vi "WVDIAL+HSRL_v1.0.vi"() -> ()   [LabVIEW 2012]
uses:
  C:/Users/H2ODial/Desktop/Shared Telescope WV DIAL Code/Libraries and VIs/PowerMeterCommands.dll
  Shared Telescope WV DIAL Code/Libraries and VIs/PowerMeterCommands.dll
  <vilib>/DAQmx/write.llb/DAQmx Write (Digital 1D Bool NChan 1Samp 1Line).vi
  <vilib>/DAQmx/miscellaneous.llb/DAQmx Fill In Error Info.vi
  <vilib>/Analysis/baseanly.llb/Mean (DBL).vi
  NCAR_DIAL_Labview/AMCS_Data.vi
  Libraries and VIs/Scalar_Data.vi
  <vilib>/Analysis/NI_AALBase.lvlib
  Libraries and VIs/Scalar_Data_2.vi
  Libraries and VIs/Scalar_Data_4.vi
  Libraries and VIs/Scalar_Data_3.vi
  Shared Telescope WV DIAL Code/bristol/CLDevIFace.dll
panel:
  out "FileHour":i32=21
  out "L_Count":i32=110
  out "background start":u32=534
  in  "Tab Control 2":enum32{"WV ND narrow", "WV ND wide"}(tab)=enum."WV ND wide"
  out "CH3 RingBuffer long":dbl[][](array[numeric])
  out "CH3 RingBuffer short":dbl[][](array[numeric])
  in  "?":T1(tab)
  out "NRB":dbl[][](graph) caption="Water Vapor Number Density"
  out "NRB 2":dbl[][](graph)=[[8.546195403591417e-05, 0.0002786584247195617, 0.0006090829121441516, 0.0011319761034550358, 0.001851230597986242, 0.002728257694582937, 0.003911345660657617, 0.005256523923123139, 0.006755425044654347, 0.008624773239187781, 0.010431137424772089, 0.012810234215426972, 0.015461219125224046, 0.018378218122423143, 0.02262031451514306, 0.02605089820013463, 0.03081964356661128, 0.03682776902972898, 0.04268026676965369, 0.050602630116497696, 0.058176055267544644, 0.06723475921094646, 0.07730364345829362, 0.08808311325248737, 0.10065736026541186, 0.1121183154362115, 0.12544132700380667, 0.1403937882704388, 0.15598356743521824, 0.17162511577051548, 0.18383704451264493, 0.19631841080771978, 0.21306952212863126, 0.22940462971855646, 0.24989138834202432, 0.26774391709096734, 0.28205876831659166, 0.3007676629703441, 0.31385204205047934, 0.33124784798609325, 0.3460233664658083, 0.35742760425188724, 0.3712840242876745, 0.3862720129999002, 0.39660375582269164, 0.40886228048361584, 0.4259284482749054, 0.440391338547647, 0.4566153688007287, 0.4717635460870204, 0.48207676553872175, 0.493753539302993, 0.5090591895240185, 0.5215880181755391, 0.533671261112484, 0.5420256236923419, 0.5530630628816117, 0.5689384508857108, 0.5752889942963373, 0.5875716528420664, 0.592552348222891, 0.5957528280323126, 0.60606140770504, 0.6165439786595378, 0.6287172140895222, 0.6342325225753401, 0.6490804275957623, 0.6524026888098357, 0.6569828232279292, 0.6692196293009464, 0.6831169256783645, 0.7013566860408543, 0.7100145647111005, 0.7160208275552816, 0.7118346778912209, 0.7144317674140145, 0.715945061880639, 0.7306883196013171, 0.7500440003241868, 0.7573606050746181, 0.7745392036058618, 0.7785022273472191, 0.7909248267167492, 0.8033782612939826, 0.8064196853129901, 0.8271538851971981, 0.8351575399099239, 0.8402193884447339, 0.8597133023547572, 0.8561064982936589, 0.8578435604795103, 0.8623534075092139, 0.8686671889614341, 0.8749972245828621, 0.8830530111544569, 0.909164243794476, 0.929038588425524, 0.9449513234760007, 0.957156632076746, 0.9643101360557969, 0.9596692122255749, 0.9545213343837654, 0.9805428317543672, 0.995047829667933, 1.029690672956509, 1.0674733507983893, 1.0955154176258788, 1.0951317989017593, 1.0974263194164438, 1.098780680310163, 1.0906771548016176, 1.1034601833969768, 1.1178136858913106, 1.1556491108545341, 1.170838831362434, 1.1937229570289496, 1.2185107373476831, 1.2369111498271113, 1.230561676484705, 1.2587157129408204, 1.258349691897498, 1.2643569689138991, 1.2850901805745287, 1.2890984172153068, 1.3232287209486395, 1.3179922411597433, 1.346817704187534, 1.3538431767650367, 1.3490196035262791, 1.3643175109856942, 1.357084592559015, 1.3735525179493822, 1.3720954670881582, 1.4069720445340057, 1.4377096932385625, 1.4667379965087042, 1.5062619180212748, 1.5283644930102516, 1.5354177107131104, 1.5563292232593602, 1.5684496791162663, 1.5568576568475363, 1.57314160663676, 1.5610280458417751, 1.581140399533629, 1.6296912525594276, 1.6562224982957428, 1.6957700702505019, 1.7149440773996392, 1.703831851733697, 1.7255160535134793, 1.7022433497624612, 1.7088135505273854, 1.7516190350709335, 1.798567492230373, 1.851955758886426, 1.8787729240747968, 1.9302841558592982, 1.9621318228338211, 1.9389378628727318, 1.9419926711108755, 1.9071918724993167, 1.8776863760152394, 1.8809405195258893, 1.9470314446188945, 1.9808515850130741, 2.0199051462386906, 2.111296178876415, 2.1153168527738186, 2.0968436639575736, 2.1412443186872054, 2.0756544478907495, 2.112753082434424, 2.1604416956610515, 2.1560867559085426, 2.239772997249097, 2.228779150280646, 2.263170685701022, 2.2168189161218668, 2.2129567210141583, 2.3490351617776835, 2.3904843802922366, 2.5153269519645782, 2.5634805908928726, 2.458644596909608, 2.4076529388828254, 2.431060203259, 2.487089848092278, 2.5385626161957418, 2.6534834782958736, 2.67324914118592, 2.6381061484328536, 2.659899097123786, 2.5932644861877714, 2.6291824330994853, 2.6989899250386693, 2.7424429265496375, 2.8488106986291943, 2.742279667999013, 2.725931661741348, 2.7773277260306966, 2.7669742901423433, 2.92714329948808, 2.9221494539127484, 2.950868194941447, 2.9730195868417186, 2.925221244719501, 3.0283229684289505, 3.045295843575443, 3.048386749915065, 2.9940537506089977, 2.999786519907248, 3.086225175965684, 3.0832975730831595, 3.1989694437550082, 3.243221406629081, 3.2005292303817927, 3.2510606719442636, 3.3383517491714887, 3.353440000926484, 3.3095989472229785, 3.410836647766328, 3.426518483197781, 3.5544093485967143, 3.796590326585979, 3.9752510583934777, 4.034684936991259, 3.941500910307474, 3.814794509432233, 3.614324384587308, 3.6283979364642334, 3.652682507305726, 3.6082445051935146, 3.757776325324033, 3.76070782445612, 3.8753962858175615, 3.832016308719547, 3.8070673373511394, 3.7482590130421487, 3.7356792789637026, 3.901429537689568, 3.9238044137388224, 3.981219962542532, 3.9581165639389835, 4.0440009093367, 3.9872219706905603, 4.074375676028611, 4.163939562811207, 4.109183162644875, 4.232130532448989, 4.32470565779948, 4.392875665538858, 4.419025834001803, 4.546703907908768, 4.6913520732902265, 5.095435948024424, 5.85033668191871, 6.948416991714669, 8.252360397367092, 9.704975333999297, 11.520408914991561, 13.322242925070737, 15.430932827011324, 17.759334108200914, 20.255853327839965, 23.129199142995606, 26.49310623037815, 30.317223286412915, 34.42247995845735, 38.843862293548, 42.96907001161705, 46.5351507877964, 49.700108765272844, 52.30595052176305, 54.66151784066439, 57.27473702687503, 59.76656578242474, 62.06676901244773, 64.07942162504204, 64.90714855474691, 64.57456805484065, 62.808310955515694, 59.961565043940276, 56.4288091190475, 52.44829418294068, 48.29155132434781, 44.122518735143416, 39.90135070569276, 35.95413315064079, 32.311788313192835, 28.664145828333695, 25.56822655944791, 22.593381127055597, 20.147311147330587, 18.37643667972368, 16.804539565374697, 15.544135239321264, 14.57019798472182, 13.511371779657093, 11.951556131001917, 10.556796376131562, 9.105859206777339, 7.636153114912772, 6.742182672366893, 5.884575550909214, 4.9120517923298905, 4.0816387293604155, 3.4251989306529906, 3.0755115887399, 2.992330865928349, 3.0592839009704034, 3.215509932991261, 3.164313441912157, 3.292078243733256, 3.3277022651481674, 3.4104950488283525, 3.6591380424661044, 3.6585893771087408, 3.645111765748741, 3.6040841077506585, 3.3942281204233713, 3.2723340521646254, 3.3042653495262546, 3.212298565962416, 3.2588896657794293, 3.412172206342532, 3.5365748913881014, 3.666044719857089, 3.6099922967500166, 3.5742002916165814, 3.3243040247393, 3.4802692620899798, 3.6002648864623774, 3.4946730738462572, 3.682551697278211, 3.534498028233769, 3.651838970885956, 3.6592843766152097, 3.5769786317282497, 3.831175889669123, 3.9537359381192307, 4.198205817594047, 4.292762449077934, 4.027917543935257, 3.86627577906732, 3.7390920401381775, 3.908518496471237, 3.9575314327457787, 4.045767179550537, 4.182182167113987, 4.319323821591138, 4.213359494616898, 3.9828552276172653, 3.9029181891931564, 3.8813083181843817, 4.124660793610378, 4.458753325246155, 4.484656167121237, 4.21569603752043, 4.398738645215913, 4.38977125517771, 4.486826719323201, 4.636388575777474, 4.721927541304717, 4.755068674711436, 4.678037042645568, 4.472456631914351, 4.437464950237424, 4.471292420670343, 4.635589244752503, 4.9756894692650535, 5.101888232883755, 5.196663320629597, 5.167081503628507, 4.932632838482907, 4.833721902386821, 4.920578756221176, 4.801799860414645, 4.982886632319263, 4.94287218541304, 4.7477113492626035, 5.053228596215403, 5.178145722278693, 5.251496618227864, 5.308182173096638, 5.126027314472312, 5.13158884387731, 5.245580767640445, 5.466282560232339, 5.520268417359091, 5.484994199187797, 5.440350102291734, 3.941060894744326, 2.540276340539141, 1.0752741992785009, -0.21371654449453512, -0.2535263616787527, -0.0215251722412666, 0.0736960393954925, -0.16074128741361193, -0.22026055992248075, -0.504917541914029, -0.5307574380992427, -0.5418672161900913, -0.5865574400501288, -0.47736616519198566, -0.17759619290122416, 0.025489947610103775, 0.12404732338561399, 0.5072486683987952, 0.1854880266358113, 0.26600693173218026, 0.37269308072518276, -0.06214751635724484, 0.16109730035647882, 0.19961295131033274, 0.16054713331939102, 0.3723968795809794, 0.13049120350027968, -0.17385934990265337, -0.21640202606490286, -0.48491744291793354, -0.3516048206810621, -0.5452074651121137, -0.6640463986814213, -0.5148790831917176, -0.5996424436961612, -0.3675738486958148, -0.24413197824721797, -0.31118451234206884, -0.451177199999366, -0.5872883257360875, -0.35674585539839615, -0.19314012538700928, 0.0021220489657220276, 0.21466183565900696, 0.09269836459999599, 0.17646046148922798, 0.056526565682545306, 0.24408390632204388, 0.07252540455404405, -0.02181420421509619, 0.10205416135256055, -0.09331498102145104, -0.07214578665686074, 0.1846866976108202, 0.5635053691699698, 0.5309428402635872, 0.5350604832036495, 0.5511159858985675, 0.39021559281953083, 0.5019216998108322, 0.8010907973716676, 0.1820967880098238, 0.2516937332550209, 0.13548174860232123, 0.003426436422801223, 0.5498271763579102, 0.3017178427483544, 0.30779490101395435, 0.3194336031664126, 0.14682798732272256, 0.35782941193936996, 0.21703523756214044, 0.1580964681743854, 0.26852071324119886, 0.06585437268575421, 0.25225607116669657, -0.0987900349022226, -0.2865272113485497, -0.23476975121469307, -0.3714731517059426, -0.2623208170135795, -0.9814932822860765, -1.0578589256565503, -0.6479324108525774, -0.5427806071790823, 0.20541712714675675, 0.19515889423177873, -0.29526119720445787, -0.472252091600822, -0.6651737975799542, -0.6186882389312311, -0.369116926064781, -0.3690155725472422, -0.38647936731578586, -0.0950262543059411, -0.03854286960600729, 0.30726911813041896, 0.4651921643385956, 0.6978446374004414, 1.0103301505079703, 1.1579083835337383, 1.3873538039368287, 0.4157864001006136, 0.6469789390673985, 0.5046572410534047, 0.26932256080595396, 0.5819929290496607, -0.026184210530850176, -0.5210278980359441, -0.5218016986678393, -0.09830787683363085, 0.10527780250099723, 0.4203966150447178, 0.43890253055010187, 0.14924195872471907, 0.49017086714906183, 0.7979315186565493, 0.9509911782214592, 1.060490580096141, 0.7547309430188422, 0.5481496744565173, 0.6572918231669737, 0.7080537983862634, 0.32232225319211155, 0.16999017226614138, -0.2027014179632393, -0.6150725603001224, -0.6127660288641613, -0.5963368434638746, -0.6377635713973827, -0.3022504867219528, 0.020185972398814287, 0.1271130821329239, 0.4991850715558948, 0.6693287614761402, 0.32397832728321585, 0.31794176368996296, 0.10669714138882108, -0.03197152766302852, 0.4185465993184435, 0.5081345035389131, 0.11472933106232114, -0.335101659818229, -0.7236369378617327, -1.0696346854599716, -0.7595991284525778, -0.4130296018032728, -0.4655290854617895, -0.1709578789784718, 0.35155527912355344, 0.49114775107992503, 0.670181627376166, 0.7230296930330916, 0.5770818030588206, 0.281430213436321, -0.15202417316952307, -0.5672339141806462, -0.784440563139071, -0.42794760098036877, 0.31191170275899854, 0.8830921349838413, 0.7115149103111856, 0.3440988921429906, 0.0, 0.0, 0.0, 0.0, 0.0]] caption="Water Vapor Number Density"
  out "CH 1 (WV off) counts display":dbl[][](graph) caption="Water Vapor Number Density"
  out "CH 3 (HSRL comb) counts display":dbl[][](graph)=[[105.35999999999967, 41.35999999999967, -21.640000000000327, 29.359999999999673, 89.35999999999967, -127.64000000000033, -119.64000000000033, 47.35999999999967, 53.35999999999967, -15.640000000000327, 82.35999999999967, 114.35999999999967, 141.35999999999967, -22.640000000000327, 130.35999999999967, 185.35999999999967, 154.35999999999967, 75.35999999999967, -42.64000000000033, 5.359999999999673, 129.35999999999967, 243.35999999999967, 192.35999999999967, 97.35999999999967, 206.35999999999967, 154.35999999999967, 301.3599999999997, 341.3599999999997, 187.35999999999967, 197.35999999999967, 384.3599999999997, 184.35999999999967, 331.3599999999997, 200.35999999999967, 183.35999999999967, 294.3599999999997, 307.3599999999997, 439.3599999999997, 415.3599999999997, 322.3599999999997, 367.3599999999997, 213.35999999999967, 366.3599999999997, 322.3599999999997, 197.35999999999967, 229.35999999999967, 264.3599999999997, 295.3599999999997, 196.35999999999967, 156.35999999999967, 205.35999999999967, 277.3599999999997, 294.3599999999997, 374.3599999999997, 277.3599999999997, 287.3599999999997, 132.35999999999967, 356.3599999999997, 275.3599999999997, 290.3599999999997, 272.3599999999997, 144.35999999999967, 185.35999999999967, 197.35999999999967, 246.35999999999967, 226.35999999999967, 185.35999999999967, 297.3599999999997, 214.35999999999967, 153.35999999999967, 159.35999999999967, 218.35999999999967, 42.35999999999967, 137.35999999999967, 88.35999999999967, 100.35999999999967, 96.35999999999967, 161.35999999999967, 102.35999999999967, 162.35999999999967, 23.359999999999673, 151.35999999999967, 171.35999999999967, 188.35999999999967, -84.64000000000033, 31.359999999999673, -26.640000000000327, 74.35999999999967, 93.35999999999967, 41.35999999999967, 17.359999999999673, -6.640000000000327, 148.35999999999967, 159.35999999999967, 33.35999999999967, 75.35999999999967, 50.35999999999967, 132.35999999999967, 43.35999999999967, 32.35999999999967, 52.35999999999967, 100.35999999999967, 1.3599999999996726, -25.640000000000327, -48.64000000000033, 80.35999999999967, -81.64000000000033, -28.640000000000327, -92.64000000000033, 70.35999999999967, 117.35999999999967, -4.640000000000327, 15.359999999999673, 36.35999999999967, 30.359999999999673, 136.35999999999967, 79.35999999999967, 103.35999999999967, 27.359999999999673, -65.64000000000033, 156.35999999999967, -72.64000000000033, 26.359999999999673, 9.359999999999673, -6.640000000000327, -48.64000000000033, 46.35999999999967, 103.35999999999967, 19.359999999999673, 80.35999999999967, -169.64000000000033, 94.35999999999967, 41.35999999999967, -86.64000000000033, -10.640000000000327, -41.64000000000033, 66.35999999999967, 74.35999999999967, 87.35999999999967, -17.640000000000327, -3.6400000000003274, -58.64000000000033, 46.35999999999967, 21.359999999999673, -12.640000000000327, -50.64000000000033, 45.35999999999967, 83.35999999999967, 152.35999999999967, -69.64000000000033, 4.359999999999673, 62.35999999999967, -40.64000000000033, -53.64000000000033, -50.64000000000033, -33.64000000000033, 38.35999999999967, -10.640000000000327, -1.6400000000003274, -7.640000000000327, -4.640000000000327, -59.64000000000033, -49.64000000000033, 60.35999999999967, 34.35999999999967, -143.64000000000033, -104.64000000000033, -59.64000000000033, 2.3599999999996726, -100.64000000000033, -3.6400000000003274, -54.64000000000033, 42.35999999999967, 135.35999999999967, -10.640000000000327, 3.3599999999996726, -6.640000000000327, -79.64000000000033, -117.64000000000033, 42.35999999999967, 90.35999999999967, -73.64000000000033, 161.35999999999967, 79.35999999999967, 41.35999999999967, -52.64000000000033, 61.35999999999967, 9.359999999999673, -10.640000000000327, -164.64000000000033, 103.35999999999967, -89.64000000000033, -32.64000000000033, 31.359999999999673, 41.35999999999967, 42.35999999999967, -68.64000000000033, 58.35999999999967, 8.359999999999673, 28.359999999999673, 37.35999999999967, -19.640000000000327, 39.35999999999967, 49.35999999999967, 9.359999999999673, 73.35999999999967, -105.64000000000033, -9.640000000000327, -171.64000000000033, -56.64000000000033, -17.640000000000327, 64.35999999999967, -50.64000000000033, -115.64000000000033, -48.64000000000033, 110.35999999999967, 79.35999999999967, -127.64000000000033, -117.64000000000033, -70.64000000000033, 46.35999999999967, -88.64000000000033, 65.35999999999967, -31.640000000000327, -32.64000000000033, -81.64000000000033, -12.640000000000327, -6.640000000000327, -25.640000000000327, -163.64000000000033, -7.640000000000327, 1.3599999999996726, -48.64000000000033, 67.35999999999967, -11.640000000000327, -14.640000000000327, 110.35999999999967, -35.64000000000033, 40.35999999999967, -34.64000000000033, -28.640000000000327, 25.359999999999673, -24.640000000000327, 32.35999999999967, 21.359999999999673, 32.35999999999967, -47.64000000000033, -158.64000000000033, -48.64000000000033, -19.640000000000327, 28.359999999999673, -32.64000000000033, 100.35999999999967, 0.3599999999996726, -58.64000000000033, 126.35999999999967, 39.35999999999967, -102.64000000000033, 45.35999999999967, 269.3599999999997, 248.35999999999967, 370.3599999999997, 551.3599999999997, 698.3599999999997, 743.3599999999997, 888.3599999999997, 1103.3599999999997, 1108.3599999999997, 1096.3599999999997, 1212.3599999999997, 1501.3599999999997, 1609.3599999999997, 1851.3599999999997, 1948.3599999999997, 1879.3599999999997, 1926.3599999999997, 1860.3599999999997, 2027.3599999999997, 1776.3599999999997, 1865.3599999999997, 1711.3599999999997, 1508.3599999999997, 1453.3599999999997, 1241.3599999999997, 1175.3599999999997, 1037.3599999999997, 924.3599999999997, 842.3599999999997, 875.3599999999997, 788.3599999999997, 727.3599999999997, 587.3599999999997, 441.3599999999997, 474.3599999999997, 404.3599999999997, 352.3599999999997, 329.3599999999997, 267.3599999999997, 205.35999999999967, 308.3599999999997, 160.35999999999967, 187.35999999999967, 146.35999999999967, 142.35999999999967, 175.35999999999967, 88.35999999999967, -74.64000000000033, 80.35999999999967, 42.35999999999967, -150.64000000000033, 30.359999999999673, -1.6400000000003274, -68.64000000000033, -65.64000000000033, 23.359999999999673, -22.640000000000327, -42.64000000000033, -84.64000000000033, -35.64000000000033, 64.35999999999967, -91.64000000000033, -36.64000000000033, -47.64000000000033, -135.64000000000033, -22.640000000000327, -123.64000000000033, 65.35999999999967, 50.35999999999967, -64.64000000000033, 13.359999999999673, 80.35999999999967, -85.64000000000033, -167.64000000000033, 13.359999999999673, 13.359999999999673, 82.35999999999967, 5.359999999999673, -0.6400000000003274, 96.35999999999967, -23.640000000000327, 49.35999999999967, -19.640000000000327, 36.35999999999967, 20.359999999999673, -70.64000000000033, -45.64000000000033, -40.64000000000033, -15.640000000000327, 7.359999999999673, -54.64000000000033, 56.35999999999967, 132.35999999999967, -0.6400000000003274, 106.35999999999967, -140.64000000000033, 54.35999999999967, -45.64000000000033, -20.640000000000327, -17.640000000000327, -74.64000000000033, 34.35999999999967, 19.359999999999673, 63.35999999999967, 43.35999999999967, 39.35999999999967, 17.359999999999673, -64.64000000000033, -58.64000000000033, 92.35999999999967, -40.64000000000033, 2.3599999999996726, 67.35999999999967, -34.64000000000033, 78.35999999999967, -14.640000000000327, -74.64000000000033, -30.640000000000327, 115.35999999999967, -34.64000000000033, -0.6400000000003274, -98.64000000000033, -52.64000000000033, -39.64000000000033, 42.35999999999967, 71.35999999999967, -8.640000000000327, 63.35999999999967, 61.35999999999967, -25.640000000000327, -98.64000000000033, -25.640000000000327, 4.359999999999673, 47.35999999999967, 155.35999999999967, 39.35999999999967, 70.35999999999967, -117.64000000000033, -26.640000000000327, -37.64000000000033, 0.3599999999996726, 2.3599999999996726, 109.35999999999967, -105.64000000000033, 88.35999999999967, -19.640000000000327, 51.35999999999967, -24.640000000000327, -84.64000000000033, 16.359999999999673, -44.64000000000033, 65.35999999999967, -39.64000000000033, 82.35999999999967, -63.64000000000033, 30.359999999999673, 36.35999999999967, 53.35999999999967, -33.64000000000033, 87.35999999999967, 131.35999999999967, 18.359999999999673, -67.64000000000033, 13.359999999999673, 67.35999999999967, -17.640000000000327, -1.6400000000003274, -44.64000000000033, 17.359999999999673, -34.64000000000033, -16.640000000000327, 49.35999999999967, 22.359999999999673, 69.35999999999967, -77.64000000000033, -6.640000000000327, 44.35999999999967, -24.640000000000327, 33.35999999999967, 33.35999999999967, -65.64000000000033, 96.35999999999967, -102.64000000000033, 57.35999999999967, 94.35999999999967, -95.64000000000033, -29.640000000000327, -88.64000000000033, -49.64000000000033, 168.35999999999967, -35.64000000000033, 10.359999999999673, -73.64000000000033, -84.64000000000033, -99.64000000000033, -39.64000000000033, -109.64000000000033, -51.64000000000033, 10.359999999999673, 52.35999999999967, -49.64000000000033, 10.359999999999673, -51.64000000000033, -6.640000000000327, 45.35999999999967, 60.35999999999967, -24.640000000000327, 29.359999999999673, 78.35999999999967, 4.359999999999673, 132.35999999999967, 13.359999999999673, -92.64000000000033, -52.64000000000033, 58.35999999999967, 30.359999999999673, -60.64000000000033, -135.64000000000033, 63.35999999999967, 8.359999999999673, 56.35999999999967, -60.64000000000033, 10.359999999999673, 30.359999999999673, -73.64000000000033, -37.64000000000033, 53.35999999999967, -18.640000000000327, -28.640000000000327, 52.35999999999967, 137.35999999999967, 53.35999999999967, 44.35999999999967, 96.35999999999967, 65.35999999999967, -82.64000000000033, -126.64000000000033, 10.359999999999673, -11.640000000000327, 21.359999999999673, 22.359999999999673, 51.35999999999967, -16.640000000000327, 51.35999999999967, 11.359999999999673, -53.64000000000033, 107.35999999999967, 109.35999999999967, -7.640000000000327, -50.64000000000033, -91.64000000000033, 40.35999999999967, 11.359999999999673, -44.64000000000033, 25.359999999999673, 80.35999999999967, 52.35999999999967, 88.35999999999967, 36.35999999999967, 89.35999999999967, 37.35999999999967, -136.64000000000033, 29.359999999999673, 57.35999999999967, 111.35999999999967, -102.64000000000033, 60.35999999999967, -92.64000000000033, 12.359999999999673, -63.64000000000033, 34.35999999999967, -151.64000000000033, -0.6400000000003274, 40.35999999999967, 142.35999999999967, 72.35999999999967, 40.35999999999967, 65.35999999999967, 29.359999999999673, -178.64000000000033, -44.64000000000033, -2.6400000000003274, 36.35999999999967, 20.359999999999673, -24.640000000000327, 34.35999999999967, -46.64000000000033, 0.3599999999996726, -38.64000000000033, -34.64000000000033, 10.359999999999673, 105.35999999999967, -24.640000000000327, 46.35999999999967, 59.35999999999967, -81.64000000000033, 51.35999999999967, -115.64000000000033, 16.359999999999673, 4.359999999999673, 0.0]] caption="Water Vapor Number Density"
  out "CH3 (HSRL combined) smooth S":dbl[](array[numeric])=[205.29783333333336, 167.4186666666667, 162.64783333333338, 170.01866666666672, 177.9353333333334, 182.0978333333334, 191.7811666666667, 197.3186666666667, 200.35616666666672, 207.1811666666667, 207.08533333333338, 213.6811666666667, 219.73533333333336, 225.1978333333334, 241.41033333333337, 244.34783333333334, 256.03533333333337, 272.84783333333337, 283.7645, 303.5686666666667, 316.51033333333334, 333.2353333333333, 350.4811666666666, 366.7019999999999, 386.11449999999996, 397.58116666666666, 412.4186666666667, 429.1186666666667, 444.3811666666667, 456.827, 458.2644999999999, 459.26449999999994, 468.65199999999993, 475.3019999999999, 488.5144999999999, 494.7061666666666, 493.37283333333323, 498.74366666666657, 494.11866666666657, 495.7478333333333, 492.92283333333324, 485.2519999999999, 480.9144999999999, 477.86033333333324, 469.12283333333323, 462.85616666666664, 461.88116666666656, 457.8936666666666, 455.5936666666666, 452.08533333333327, 444.0686666666667, 437.53116666666665, 434.24783333333335, 428.6353333333334, 422.7895000000001, 414.24783333333335, 408.0103333333334, 405.3853333333334, 396.17283333333336, 391.27699999999993, 381.802, 371.62283333333335, 366.16866666666664, 360.97283333333337, 356.87699999999995, 349.2103333333333, 346.8061666666666, 338.4353333333333, 331.03116666666665, 327.6436666666666, 325.102, 324.577, 319.6603333333333, 313.73116666666664, 303.6686666666667, 296.83116666666666, 289.8061666666666, 288.2436666666667, 288.43533333333335, 284.02700000000004, 283.34366666666665, 277.90616666666665, 275.5853333333334, 273.3061666666667, 267.9395, 268.47283333333337, 264.88533333333334, 260.4811666666667, 260.56866666666673, 253.76033333333336, 248.7311666666667, 244.64366666666672, 241.17283333333336, 237.7978333333334, 234.9686666666667, 236.89783333333338, 237.1103333333334, 236.27700000000004, 234.52283333333338, 231.58116666666672, 225.93950000000004, 220.35616666666672, 221.9853333333334, 220.96033333333338, 224.31033333333338, 228.16450000000003, 229.79783333333336, 225.4936666666667, 221.84783333333337, 218.11033333333336, 212.6311666666667, 211.30200000000005, 210.2811666666667, 213.5936666666667, 212.65616666666673, 213.08950000000004, 213.81033333333338, 213.37700000000007, 208.73950000000002, 209.9686666666667, 206.46033333333338, 204.06450000000004, 204.05200000000005, 201.4061666666667, 203.43950000000007, 199.43950000000004, 200.60200000000003, 198.51450000000003, 194.7603333333334, 193.95200000000003, 189.99783333333335, 189.40200000000004, 186.3728333333334, 188.26450000000006, 189.53533333333337, 190.52700000000004, 192.8103333333334, 192.81450000000007, 190.9311666666667, 190.77700000000004, 189.5478333333334, 185.51450000000006, 184.8436666666667, 180.88950000000006, 180.70200000000003, 183.70200000000006, 184.16033333333337, 186.01450000000006, 185.60200000000003, 181.95616666666672, 181.83950000000004, 177.0436666666667, 175.41450000000006, 177.47700000000006, 179.8853333333334, 182.85200000000006, 183.1436666666667, 185.78533333333337, 186.4811666666667, 181.98950000000005, 180.02283333333335, 174.6311666666667, 169.83533333333338, 168.06450000000004, 171.8603333333334, 172.7436666666667, 174.04366666666672, 179.74783333333338, 177.9686666666667, 174.35200000000003, 175.96450000000004, 168.61033333333336, 169.64366666666672, 171.4811666666667, 169.18950000000004, 173.7561666666667, 170.96033333333338, 171.65200000000004, 166.27283333333338, 164.14783333333338, 172.3061666666667, 173.4228333333334, 180.47700000000006, 181.9353333333334, 172.63116666666673, 167.24783333333338, 167.0728333333334, 169.10616666666672, 170.7811666666667, 176.62700000000004, 176.08533333333338, 171.97283333333337, 171.60200000000003, 165.5936666666667, 166.16866666666672, 168.83950000000004, 169.8186666666667, 174.6186666666667, 166.4186666666667, 163.7811666666667, 165.21033333333338, 162.97283333333337, 170.6978333333334, 168.7436666666667, 168.74366666666674, 168.36450000000005, 164.0686666666667, 168.21450000000004, 167.5436666666667, 166.12283333333338, 161.62700000000004, 160.41450000000003, 163.4853333333334, 161.81033333333335, 166.31450000000004, 167.0561666666667, 163.34783333333337, 164.4061666666667, 167.27700000000004, 166.5103333333334, 162.85616666666672, 166.32283333333336, 165.5936666666667, 170.23533333333336, 180.20200000000006, 187.00200000000004, 188.12700000000004, 182.18533333333338, 174.80616666666668, 164.20200000000006, 163.41866666666672, 163.09783333333337, 159.73950000000005, 164.9311666666667, 163.66033333333337, 167.2186666666667, 163.96033333333338, 161.5311666666667, 157.71450000000004, 155.88116666666673, 161.43950000000004, 161.02700000000004, 162.03950000000006, 159.78533333333337, 161.9186666666667, 158.35616666666672, 160.50616666666673, 162.71033333333338, 159.28950000000003, 162.73950000000005, 164.97283333333337, 166.2436666666667, 165.91450000000006, 169.3603333333334, 173.37283333333338, 186.81033333333338, 212.7603333333334, 250.63533333333336, 295.2311666666667, 344.34783333333337, 405.3645, 464.8895, 533.9811666666666, 609.4019999999999, 689.2269999999999, 780.3061666666665, 886.0769999999999, 1005.1020000000001, 1131.156166666667, 1265.131166666667, 1387.2978333333338, 1489.7103333333337, 1577.847833333334, 1647.206166666667, 1707.7395000000006, 1775.106166666667, 1837.7020000000005, 1893.543666666667, 1939.9520000000005, 1950.7645000000002, 1927.4811666666671, 1862.8311666666668, 1767.7270000000008, 1653.9770000000003, 1528.6645000000005, 1399.6895000000004, 1271.7603333333336, 1143.7395000000004, 1024.8228333333336, 915.7645, 807.7728333333333, 716.3228333333333, 629.2686666666666, 557.7686666666666, 505.58949999999993, 459.4561666666666, 422.3103333333333, 393.3228333333333, 362.427, 318.6061666666667, 279.677, 239.74783333333335, 199.81450000000007, 175.3103333333334, 152.0478333333334, 126.12700000000005, 104.1478333333334, 86.8478333333334, 77.48533333333339, 74.90616666666673, 76.08950000000007, 79.4603333333334, 77.69783333333339, 80.31866666666673, 80.6728333333334, 82.15616666666673, 87.5853333333334, 87.02283333333341, 86.1603333333334, 84.6603333333334, 79.23950000000006, 75.92283333333339, 76.18950000000005, 73.61450000000006, 74.22283333333338, 77.23533333333339, 79.56033333333339, 81.96866666666673, 80.22700000000006, 78.95200000000006, 72.99366666666671, 75.95616666666672, 78.10200000000006, 75.3603333333334, 78.93533333333339, 75.31450000000007, 77.35200000000006, 77.05200000000006, 74.87700000000005, 79.7228333333334, 81.78950000000006, 86.33533333333338, 87.76450000000006, 81.87700000000005, 78.13950000000006, 75.13533333333339, 78.08533333333338, 78.61033333333339, 79.90200000000006, 82.1228333333334, 84.33116666666672, 81.79783333333339, 76.88950000000006, 74.92283333333339, 74.08950000000006, 78.28950000000006, 84.15200000000006, 84.16866666666674, 78.6853333333334, 81.64366666666672, 81.02700000000006, 82.36033333333339, 84.63533333333339, 85.7228333333334, 85.85200000000006, 84.00200000000007, 79.87700000000007, 78.82283333333339, 78.99366666666671, 81.45200000000006, 86.95200000000006, 88.67700000000006, 89.83950000000006, 88.85200000000006, 84.3728333333334, 82.24366666666673, 83.27700000000006, 80.83950000000006, 83.44366666666673, 82.33950000000006, 78.67700000000006, 83.29783333333339, 84.9103333333334, 85.66450000000006, 86.13950000000006, 82.75616666666673, 82.41866666666674, 83.81450000000007, 86.88950000000007, 87.2978333333334, 86.2978333333334, 85.1603333333334, 61.39366666666673, 39.381166666666736, 16.589500000000058, -3.281333333333275, -3.8729999999999416, -0.32716666666660776, 1.1145000000000589, -2.4188333333332745, -3.2979999999999414, -7.522999999999941, -7.868833333333274, -7.993833333333274, -8.610499999999941, -6.97299999999994, -2.5813333333332737, 0.36866666666672543, 1.785333333333392, 7.264500000000059, 2.6436666666667255, 3.7728333333333923, 5.260333333333392, -0.872999999999941, 2.2520000000000593, 2.7770000000000588, 2.222833333333392, 5.131166666666726, 1.7895000000000585, -2.3729999999999416, -2.939666666666608, -6.556333333333274, -4.731333333333275, -7.302166666666608, -8.852166666666607, -6.831333333333275, -7.918833333333274, -4.831333333333275, -3.1938333333332745, -4.052166666666608, -5.847999999999941, -7.577166666666608, -4.581333333333275, -2.4688333333332744, 0.02700000000005842, 2.718666666666725, 1.1686666666667254, 2.2145000000000588, 0.7061666666667255, 3.035333333333392, 0.8978333333333921, -0.26883333333327464, 1.2520000000000588, -1.1396666666666078, -0.8771666666666079, 2.2353333333333922, 6.789500000000059, 6.3686666666667255, 6.3895000000000595, 6.552000000000059, 4.6186666666667255, 5.914500000000059, 9.397833333333391, 2.127000000000059, 2.927000000000059, 1.5686666666667257, 0.03950000000005893, 6.310333333333393, 3.447833333333392, 3.502000000000059, 3.6186666666667255, 1.6561666666667256, 4.018666666666726, 2.4270000000000587, 1.7603333333333924, 2.977000000000059, 0.7270000000000585, 2.7728333333333923, -1.0813333333332746, -3.122999999999941, -2.5479999999999414, -4.014666666666608, -2.8229999999999413, -10.518833333333275, -11.289666666666609, -6.885499999999942, -5.743833333333274, 2.164500000000059, 2.0478333333333922, -3.085499999999941, -4.914666666666608, -6.893833333333275, -6.385499999999942, -3.793833333333274, -3.7771666666666075, -3.9396666666666076, -0.964666666666607, -0.389666666666608, 3.0936666666667256, 4.664500000000059, 6.968666666666726, 10.047833333333394, 11.468666666666726, 13.685333333333391, 4.085333333333393, 6.331166666666727, 4.918666666666726, 2.6145000000000596, 5.627000000000059, -0.2521666666666079, -4.997999999999942, -4.985499999999941, -0.9354999999999412, 0.9978333333333924, 3.968666666666725, 4.127000000000059, 1.397833333333392, 4.572833333333392, 7.414500000000059, 8.802000000000058, 9.777000000000058, 6.9311666666667255, 5.014500000000059, 5.989500000000058, 6.427000000000059, 2.914500000000059, 1.5311666666667252, -1.8188333333332745, -5.497999999999941, -5.456333333333274, -5.289666666666609, -5.635499999999942, -2.6604999999999412, 0.17700000000005867, 1.110333333333392, 4.343666666666726, 5.802000000000058, 2.797833333333392, 2.7353333333333922, 0.9145000000000589, -0.2729999999999413, 3.560333333333392, 4.3061666666667255, 0.9686666666667256, -2.8188333333332745, -6.064666666666607, -8.931333333333274, -6.318833333333275, -3.4229999999999414, -3.843833333333275, -1.4063333333332746, 2.8811666666667257, 4.010333333333392, 5.452000000000059, 5.860333333333393, 4.6603333333333925, 2.2645000000000586, -1.2188333333332744, -4.531333333333275, -6.243833333333274, -3.393833333333275, 2.4645000000000583, 6.952000000000059, 5.581166666666725, 2.689500000000059]
  out "CH3 (HSRL combined) smooth L":dbl[](array[numeric])=[66.7708561643836, 29.338493150684968, 27.07393835616442, 32.525993150684975, 36.934383561643884, 40.63815068493156, 46.37873287671238, 48.601335616438405, 53.01743150684937, 59.80595890410964, 64.68438356164387, 71.85047945205483, 77.13900684931511, 82.96606164383564, 90.89414383561648, 98.40869863013702, 107.58078767123291, 118.46948630136993, 127.8898630136987, 139.92496575342471, 150.56965753424666, 164.39328767123294, 178.45150684931514, 191.23318493150688, 206.85390410958908, 219.08250000000004, 230.7408904109589, 241.09020547945207, 249.3325, 255.5533904109589, 261.32821917808224, 265.47547945205486, 271.20578767123294, 274.0191438356165, 276.65184931506855, 279.08678082191784, 279.11332191780826, 281.9241095890411, 280.16469178082195, 277.30253424657536, 274.033698630137, 268.9977397260274, 267.6355821917808, 264.4472260273973, 260.9686301369863, 258.0311301369863, 253.527705479452, 251.86160958904105, 248.24260273972598, 245.44808219178083, 241.65784246575345, 235.7862671232877, 233.76828767123294, 230.248595890411, 224.76229452054798, 224.43010273972607, 218.75715753424657, 214.24517123287674, 211.05938356164387, 204.18523972602742, 199.68095890410962, 194.1544178082192, 189.80510273972604, 185.13986301369866, 182.32565068493153, 178.3222260273973, 176.3984246575343, 174.19808219178088, 170.36417808219187, 168.71691780821925, 165.5439726027398, 163.28455479452063, 158.77342465753435, 154.68695205479463, 148.17496575342474, 143.6424315068494, 139.37530821917815, 135.8453424657535, 133.6758219178083, 129.1176027397261, 127.93095890410969, 124.23660958904118, 121.9523630136987, 120.0011643835617, 116.52941780821922, 114.94722602739729, 111.11845890410962, 108.91811643835618, 106.56794520547948, 103.07821917808222, 100.70921232876715, 97.24174657534249, 93.12616438356167, 89.21263698630139, 87.24602739726029, 85.67582191780824, 87.35904109589043, 88.14500000000002, 85.17924657534249, 84.59106164383564, 79.87273972602742, 77.44808219178086, 77.98832191780825, 76.54397260273977, 77.02684931506855, 75.34106164383566, 73.75202054794524, 72.58934931506853, 71.998595890411, 71.19037671232881, 71.13986301369867, 68.47291095890415, 67.35476027397264, 68.4943150684932, 67.06023972602743, 67.36417808219181, 67.67667808219181, 66.85390410958908, 65.80339041095894, 64.14414383561648, 62.686095890410996, 60.28712328767127, 58.16469178082196, 58.79482876712333, 57.4831849315069, 55.38986301369868, 58.65613013698635, 57.882157534246616, 55.585924657534285, 57.461780821917856, 53.57222602739731, 51.45321917808224, 53.16297945205485, 51.13130136986307, 51.154417808219236, 51.564520547945264, 50.0234246575343, 51.44465753424663, 51.35304794520553, 53.2040753424658, 53.88130136986306, 51.49345890410964, 50.77513698630142, 47.26143835616443, 45.38130136986307, 45.83592465753429, 44.430102739726074, 43.724623287671285, 45.371883561643884, 44.65869863013704, 46.24773972602745, 46.37530821917813, 43.94380136986307, 42.94380136986307, 42.432671232876764, 43.35304794520553, 43.40099315068499, 44.47804794520553, 44.06537671232882, 42.495171232876764, 41.4831849315069, 40.044828767123335, 37.964349315068546, 37.22291095890416, 37.91297945205484, 38.663835616438405, 39.210068493150736, 40.69208904109594, 39.31023972602745, 36.611609589041144, 37.669828767123335, 35.62445205479457, 37.46349315068498, 40.07565068493156, 40.1552739726028, 40.547397260274025, 38.96349315068498, 38.01058219178087, 36.455787671232926, 35.89500000000005, 39.04825342465759, 39.060239726027454, 39.11674657534252, 39.44037671232882, 35.90099315068498, 34.69123287671238, 35.705787671232926, 36.374452054794574, 38.39414383561649, 40.94465753424663, 40.83421232876717, 39.01143835616443, 36.84791095890416, 35.11503424657539, 34.871883561643884, 35.9943150684932, 35.086780821917856, 34.69208904109594, 33.95236301369867, 33.924109589041144, 35.7956849315069, 36.091061643835666, 37.342773972602785, 37.08849315068498, 36.759726027397306, 36.15613013698635, 33.67924657534252, 32.87102739726032, 32.41041095890416, 30.936095890411003, 30.56280821917813, 30.728047945205525, 30.72119863013703, 33.053390410958954, 33.651849315068546, 33.40869863013704, 33.30082191780827, 32.178390410958954, 32.832500000000046, 30.851335616438405, 32.87102739726032, 33.15955479452059, 32.396712328767165, 36.55167808219183, 36.07393835616443, 38.32308219178087, 40.11417808219183, 39.17410958904115, 38.07308219178087, 33.70065068493155, 32.784554794520595, 31.716061643835666, 33.711780821917856, 37.49773972602745, 35.40356164383566, 38.35904109589046, 35.806815068493194, 32.927534246575384, 35.25116438356169, 31.55167808219182, 29.599623287671264, 29.97890410958908, 28.101335616438394, 28.119315068493194, 30.059383561643884, 29.97291095890416, 31.27085616438361, 31.316232876712377, 29.05595890410963, 27.22890410958908, 26.71263698630141, 26.070513698630172, 26.93095890410963, 30.148424657534292, 32.5679452054795, 36.97547945205484, 46.992602739726074, 59.19380136986307, 74.7708561643836, 94.94722602739728, 118.67154109589043, 144.4198287671233, 178.93438356164387, 223.96434931506855, 278.49174657534246, 345.2597260273972, 420.70493150684933, 499.61160958904134, 584.1758219178087, 674.1039041095894, 766.4634931506853, 863.6852397260275, 969.3051027397257, 1072.3342123287666, 1164.0431164383554, 1233.269999999999, 1259.1355821917798, 1249.4515068493142, 1207.254589041095, 1145.3290753424649, 1080.1655479452047, 1020.2074999999993, 977.5722260273967, 950.9472260273968, 931.3076712328764, 906.8787328767121, 869.6535616438355, 811.1167465753423, 738.9583561643835, 662.1176027397261, 580.9309589041097, 506.5217123287673, 441.8316438356166, 387.40955479452066, 350.3547602739727, 327.6869520547947, 315.22034246575356, 311.4806164383563, 304.1501369863015, 289.15527397260286, 269.9215410958905, 241.81109589041108, 212.1895205479453, 185.879589041096, 156.0020205479453, 128.58335616438362, 105.81708904109591, 84.07479452054797, 65.87445205479456, 50.30767123287676, 35.27941780821922, 25.46349315068497, 16.228904109589074, 14.912123287671267, 13.84705479452058, 12.753732876712363, 15.649280821917843, 14.484897260274005, 12.017431506849348, 9.475479452054827, 9.344486301369898, 8.208356164383595, 9.04397260273976, 11.584212328767158, 10.145000000000035, 10.091917808219211, 12.083356164383595, 11.454931506849348, 10.009726027397294, 10.331643835616472, 7.4506506849315395, 7.063664383561678, 10.73147260273976, 9.781130136986334, 10.886438356164417, 9.94551369863017, 9.694657534246609, 9.465205479452088, 9.936952054794554, 10.672397260274007, 9.538835616438389, 11.349623287671266, 11.436095890410991, 12.168116438356197, 12.527705479452088, 11.691232876712363, 12.59534246575346, 9.604760273972637, 9.693801369863047, 10.828219178082225, 12.124452054794553, 13.721198630137017, 13.963493150684965, 12.89842465753428, 11.330787671232912, 13.158698630137021, 13.87702054794524, 13.22633561643839, 12.628732876712364, 13.877876712328803, 13.057671232876746, 14.936095890410991, 15.942945205479486, 16.05339041095894, 16.921541095890447, 17.01143835616442, 16.536267123287708, 15.105616438356197, 14.6681164383562, 13.060239726027433, 14.109897260274007, 14.29397260273976, 14.78455479452058, 16.22547945205483, 15.688664383561678, 15.905273972602775, 15.677534246575377, 14.531130136986336, 14.480616438356197, 14.124452054794554, 12.73232876712332, 13.222910958904142, 12.18438356164387, 11.807671232876745, 12.418116438356197, 12.839349315068528, 13.843630136986338, 14.685239726027433, 15.620171232876746, 15.09106164383565, 14.036267123287704, 12.869315068493185, 7.8992808219178405, 3.123595890410992, 0.18438356164386954, -4.110136986301336, -3.1914726027396925, -0.6640753424657198, -0.32674657534243234, -0.17263698630133661, -3.3370205479451727, -6.456883561643803, -8.483424657534215, -5.7591095890410635, -3.643527397260241, -2.173493150684898, 0.8333561643835955, -1.1794863013698293, -0.06133561643832236, 0.7905479452055131, -2.4842808219177748, -1.0510616438355829, -1.6418150684931172, -2.338732876712295, -0.7514041095890076, -1.9329109589040758, -2.396952054794487, -3.056198630136953, -2.677773972602706, -4.030513698630104, -3.247979452054761, -3.807910958904076, -3.7805136986301036, -2.1383904109588707, -1.115273972602706, 2.1518493150685267, 3.2023630136986636, 2.6912328767123617, 1.4968835616438692, -1.3044863013698296, -2.6289726027396925, -2.843013698630103, -1.3284589041095556, -0.5656164383561307, 1.161267123287705, 1.1878082191781156, 0.5208561643835956, 1.662123287671267, 1.0619520547945545, 2.0782191780822257, 0.1903767123288007, 0.029417808219211472, -0.07589041095887067, -0.29164383561640495, 0.20493150684934858, 0.6912328767123622, 1.910410958904143, 2.171541095890445, 1.473767123287705, 1.0234246575342805, 1.1612671232877056, 1.9172602739726368, 2.937808219178116, 1.3025342465753764, 1.1912328767123626, -0.06989726027393894, 0.20921232876715723, 1.7759931506849655, -0.2890753424657196, 0.0876369863014036, 0.3710273972603077, -0.974006849315035, -0.15465753424654166, -1.2103082191780485, -2.8139041095890076, -2.0904452054794183, -1.3729794520547607, -1.8627054794520213, -1.6529452054794183, -2.1135616438355824, -3.7685273972602404, -4.403801369862981, -2.628972602739693, -4.08017123287668, -2.6897602739725697, -0.07760273972599402, -1.1760616438355829, 1.3196575342466093, 0.38301369863017093, -2.031369863013665, -2.242842465753391, -4.480856164383528, -4.895239726027364, -3.051061643835583, -2.14866438356161, 0.8907191780822254, 0.5491095890411294, -2.574178082191748, -4.240273972602707, -5.87811643835613, -4.229999999999966, -0.46373287671229524, 1.103047945205513, 3.419828767123321, 3.5268493150685263, 3.1586986301370192, 4.286267123287704, 2.737465753424691, 1.3718835616438694, 0.9395205479452395, -1.4346232876711988, -1.338732876712295, -0.7265753424657195, -0.3353082191780485, 0.5414041095890747, -0.59643835616435, -1.0964383561643503, 0.18267123287674591, 1.0208561643835954, 1.939520547945239, 2.2211986301370197, 2.206643835616472, 1.4489383561644174, -0.21458904109585664, 0.9283904109589378, -0.15722602739722696, 0.5713698630137318, 2.296541095890444, 0.3932876712329102, -1.8335958904109253, -2.238561643835583, -2.032226027397227, -2.8395890410958575, 0.47890410958907437, 0.9301027397260607, 0.09619863013701963, 2.7143493150685263, 0.2374657534246909, 0.24431506849318407, -0.02452054794517189, 1.1390068493151024, 1.5328424657534587, 0.9703424657534588, -0.06047945205476002, -0.4688698630136645, 0.6972260273972943, -0.07417808219174693, 2.286267123287705, 0.7006506849315404, -1.4157876712328432, -1.2556849315068161, -1.8472945205479117, -2.437191780821885, 1.9566438356164717, 0.13386986301373227, 1.902705479452088, 2.1278767123288005, -0.6880479452054457, 2.6980821917808555, -0.7942123287670896, -0.15465753424654183, 0.32136986301373216, -0.20003424657530883, 1.41897260273976, 0.20664383561647215]
  out "CH3 Bin Readings":dbl[](array[numeric])=[5120.0, 5056.0, 4993.0, 5044.0, 5104.0, 4887.0, 4895.0, 5062.0, 5068.0, 4999.0, 5097.0, 5129.0, 5156.0, 4992.0, 5145.0, 5200.0, 5169.0, 5090.0, 4972.0, 5020.0, 5144.0, 5258.0, 5207.0, 5112.0, 5221.0, 5169.0, 5316.0, 5356.0, 5202.0, 5212.0, 5399.0, 5199.0, 5346.0, 5215.0, 5198.0, 5309.0, 5322.0, 5454.0, 5430.0, 5337.0, 5382.0, 5228.0, 5381.0, 5337.0, 5212.0, 5244.0, 5279.0, 5310.0, 5211.0, 5171.0, 5220.0, 5292.0, 5309.0, 5389.0, 5292.0, 5302.0, 5147.0, 5371.0, 5290.0, 5305.0, 5287.0, 5159.0, 5200.0, 5212.0, 5261.0, 5241.0, 5200.0, 5312.0, 5229.0, 5168.0, 5174.0, 5233.0, 5057.0, 5152.0, 5103.0, 5115.0, 5111.0, 5176.0, 5117.0, 5177.0, 5038.0, 5166.0, 5186.0, 5203.0, 4930.0, 5046.0, 4988.0, 5089.0, 5108.0, 5056.0, 5032.0, 5008.0, 5163.0, 5174.0, 5048.0, 5090.0, 5065.0, 5147.0, 5058.0, 5047.0, 5067.0, 5115.0, 5016.0, 4989.0, 4966.0, 5095.0, 4933.0, 4986.0, 4922.0, 5085.0, 5132.0, 5010.0, 5030.0, 5051.0, 5045.0, 5151.0, 5094.0, 5118.0, 5042.0, 4949.0, 5171.0, 4942.0, 5041.0, 5024.0, 5008.0, 4966.0, 5061.0, 5118.0, 5034.0, 5095.0, 4845.0, 5109.0, 5056.0, 4928.0, 5004.0, 4973.0, 5081.0, 5089.0, 5102.0, 4997.0, 5011.0, 4956.0, 5061.0, 5036.0, 5002.0, 4964.0, 5060.0, 5098.0, 5167.0, 4945.0, 5019.0, 5077.0, 4974.0, 4961.0, 4964.0, 4981.0, 5053.0, 5004.0, 5013.0, 5007.0, 5010.0, 4955.0, 4965.0, 5075.0, 5049.0, 4871.0, 4910.0, 4955.0, 5017.0, 4914.0, 5011.0, 4960.0, 5057.0, 5150.0, 5004.0, 5018.0, 5008.0, 4935.0, 4897.0, 5057.0, 5105.0, 4941.0, 5176.0, 5094.0, 5056.0, 4962.0, 5076.0, 5024.0, 5004.0, 4850.0, 5118.0, 4925.0, 4982.0, 5046.0, 5056.0, 5057.0, 4946.0, 5073.0, 5023.0, 5043.0, 5052.0, 4995.0, 5054.0, 5064.0, 5024.0, 5088.0, 4909.0, 5005.0, 4843.0, 4958.0, 4997.0, 5079.0, 4964.0, 4899.0, 4966.0, 5125.0, 5094.0, 4887.0, 4897.0, 4944.0, 5061.0, 4926.0, 5080.0, 4983.0, 4982.0, 4933.0, 5002.0, 5008.0, 4989.0, 4851.0, 5007.0, 5016.0, 4966.0, 5082.0, 5003.0, 5000.0, 5125.0, 4979.0, 5055.0, 4980.0, 4986.0, 5040.0, 4990.0, 5047.0, 5036.0, 5047.0, 4967.0, 4856.0, 4966.0, 4995.0, 5043.0, 4982.0, 5115.0, 5015.0, 4956.0, 5141.0, 5054.0, 4912.0, 5060.0, 5284.0, 5263.0, 5385.0, 5566.0, 5713.0, 5758.0, 5903.0, 6118.0, 6123.0, 6111.0, 6227.0, 6516.0, 6624.0, 6866.0, 6963.0, 6894.0, 6941.0, 6875.0, 7042.0, 6791.0, 6880.0, 6726.0, 6523.0, 6468.0, 6256.0, 6190.0, 6052.0, 5939.0, 5857.0, 5890.0, 5803.0, 5742.0, 5602.0, 5456.0, 5489.0, 5419.0, 5367.0, 5344.0, 5282.0, 5220.0, 5323.0, 5175.0, 5202.0, 5161.0, 5157.0, 5190.0, 5103.0, 4940.0, 5095.0, 5057.0, 4864.0, 5045.0, 5013.0, 4946.0, 4949.0, 5038.0, 4992.0, 4972.0, 4930.0, 4979.0, 5079.0, 4923.0, 4978.0, 4967.0, 4879.0, 4992.0, 4891.0, 5080.0, 5065.0, 4950.0, 5028.0, 5095.0, 4929.0, 4847.0, 5028.0, 5028.0, 5097.0, 5020.0, 5014.0, 5111.0, 4991.0, 5064.0, 4995.0, 5051.0, 5035.0, 4944.0, 4969.0, 4974.0, 4999.0, 5022.0, 4960.0, 5071.0, 5147.0, 5014.0, 5121.0, 4874.0, 5069.0, 4969.0, 4994.0, 4997.0, 4940.0, 5049.0, 5034.0, 5078.0, 5058.0, 5054.0, 5032.0, 4950.0, 4956.0, 5107.0, 4974.0, 5017.0, 5082.0, 4980.0, 5093.0, 5000.0, 4940.0, 4984.0, 5130.0, 4980.0, 5014.0, 4916.0, 4962.0, 4975.0, 5057.0, 5086.0, 5006.0, 5078.0, 5076.0, 4989.0, 4916.0, 4989.0, 5019.0, 5062.0, 5170.0, 5054.0, 5085.0, 4897.0, 4988.0, 4977.0, 5015.0, 5017.0, 5124.0, 4909.0, 5103.0, 4995.0, 5066.0, 4990.0, 4930.0, 5031.0, 4970.0, 5080.0, 4975.0, 5097.0, 4951.0, 5045.0, 5051.0, 5068.0, 4981.0, 5102.0, 5146.0, 5033.0, 4947.0, 5028.0, 5082.0, 4997.0, 5013.0, 4970.0, 5032.0, 4980.0, 4998.0, 5064.0, 5037.0, 5084.0, 4937.0, 5008.0, 5059.0, 4990.0, 5048.0, 5048.0, 4949.0, 5111.0, 4912.0, 5072.0, 5109.0, 4919.0, 4985.0, 4926.0, 4965.0, 5183.0, 4979.0, 5025.0, 4941.0, 4930.0, 4915.0, 4975.0, 4905.0, 4963.0, 5025.0, 5067.0, 4965.0, 5025.0, 4963.0, 5008.0, 5060.0, 5075.0, 4990.0, 5044.0, 5093.0, 5019.0, 5147.0, 5028.0, 4922.0, 4962.0, 5073.0, 5045.0, 4954.0, 4879.0, 5078.0, 5023.0, 5071.0, 4954.0, 5025.0, 5045.0, 4941.0, 4977.0, 5068.0, 4996.0, 4986.0, 5067.0, 5152.0, 5068.0, 5059.0, 5111.0, 5080.0, 4932.0, 4888.0, 5025.0, 5003.0, 5036.0, 5037.0, 5066.0, 4998.0, 5066.0, 5026.0, 4961.0, 5122.0, 5124.0, 5007.0, 4964.0, 4923.0, 5055.0, 5026.0, 4970.0, 5040.0, 5095.0, 5067.0, 5103.0, 5051.0, 5104.0, 5052.0, 4878.0, 5044.0, 5072.0, 5126.0, 4912.0, 5075.0, 4922.0, 5027.0, 4951.0, 5049.0, 4863.0, 5014.0, 5055.0, 5157.0, 5087.0, 5055.0, 5080.0, 5044.0, 4836.0, 4970.0, 5012.0, 5051.0, 5035.0, 4990.0, 5049.0, 4968.0, 5015.0, 4976.0, 4980.0, 5025.0, 5120.0, 4990.0, 5061.0, 5074.0, 4933.0, 5066.0, 4899.0, 5031.0, 5019.0]
  out "CH2 (molecular) smoothed":dbl[](array[numeric])=[14.218630136986288, 11.42839041095889, 8.956643835616426, 9.009726027397248, 9.493458904109577, 11.585924657534234, 13.788835616438343, 16.46349315068492, 15.523424657534232, 16.448082191780806, 19.51657534246574, 20.384726027397246, 23.73061643835615, 27.74345890410958, 29.339349315068482, 31.96863013698629, 31.165547945205468, 33.356472602739714, 34.819657534246566, 36.81708904109588, 40.01229452054793, 42.977191780821904, 44.01400684931505, 49.93181506849314, 55.74431506849314, 58.3924315068493, 60.49431506849314, 61.38215753424656, 62.77256849315066, 65.01999999999998, 71.02513698630135, 72.30510273972601, 72.60647260273971, 73.24260273972601, 74.52856164383562, 74.95664383561643, 75.02770547945205, 73.45835616438356, 72.25373287671232, 72.89328767123287, 74.13900684931505, 74.48660958904107, 72.49260273972601, 72.90356164383559, 72.41811643835615, 73.29910958904108, 72.30595890410959, 72.25287671232876, 69.21092465753425, 64.81023972602739, 62.69979452054793, 59.11417808219177, 60.420684931506834, 61.88729452054793, 61.549965753424644, 60.541404109589024, 57.90613013698629, 53.783698630136975, 55.45921232876711, 53.365034246575334, 52.08078767123287, 54.67667808219177, 49.73660958904108, 48.74260273972601, 48.5910616438356, 47.662123287671214, 48.752020547945186, 46.36931506849314, 45.263150684931496, 41.76914383561642, 40.31366438356163, 41.88044520547944, 39.27256849315067, 41.5910616438356, 40.779417808219165, 37.65184931506848, 37.764863013698616, 34.6715410958904, 30.90955479452053, 31.598767123287658, 30.769143835616426, 29.266575342465742, 31.886438356164376, 29.420684931506838, 30.15527397260273, 30.231472602739714, 29.70921232876711, 29.49602739726026, 29.7674315068493, 27.33678082191779, 25.344486301369848, 28.622739726027383, 25.599623287671214, 26.313664383561626, 25.151849315068475, 23.52171232876711, 21.85390410958903, 20.058527397260264, 20.841917808219165, 17.20835616438355, 19.885582191780806, 23.68866438356163, 21.08335616438355, 22.02171232876711, 19.229760273972587, 15.289691780821903, 13.42839041095889, 14.597054794520533, 15.920684931506834, 15.333356164383549, 19.07821917808218, 16.53198630136985, 13.490034246575329, 14.430102739726015, 13.08934931506848, 13.869315068493139, 14.264006849315056, 14.75030821917807, 15.390719178082179, 14.354760273972591, 14.043972602739714, 12.63558219178081, 11.44294520547944, 10.310239726027385, 13.37530821917807, 14.34534246575341, 14.021712328767109, 15.597054794520535, 12.560239726027383, 10.905273972602728, 12.285410958904096, 10.872739726027383, 13.039691780821904, 16.40784246575341, 16.837636986301355, 16.930102739726014, 14.645856164383547, 10.883013698630123, 6.707499999999985, 6.811952054794507, 6.538835616438343, 8.494315068493137, 9.221198630136973, 8.521712328767109, 6.520856164383548, 6.407842465753411, 6.601335616438342, 7.864178082191768, 7.988321917808206, 5.20921232876711, 5.513150684931493, 4.3119520547945065, 5.847910958904095, 3.365034246575328, 3.3693150684931368, 3.690376712328753, 4.893287671232863, 7.982328767123275, 7.728904109589028, 6.840205479452042, 4.673253424657521, 3.4960273972602605, 3.4686301369862886, 3.843630136986288, 6.003732876712316, 7.752876712328753, 8.153561643835603, 8.09962328767122, 6.421541095890397, 5.892431506849302, 6.2426027397260135, 5.7134931506849185, 4.697226027397247, 3.7340410958903973, 4.736609589041082, 7.025136986301356, 7.189520547945192, 8.180102739726014, 5.598767123287658, 4.573082191780809, 5.829075342465741, 6.019999999999987, 4.618458904109576, 3.902705479452042, 4.92839041095889, 4.848767123287658, 7.946369863013686, 8.708356164383549, 7.4027054794520435, 5.949794520547933, 3.791404109589028, 2.8581849315068366, 3.028561643835604, 3.848767123287659, 5.877876712328755, 5.857328767123275, 5.506301369863001, 7.442945205479438, 8.8924315068493, 6.974623287671219, 7.269999999999985, 4.335068493150671, 2.9258219178082054, 3.8333561643835483, 0.727191780821905, -0.15037671232878025, 0.19808219178080888, 0.20407534246573988, 2.140719178082178, 1.996883561643822, -0.30448630136987614, 0.9232534246575212, 1.2845547945205351, 4.597054794520536, 4.487465753424646, 4.565376712328755, 2.6621232876712204, 2.0080136986301236, 2.3727397260273837, 0.36760273972601387, 4.706643835616425, 4.693801369863001, 3.4249657534246447, 4.436095890410947, 1.8470547945205351, -0.3318835616438487, 1.4386643835616304, 2.958356164383548, 5.886438356164369, 6.665547945205465, 5.4215410958903965, 4.222910958904096, 0.7896917808219047, 0.8530479452054662, 0.666404109589028, -1.3695547945205613, -2.2359931506849446, -3.177773972602753, -0.7214383561643969, 1.4515068493150558, 1.9472260273972475, 2.448938356164371, 1.2400342465753291, 1.54226027397259, 4.585924657534234, 4.6689726027397125, 5.7511643835616315, 5.116746575342453, 4.121027397260262, 5.263150684931494, 5.019999999999987, 5.1467123287671095, 4.369315068493138, 3.685239726027384, 1.666404109589028, -0.04250000000001308, -0.4722945205479586, 0.5705136986301237, 2.408698630136973, 3.8136643835616306, 1.9908904109588914, 1.4711986301369733, 0.9360958904109458, 1.558527397260261, 2.39157534246574, 3.656130136986288, 2.8299315068493023, 2.9086986301369735, 5.058527397260262, 5.598767123287659, 6.0816438356164255, 5.341061643835603, 3.706643835616425, 1.5902054794520417, 2.508013698630124, 2.067089041095877, 1.4172602739725897, 3.746027397260261, 2.880445205479439, 3.8153767123287543, 7.763150684931494, 7.011438356164371, 7.910410958904096, 8.653561643835603, 6.114178082191768, 5.790547945205467, 5.597910958904096, 2.6509931506849185, 2.379589041095877, 0.34619863013697316, -2.937191780821931, 0.2597260273972466, -0.7625342465753562, -0.8926712328767261, 0.9985958904109454, -0.2351369863013828, 1.2126369863013566, 0.2734246575342334, -0.9303424657534374, -2.076746575342478, -3.2925000000000124, 0.06366438356163107, 0.9814726027397127, 1.7768493150684799, 0.5756506849314933, -0.3087671232876843, 1.000308219178069, 3.0105821917808084, 5.983184931506836, 4.986609589041082, 7.660410958904095, 5.507157534246562, 2.9900342465753296, 2.9121232876712195, 0.7229109589040966, 1.5088698630136859, 2.08934931506848, -0.12383561643836871, -2.038219178082204, -1.5099657534246702, 1.1098972602739605, 1.1527054794520417, 1.7040753424657407, 0.9146917808219047, 2.794828767123274, 6.869315068493137, 10.600479452054781, 11.319657534246561, 7.190376712328754, 6.6509931506849185, 2.4908904109588916, 0.6544178082191655, -0.04078767123288907, -1.8601369863013828, -1.4508904109589171, -1.7719520547945335, -1.2214383561643967, 2.781130136986288, 3.5867808219177943, 4.7785616438356024, 6.023424657534234, 4.34448630136985, 3.400993150684919, 1.4754794520547818, 1.4472260273972473, 1.6732534246575215, 3.069657534246563, 4.595342465753411, 3.3444863013698503, 3.3205136986301245, 2.0003082191780694, 1.4797602739725901, 1.7503082191780694, 1.9086986301369735, 0.5199999999999871, 0.6287328767123154, 0.5824999999999867, -0.05705479452056128, 3.370171232876699, 4.368458904109575, 2.7220547945205347, 0.8470547945205343, 0.3761643835616306, 0.23917808219176806, 3.9095547945205356, 6.769999999999987, 6.811095890410947, 8.136438356164371, 6.65184931506848, 3.3992808219177943, 0.11674657534245236, 0.06623287671231548, 0.31109589041094576, 0.7066438356164253, 3.2220547945205347, 3.7931164383561518, 4.0927739726027275, 3.856472602739714, 2.8119520547945083, -1.2068835616438485, -3.6615068493150815, -2.9979794520548078, -2.7967808219178214, 0.06537671232875364, 2.4934589041095756, 2.007157534246562, 2.559383561643822, 1.989178082191768, -1.1264041095890538, 1.786267123287658, 4.14157534246574, 0.9181164383561509, 3.0328424657534114, 0.8984246575342335, 0.052534246575329346, 5.132157534246561, 6.0439726027397125, 7.752020547945191, 7.379589041095877, 5.582499999999987, 5.335068493150673, 2.1655479452054665, 1.9232534246575212, 0.5071575342465624, -0.2496917808219305, 2.0388356164383437, 0.6801027397260146, 3.843630136986289, 7.212636986301357, 3.4489383561643696, 3.1253082191780686, 1.2665753424657393, -1.2659589041096027, 1.239178082191768, 2.8958561643835483, 1.1278767123287536, 0.3838698630136854, -0.5073972602739859, -2.1837671232876836, -0.13924657534247864, -1.102431506849328, 0.21520547945204171, 0.267431506849302, -0.77537671232878, -0.042500000000012694, -0.005684931506862112, 2.3872945205479326, 4.136438356164371, 3.0688013698630012, 2.196369863013686, -0.301917808219191, -1.4389041095890542, 0.7143493150684803, -0.1486643835616568, 1.7160616438356033, 0.09106164383560333, -0.9877054794520678, 1.2015068493150558, 1.0670890410958778, 2.538835616438343, 2.304246575342453, 2.7717123287671095, 1.4215410958903976, 2.430958904109576, 2.5996232876712195, 2.975479452054781, 4.545684931506836, 1.6604109589040954, 4.369315068493137, 3.4857534246575206, -0.24455479452056061, -0.4123630136986429, -2.158938356164396, -1.5425000000000126, -1.7976369863013824, 2.8042465753424524, 1.502876712328754, 1.0636643835616304, 2.722910958904096, 1.5850684931506716, 3.704931506849302, 3.147568493150672, 6.425821917808205, 7.533698630136973, 7.830787671232864, 6.799109589041082, 1.2348972602739585, -1.5810273972602873, -1.2111643835616572, 0.644999999999986, 3.6860958904109453, 3.870171232876699, 3.4814726027397125, 0.31452054794519246, 3.028561643835603, 3.0576712328766993, 2.305958904109576, 5.375308219178069, 2.003732876712316, 4.87102739726026, 6.0063013698629995, 2.4189726027397125, 2.506301369863, 1.3881506849314944, -0.2582534246575464, 3.098767123287659, 4.2289041095890285, 3.9789041095890285, 3.82393835616437, 1.5533904109588907, 3.316232876712315, 4.049965753424644, 6.196369863013685, 10.13643835616437, 10.048253424657519, 6.49688356164382, 5.376164383561629, 1.2888356164383412, -1.3721232876712461, 0.9266780821917681, -1.6332534246575472, -1.7805136986301497, -1.977431506849328, -2.8087671232876845, -2.867842465753438, -0.8823972602739859, -1.0690410958904244, 1.1081849315068357, 1.1886643835616304, -0.2445547945205615, 2.1852397260273837, -0.02109589041097204, 1.673253424657521, 3.7468835616438216, 4.4814726027397125, 3.800821917808206, 5.407842465753411, 3.403561643835604, 1.1253082191780688, 3.1741095890410826, 1.1098972602739596, 3.564520547945193, 5.163835616438343, 5.782842465753411, 6.273424657534234, 7.059383561643822, 6.414691780821904, 3.4232534246575206, 0.2520205479451927, -2.367842465753437, -4.933767123287684, -5.500547945205492, -4.715445205479465, -1.661506849315082, 2.906130136986288, 4.909554794520535, 9.288835616438343, 7.939520547945193, 3.390719178082179, 2.5063013698630012, -0.5519178082191905, -2.166643835616451, -2.896952054794533, -1.8746917808219306, 0.6158904109588916, 0.29568493150683683, 0.9386643835616311, -1.9740068493150809, -1.9157876712328892, -3.8370205479452184, -2.878972602739739, -3.0493493150685063, -4.896952054794534, -2.0313698630137114, -0.6897602739726155]
  out "CH 2 Bin Readings":dbl[](array[numeric])=[9876.0, 9729.0, 9869.0, 9694.0, 9667.0, 9998.0, 9701.0, 9893.0, 9744.0, 9929.0, 9875.0, 9959.0, 9757.0, 9800.0, 9655.0, 9858.0, 9784.0, 9837.0, 9778.0, 9609.0, 9905.0, 9751.0, 9790.0, 9737.0, 9812.0, 9735.0, 9946.0, 9837.0, 9893.0, 9991.0, 9922.0, 9805.0, 9875.0, 9729.0, 9922.0, 9882.0, 9853.0, 9971.0, 9917.0, 9948.0, 9966.0, 10004.0, 10062.0, 9851.0, 9925.0, 9960.0, 9990.0, 10114.0, 10003.0, 9955.0, 10007.0, 9949.0, 9748.0, 9979.0, 10077.0, 9865.0, 9892.0, 9904.0, 9854.0, 9949.0, 9811.0, 10039.0, 9924.0, 9769.0, 9794.0, 9853.0, 9928.0, 9624.0, 9780.0, 9806.0, 9711.0, 9824.0, 9844.0, 9879.0, 9898.0, 10077.0, 9759.0, 9942.0, 9759.0, 9820.0, 9958.0, 9670.0, 9741.0, 9864.0, 9926.0, 9781.0, 9863.0, 9929.0, 9787.0, 9806.0, 9937.0, 9873.0, 9783.0, 9795.0, 9846.0, 9782.0, 9811.0, 9843.0, 9726.0, 9961.0, 9997.0, 9749.0, 9928.0, 9904.0, 9944.0, 9694.0, 9687.0, 9966.0, 9676.0, 9575.0, 9901.0, 9725.0, 9706.0, 9654.0, 9911.0, 9939.0, 9802.0, 9715.0, 9765.0, 9870.0, 9999.0, 9672.0, 9848.0, 9906.0, 9809.0, 9918.0, 9480.0, 9802.0, 9876.0, 9748.0, 9799.0, 9728.0, 9885.0, 9814.0, 9826.0, 9878.0, 9803.0, 9861.0, 9780.0, 9777.0, 9623.0, 9680.0, 9745.0, 9642.0, 9776.0, 9845.0, 9716.0, 9682.0, 9894.0, 9906.0, 9800.0, 9654.0, 9805.0, 9806.0, 9838.0, 9968.0, 9876.0, 9798.0, 9702.0, 9999.0, 9595.0, 9664.0, 9810.0, 9884.0, 9821.0, 9597.0, 9727.0, 9851.0, 9735.0, 9910.0, 9840.0, 9905.0, 9853.0, 9856.0, 9901.0, 9786.0, 9956.0, 9839.0, 9975.0, 9693.0, 9684.0, 9887.0, 9729.0, 9869.0, 9628.0, 9912.0, 9794.0, 9743.0, 9826.0, 9733.0, 9760.0, 9931.0, 9691.0, 9889.0, 9857.0, 9755.0, 9725.0, 9656.0, 9630.0, 10000.0, 9684.0, 9720.0, 9704.0, 9816.0, 9900.0, 9753.0, 9785.0, 9830.0, 9860.0, 9816.0, 9775.0, 9829.0, 9885.0, 9843.0, 9677.0, 9805.0, 9714.0, 9790.0, 9823.0, 9659.0, 9843.0, 9711.0, 9864.0, 9735.0, 9688.0, 9820.0, 9809.0, 9673.0, 9651.0, 9869.0, 9880.0, 9838.0, 9634.0, 9751.0, 9789.0, 9682.0, 9838.0, 9879.0, 9737.0, 9915.0, 9879.0, 9692.0, 9742.0, 9777.0, 9711.0, 9767.0, 9827.0, 9821.0, 9806.0, 9857.0, 9705.0, 9866.0, 9856.0, 9824.0, 9771.0, 9870.0, 9787.0, 9842.0, 9751.0, 9784.0, 9833.0, 9782.0, 9704.0, 9701.0, 9797.0, 9790.0, 9800.0, 9831.0, 9629.0, 9637.0, 9844.0, 9837.0, 9716.0, 9757.0, 9840.0, 9754.0, 9732.0, 9689.0, 9732.0, 9606.0, 9725.0, 9926.0, 9960.0, 9651.0, 9757.0, 9740.0, 9847.0, 9664.0, 9924.0, 9880.0, 9731.0, 9732.0, 9887.0, 9717.0, 9804.0, 9763.0, 9919.0, 9784.0, 9911.0, 9945.0, 9761.0, 9844.0, 9829.0, 9888.0, 9704.0, 9699.0, 9849.0, 9812.0, 9707.0, 9842.0, 9815.0, 9787.0, 9761.0, 9702.0, 9781.0, 9804.0, 9892.0, 9804.0, 9758.0, 9769.0, 9840.0, 9761.0, 9852.0, 9764.0, 9757.0, 10048.0, 9707.0, 9737.0, 9861.0, 9861.0, 9727.0, 9819.0, 9827.0, 9841.0, 9677.0, 9695.0, 9844.0, 9796.0, 9741.0, 9555.0, 9981.0, 9627.0, 9796.0, 9731.0, 9788.0, 9990.0, 9575.0, 9905.0, 9886.0, 9663.0, 9894.0, 9832.0, 9614.0, 9684.0, 9651.0, 9752.0, 9732.0, 9772.0, 9884.0, 9645.0, 9834.0, 9871.0, 9971.0, 9567.0, 9603.0, 9853.0, 9857.0, 9762.0, 9850.0, 9778.0, 9762.0, 9713.0, 9822.0, 9908.0, 9839.0, 9922.0, 9769.0, 9840.0, 9863.0, 9834.0, 9764.0, 9813.0, 9776.0, 9805.0, 10039.0, 9915.0, 9745.0, 9698.0, 9756.0, 9761.0, 9924.0, 9678.0, 9787.0, 9915.0, 9710.0, 9797.0, 9786.0, 9972.0, 9795.0, 9734.0, 9673.0, 9764.0, 9808.0, 9901.0, 9779.0, 9621.0, 9889.0, 9720.0, 9833.0, 9691.0, 9794.0, 9891.0, 9681.0, 9685.0, 9724.0, 9820.0, 9753.0, 9767.0, 9623.0, 9629.0, 9843.0, 9862.0, 9827.0, 9981.0, 9789.0, 9800.0, 9830.0, 9811.0, 9748.0, 9824.0, 9824.0, 9694.0, 9803.0, 9848.0, 9830.0, 9840.0, 9870.0, 9879.0, 9629.0, 9779.0, 9758.0, 9740.0, 9779.0, 9936.0, 9689.0, 9634.0, 9643.0, 9876.0, 9685.0, 9849.0, 9717.0, 9881.0, 9787.0, 9701.0, 9858.0, 9671.0, 9843.0, 9740.0, 9707.0, 9784.0, 9924.0, 9701.0, 9716.0, 9782.0, 9857.0, 9738.0, 9831.0, 9975.0, 9920.0, 9806.0, 9768.0, 9941.0, 9795.0, 9817.0, 9765.0, 9852.0, 9870.0, 9864.0, 9874.0, 9723.0, 9962.0, 9935.0, 9711.0, 9784.0, 9947.0, 9803.0, 9874.0, 9816.0, 9701.0, 9815.0, 9881.0, 9812.0, 9722.0, 9914.0, 9738.0, 9956.0, 9776.0, 9882.0, 9820.0, 9834.0, 9719.0, 9734.0, 9830.0, 9892.0, 9817.0, 9763.0, 9951.0, 9757.0, 9947.0, 9740.0, 9767.0, 9729.0, 9759.0, 9920.0, 9954.0, 9901.0, 9958.0, 9724.0, 9717.0, 9738.0, 9817.0, 9688.0, 9786.0, 9802.0, 9754.0, 9895.0, 9603.0, 9840.0, 9659.0, 9932.0, 9981.0, 9716.0, 9815.0, 9902.0, 9849.0, 9541.0, 9843.0, 9741.0, 9902.0, 9816.0, 9785.0, 9739.0, 9741.0, 9805.0, 9742.0, 9800.0, 9887.0, 9693.0, 9832.0, 9963.0, 9678.0, 9690.0, 9875.0, 9742.0, 9870.0, 9825.0, 9610.0, 9815.0, 9698.0]
  in  "stop":bool
  in  "Reset Average":bool=TRUE
  in  "Save Data?":bool=TRUE
  in  "Collect Data?":bool=TRUE
  in  "ILX Address":i32=6 min=0 step=1
  in  "Lambda On DBR Current":dbl=171.13999999999868
  in  "Lambda Off DBR Current":dbl=172.9499999999997
  in  "Tab Control":T2(tab)=enum."NRB"
  out "NRB plot":cluster{"Y":dbl[], "Y":dbl[]}[](graph)=[{"Y"=[0.0, 0.0, 0.0, 0.0, 0.0, 0.0, 0.0, 0.0, 0.0, 0.0, 0.0, 0.0, 0.0, 0.0, 0.0, 0.0, 0.0, 0.0, 0.0, 0.0, 0.0, 0.0, 0.0, 0.0, 0.0, 0.0, 0.0, 0.0, 0.0, 0.0, 0.0, 0.0, 0.0, 0.0, 0.0, 0.0, 0.0, 0.0, 0.0, 0.0, 0.0, 0.0, 0.0, 0.0, 0.0, 0.0, 0.0, 0.0, 0.0, 0.0, 0.0, 0.0, 0.0, 0.0, 0.0, 0.0, 0.0, 0.0, 0.0, 0.0, 0.0, 0.0, 0.0, 0.0, 0.0, 0.0, 0.0, 0.0, 0.0, 0.0, 0.0, 0.0, 0.0, 0.0, 0.0, 0.0, 0.0, 0.0, 0.0, 0.0, 0.0, 0.0, 0.0, 0.0, 0.0, 0.0, 0.0, 0.0, 0.0, 0.0, 0.0, 0.0, 0.0, 0.0, 0.0, 0.0, 0.0, 0.0, 0.0, 0.0, 0.0, 0.0, 0.0, 0.0, 0.0, 0.0, 0.0, 0.0, 0.0, 0.0, 0.0, 0.0, 0.0, 0.0, 0.0, 0.0, 0.0, 0.0, 0.0, 0.0, 0.0, 0.0, 0.0, 0.0, 0.0, 0.0, 0.0, 0.0, 0.0, 0.0, 0.0, 0.0, 0.0, 0.0, 0.0, 0.0, 0.0, 0.0, 0.0, 0.0, 0.0, 0.0, 0.0, 0.0, 0.0, 0.0, 0.0, 0.0, 0.0, 0.0, 0.0, 0.0, 0.0, 0.0, 0.0, 0.0, 0.0, 0.0, 0.0, 0.0, 0.0, 0.0, 0.0, 0.0, 0.0, 0.0, 0.0, 0.0, 0.0, 0.0, 0.0, 0.0, 0.0, 0.0, 0.0, 0.0, 0.0, 0.0, 0.0, 0.0, 0.0, 0.0, 0.0, 0.0, 0.0, 0.0, 0.0, 0.0, 0.0, 0.0, 0.0, 0.0, 0.0, 0.0, 0.0, 0.0, 0.0, 0.0, 0.0, 0.0, 0.0, 0.0, 0.0, 0.0, 0.0, 0.0, 0.0, 0.0, 0.0, 0.0, 0.0, 0.0, 0.0, 0.0, 0.0, 0.0, 0.0, 0.0, 0.0, 0.0, 0.0, 0.0, 0.0, 0.0, 0.0, 0.0, 0.0, 0.0, 0.0, 0.0, 0.0, 0.0, 0.0, 0.0, 0.0, 0.0, 0.0, 0.0, 0.0, 0.0, 0.0, 0.0, 0.0, 0.0, 0.0, 0.0, 0.0, 0.0, 0.0, 0.0, 0.0, 0.0, 0.0, 0.0, 0.0, 0.0, 0.0, 0.0, 0.0, 0.0, 0.0, 0.0, 0.0, 0.0, 0.0, 0.0, 0.0, 0.0, 0.0, 0.0, 0.0, 0.0, 0.0, 0.0, 0.0, 0.0, 0.0, 0.0, 0.0, 0.0, 0.0, 0.0, 0.0, 0.0, 0.0, 0.0, 0.0, 0.0, 0.0, 0.0, 0.0, 0.0, 0.0, 0.0, 0.0, 0.0, 0.0, 0.0, 0.0, 0.0, 0.0, 0.0, 0.0, 0.0, 0.0, 0.0, 0.0, 0.0, 0.0, 0.0, 0.0, 0.0, 0.0, 0.0, 0.0, 0.0, 0.0, 0.0, 0.0, 0.0, 0.0, 0.0, 0.0, 0.0, 0.0, 0.0, 0.0, 0.0, 0.0, 0.0, 0.0, 0.0, 0.0, 0.0, 0.0, 0.0, 0.0, 0.0, 0.0, 0.0, 0.0, 0.0, 0.0, 0.0, 0.0, 0.0, 0.0, 0.0, 0.0, 0.0, 0.0, 0.0, 0.0, 0.0, 0.0, 0.0, 0.0, 0.0, 0.0, 0.0, 0.0, 0.0, 0.0, 0.0, 0.0, 0.0, 0.0, 0.0, 0.0, 0.0, 0.0, 0.0, 0.0, 0.0, 0.0, 0.0, 0.0, 0.0, 0.0, 0.0, 0.0, 0.0, 0.0, 0.0, 0.0, 0.0, 0.0, 0.0, 0.0, 0.0, 0.0, 0.0, 0.0, 0.0, 0.0, 0.0, 0.0, 0.0, 0.0, 0.0, 0.0, 0.0, 0.0, 0.0, 0.0, 0.0, 0.0, 0.0, 0.0, 0.0, 0.0, 0.0, 0.0, 0.0, 0.0, 0.0, 0.0, 0.0, 0.0, 0.0, 0.0, 0.0, 0.0, 0.0, 0.0, 0.0, 0.0, 0.0, 0.0, 0.0, 0.0, 0.0, 0.0, 0.0, 0.0, 0.0, 0.0, 0.0, 0.0, 0.0, 0.0, 0.0, 0.0, 0.0, 0.0, 0.0, 0.0, 0.0, 0.0, 0.0, 0.0, 0.0, 0.0, 0.0, 0.0, 0.0, 0.0, 0.0, 0.0, 0.0, 0.0, 0.0, 0.0, 0.0, 0.0, 0.0, 0.0, 0.0, 0.0, 0.0, 0.0, 0.0, 0.0, 0.0, 0.0, 0.0, 0.0, 0.0, 0.0, 0.0, 0.0, 0.0, 0.0, 0.0, 0.0, 0.0, 0.0, 0.0, 0.0, 0.0, 0.0, 0.0, 0.0, 0.0, 0.0, 0.0, 0.0, 0.0, 0.0, 0.0, 0.0, 0.0, 0.0, 0.0, 0.0, 0.0, 0.0, 0.0, 0.0, 0.0, 0.0, 0.0, 0.0, 0.0, 0.0, 0.0, 0.0, 0.0, 0.0, 0.0, 0.0, 0.0, 0.0, 0.0, 0.0, 0.0, 0.0, 0.0, 0.0, 0.0, 0.0, 0.0, 0.0, 0.0, 0.0, 0.0, 0.0, 0.0, 0.0, 0.0, 0.0, 0.0, 0.0, 0.0, 0.0, 0.0, 0.0, 0.0, 0.0, 0.0, 0.0, 0.0, 0.0, 0.0, 0.0], "Y"=[0.0375, 0.075, 0.11249999999999999, 0.15, 0.1875, 0.225, 0.26249999999999996, 0.3, 0.33749999999999997, 0.37499999999999994, 0.4125, 0.44999999999999996, 0.48749999999999993, 0.525, 0.5625, 0.6, 0.6375, 0.6749999999999999, 0.7124999999999999, 0.75, 0.7875, 0.825, 0.8624999999999999, 0.8999999999999999, 0.9374999999999999, 0.975, 1.0125, 1.05, 1.0875000000000001, 1.125, 1.1625, 1.2, 1.2375, 1.2750000000000001, 1.3125, 1.35, 1.3875, 1.425, 1.4625000000000001, 1.5, 1.5375, 1.575, 1.6125, 1.6500000000000001, 1.6875, 1.725, 1.7625, 1.8, 1.8375, 1.875, 1.9125, 1.95, 1.9875, 2.025, 2.0625, 2.1, 2.1375, 2.175, 2.2125, 2.25, 2.2875, 2.325, 2.3625, 2.4, 2.4375, 2.475, 2.5125, 2.55, 2.5875, 2.625, 2.6625, 2.7, 2.7375, 2.775, 2.8125, 2.85, 2.8875, 2.925, 2.9625, 3.0, 3.0375, 3.075, 3.1125, 3.15, 3.1875, 3.225, 3.2625, 3.3, 3.3375, 3.375, 3.4125, 3.45, 3.4875, 3.525, 3.5625, 3.6, 3.6374999999999997, 3.675, 3.7125, 3.75, 3.7875, 3.8249999999999997, 3.8625, 3.9, 3.9375, 3.975, 4.012499999999999, 4.05, 4.0874999999999995, 4.124999999999999, 4.1625, 4.199999999999999, 4.2375, 4.2749999999999995, 4.312499999999999, 4.35, 4.387499999999999, 4.425, 4.4624999999999995, 4.499999999999999, 4.5375, 4.574999999999999, 4.6125, 4.6499999999999995, 4.687499999999999, 4.725, 4.762499999999999, 4.8, 4.8374999999999995, 4.874999999999999, 4.9125, 4.949999999999999, 4.9875, 5.0249999999999995, 5.062499999999999, 5.1, 5.137499999999999, 5.175, 5.2124999999999995, 5.249999999999999, 5.2875, 5.324999999999999, 5.3625, 5.3999999999999995, 5.437499999999999, 5.475, 5.512499999999999, 5.55, 5.5874999999999995, 5.624999999999999, 5.6625, 5.699999999999999, 5.7375, 5.7749999999999995, 5.812499999999999, 5.85, 5.887499999999999, 5.925, 5.9624999999999995, 5.999999999999999, 6.0375, 6.074999999999999, 6.1125, 6.1499999999999995, 6.187499999999999, 6.225, 6.262499999999999, 6.3, 6.3374999999999995, 6.374999999999999, 6.4125, 6.449999999999999, 6.4875, 6.5249999999999995, 6.562499999999999, 6.6, 6.637499999999999, 6.675, 6.7124999999999995, 6.749999999999999, 6.7875, 6.824999999999999, 6.8625, 6.8999999999999995, 6.937499999999999, 6.975, 7.012499999999999, 7.05, 7.0874999999999995, 7.124999999999999, 7.1625, 7.199999999999999, 7.237499999999999, 7.2749999999999995, 7.312499999999999, 7.35, 7.387499999999999, 7.424999999999999, 7.4624999999999995, 7.499999999999999, 7.5375, 7.574999999999999, 7.612499999999999, 7.6499999999999995, 7.687499999999999, 7.725, 7.762499999999999, 7.799999999999999, 7.8374999999999995, 7.874999999999999, 7.9125, 7.949999999999999, 7.987499999999999, 8.025, 8.0625, 8.1, 8.1375, 8.174999999999999, 8.212499999999999, 8.25, 8.2875, 8.325, 8.362499999999999, 8.399999999999999, 8.4375, 8.475, 8.5125, 8.549999999999999, 8.587499999999999, 8.625, 8.6625, 8.7, 8.737499999999999, 8.774999999999999, 8.8125, 8.85, 8.8875, 8.924999999999999, 8.962499999999999, 9.0, 9.0375, 9.075, 9.112499999999999, 9.149999999999999, 9.1875, 9.225, 9.2625, 9.299999999999999, 9.337499999999999, 9.375, 9.4125, 9.45, 9.487499999999999, 9.524999999999999, 9.5625, 9.6, 9.6375, 9.674999999999999, 9.712499999999999, 9.75, 9.7875, 9.825, 9.862499999999999, 9.899999999999999, 9.9375, 9.975, 10.0125, 10.049999999999999, 10.087499999999999, 10.125, 10.1625, 10.2, 10.237499999999999, 10.274999999999999, 10.3125, 10.35, 10.3875, 10.424999999999999, 10.462499999999999, 10.5, 10.5375, 10.575, 10.612499999999999, 10.649999999999999, 10.6875, 10.725, 10.7625, 10.799999999999999, 10.837499999999999, 10.875, 10.9125, 10.95, 10.987499999999999, 11.024999999999999, 11.0625, 11.1, 11.1375, 11.174999999999999, 11.212499999999999, 11.25, 11.2875, 11.325, 11.362499999999999, 11.399999999999999, 11.4375, 11.475, 11.5125, 11.549999999999999, 11.587499999999999, 11.625, 11.6625, 11.7, 11.737499999999999, 11.774999999999999, 11.8125, 11.85, 11.8875, 11.924999999999999, 11.962499999999999, 12.0, 12.0375, 12.075, 12.112499999999999, 12.149999999999999, 12.1875, 12.225, 12.2625, 12.299999999999999, 12.337499999999999, 12.375, 12.4125, 12.45, 12.487499999999999, 12.524999999999999, 12.5625, 12.6, 12.6375, 12.674999999999999, 12.712499999999999, 12.75, 12.7875, 12.825, 12.862499999999999, 12.899999999999999, 12.9375, 12.975, 13.0125, 13.049999999999999, 13.087499999999999, 13.125, 13.1625, 13.2, 13.237499999999999, 13.274999999999999, 13.3125, 13.35, 13.3875, 13.424999999999999, 13.462499999999999, 13.5, 13.5375, 13.575, 13.612499999999999, 13.649999999999999, 13.6875, 13.725, 13.7625, 13.799999999999999, 13.837499999999999, 13.875, 13.9125, 13.95, 13.987499999999999, 14.024999999999999, 14.0625, 14.1, 14.1375, 14.174999999999999, 14.212499999999999, 14.25, 14.2875, 14.325, 14.362499999999999, 14.399999999999999, 14.437499999999998, 14.475, 14.5125, 14.549999999999999, 14.587499999999999, 14.624999999999998, 14.6625, 14.7, 14.737499999999999, 14.774999999999999, 14.812499999999998, 14.85, 14.8875, 14.924999999999999, 14.962499999999999, 14.999999999999998, 15.0375, 15.075, 15.112499999999999, 15.149999999999999, 15.187499999999998, 15.225, 15.2625, 15.299999999999999, 15.337499999999999, 15.374999999999998, 15.4125, 15.45, 15.487499999999999, 15.524999999999999, 15.562499999999998, 15.6, 15.6375, 15.674999999999999, 15.712499999999999, 15.749999999999998, 15.7875, 15.825, 15.862499999999999, 15.899999999999999, 15.937499999999998, 15.975, 16.0125, 16.05, 16.087500000000002, 16.125, 16.1625, 16.2, 16.2375, 16.275000000000002, 16.3125, 16.35, 16.3875, 16.425, 16.462500000000002, 16.5, 16.5375, 16.575, 16.6125, 16.650000000000002, 16.6875, 16.725, 16.7625, 16.8, 16.837500000000002, 16.875, 16.9125, 16.95, 16.9875, 17.025000000000002, 17.0625, 17.1, 17.1375, 17.175, 17.212500000000002, 17.25, 17.2875, 17.325, 17.3625, 17.400000000000002, 17.4375, 17.475, 17.5125, 17.55, 17.587500000000002, 17.625, 17.6625, 17.7, 17.7375, 17.775000000000002, 17.8125, 17.85, 17.8875, 17.925, 17.962500000000002, 18.0, 18.0375, 18.075, 18.1125, 18.150000000000002, 18.1875, 18.225, 18.2625, 18.3, 18.337500000000002, 18.375, 18.4125, 18.45, 18.4875, 18.525000000000002, 18.5625, 18.6, 18.6375, 18.675, 18.712500000000002, 18.75, 18.7875, 18.825, 18.8625, 18.900000000000002, 18.9375, 18.975, 19.0125, 19.05, 19.087500000000002, 19.125, 19.1625, 19.2, 19.2375, 19.275000000000002, 19.3125, 19.35, 19.3875, 19.425, 19.462500000000002, 19.5, 19.5375, 19.575, 19.6125, 19.650000000000002, 19.6875, 19.725, 19.7625, 19.8, 19.837500000000002, 19.875, 19.9125, 19.95, 19.9875, 20.025000000000002, 20.0625, 20.1, 20.1375, 20.175, 20.212500000000002, 20.25, 20.2875, 20.325, 20.3625, 20.400000000000002, 20.4375, 20.475, 20.5125, 20.55, 20.587500000000002, 20.625, 20.6625, 20.7, 20.7375, 20.775000000000002, 20.8125, 20.85, 20.8875, 20.925, 20.962500000000002, 21.0]}, ...(2 in all)]
  in  "background length":i32=25
  out "Correction":cluster{"Y":dbl[], "Y":dbl[]}[](graph)=[{"Y"=[1.0, 1.0, 1.0, 1.0, 1.0, 1.0, 1.0, 1.0, 1.0, 1.0, 1.0, 1.0, 1.0, 1.0, 1.0, 1.0, 1.0, 1.0, 1.0, 1.0, 1.0, 1.0, 1.0, 1.0, 1.0, 1.0, 1.0, 1.0, 1.0, 1.0, 1.0, 1.0, 1.0, 1.0, 1.0, 1.0, 1.0, 1.0, 1.0, 1.0, 1.0, 1.0, 1.0, 1.0, 1.0, 1.0, 1.0, 1.0, 1.0, 1.0, 1.0, 1.0, 1.0, 1.0, 1.0, 1.0, 1.0, 1.0, 1.0, 1.0, 1.0, 1.0, 1.0, 1.0, 1.0, 1.0, 1.0, 1.0, 1.0, 1.0, 1.0, 1.0, 1.0, 1.0, 1.0, 1.0, 1.0, 1.0, 1.0, 1.0, 1.0, 1.0, 1.0, 1.0, 1.0, 1.0, 1.0, 1.0, 1.0, 1.0, 1.0, 1.0, 1.0, 1.0, 1.0, 1.0, 1.0, 1.0, 1.0, 1.0, 1.0, 1.0, 1.0, 1.0, 1.0, 1.0, 1.0, 1.0, 1.0, 1.0, 1.0, 1.0, 1.0, 1.0, 1.0, 1.0, 1.0, 1.0, 1.0, 1.0, 1.0, 1.0, 1.0, 1.0, 1.0, 1.0, 1.0, 1.0, 1.0, 1.0, 1.0, 1.0, 1.0, 1.0, 1.0, 1.0, 1.0, 1.0, 1.0, 1.0, 1.0, 1.0, 1.0, 1.0, 1.0, 1.0, 1.0, 1.0, 1.0, 1.0, 1.0, 1.0, 1.0, 1.0, 1.0, 1.0, 1.0, 1.0, 1.0, 1.0, 1.0, 1.0, 1.0, 1.0, 1.0, 1.0, 1.0, 1.0, 1.0, 1.0, 1.0, 1.0, 1.0, 1.0, 1.0, 1.0, 1.0, 1.0, 1.0, 1.0, 1.0, 1.0, 1.0, 1.0, 1.0, 1.0, 1.0, 1.0, 1.0, 1.0, 1.0, 1.0, 1.0, 1.0, 1.0, 1.0, 1.0, 1.0, 1.0, 1.0, 1.0, 1.0, 1.0, 1.0, 1.0, 1.0, 1.0, 1.0, 1.0, 1.0, 1.0, 1.0, 1.0, 1.0, 1.0, 1.0, 1.0, 1.0, 1.0, 1.0, 1.0, 1.0, 1.0, 1.0, 1.0, 1.0, 1.0, 1.0, 1.0, 1.0, 1.0, 1.0, 1.0, 1.0, 1.0, 1.0, 1.0, 1.0, 1.0, 1.0, 1.0, 1.0, 1.0, 1.0, 1.0, 1.0, 1.0, 1.0, 1.0, 1.0, 1.0, 1.0, 1.0, 1.0, 1.0, 1.0, 1.0, 1.0, 1.0, 1.0, 1.0, 1.0, 1.0, 1.0, 1.0, 1.0, 1.0, 1.0, 1.0, 1.0, 1.0, 1.0, 1.0, 1.0, 1.0, 1.0, 1.0, 1.0, 1.0, 1.0, 1.0, 1.0, 1.0, 1.0, 1.0, 1.0, 1.0, 1.0, 1.0, 1.0, 1.0, 1.0, 1.0, 1.0, 1.0, 1.0, 1.0, 1.0, 1.0, 1.0, 1.0, 1.0, 1.0, 1.0, 1.0, 1.0, 1.0, 1.0, 1.0, 1.0, 1.0, 1.0, 1.0, 1.0, 1.0, 1.0, 1.0, 1.0, 1.0, 1.0, 1.0, 1.0, 1.0, 1.0, 1.0, 1.0, 1.0, 1.0, 1.0, 1.0, 1.0, 1.0, 1.0, 1.0, 1.0, 1.0, 1.0, 1.0, 1.0, 1.0, 1.0, 1.0, 1.0, 1.0, 1.0, 1.0, 1.0, 1.0, 1.0, 1.0, 1.0, 1.0, 1.0, 1.0, 1.0, 1.0, 1.0, 1.0, 1.0, 1.0, 1.0, 1.0, 1.0, 1.0, 1.0, 1.0, 1.0, 1.0, 1.0, 1.0, 1.0, 1.0, 1.0, 1.0, 1.0, 1.0, 1.0, 1.0, 1.0, 1.0, 1.0, 1.0, 1.0, 1.0, 1.0, 1.0, 1.0, 1.0, 1.0, 1.0, 1.0, 1.0, 1.0, 1.0, 1.0, 1.0, 1.0, 1.0, 1.0, 1.0, 1.0, 1.0, 1.0, 1.0, 1.0, 1.0, 1.0, 1.0, 1.0, 1.0, 1.0, 1.0, 1.0, 1.0, 1.0, 1.0, 1.0, 1.0, 1.0, 1.0, 1.0, 1.0, 1.0, 1.0, 1.0, 1.0, 1.0, 1.0, 1.0, 1.0, 1.0, 1.0, 1.0, 1.0, 1.0, 1.0, 1.0, 1.0, 1.0, 1.0, 1.0, 1.0, 1.0, 1.0, 1.0, 1.0, 1.0, 1.0, 1.0, 1.0, 1.0, 1.0, 1.0, 1.0, 1.0, 1.0, 1.0, 1.0, 1.0, 1.0, 1.0, 1.0, 1.0, 1.0, 1.0, 1.0, 1.0, 1.0, 1.0, 1.0, 1.0, 1.0, 1.0, 1.0, 1.0, 1.0, 1.0, 1.0, 1.0, 1.0, 1.0, 1.0, 1.0, 1.0, 1.0, 1.0, 1.0, 1.0, 1.0, 1.0, 1.0, 1.0, 1.0, 1.0, 1.0, 1.0, 1.0, 1.0, 1.0, 1.0, 1.0, 1.0, 1.0, 1.0, 1.0, 1.0, 1.0, 1.0, 1.0, 1.0, 1.0, 1.0, 1.0, 1.0, 1.0, 1.0, 1.0, 1.0, 1.0, 1.0, 1.0, 1.0, 1.0, 1.0, 1.0, 1.0, 1.0, 1.0, 1.0, 1.0, 1.0, 1.0, 1.0, 1.0, 1.0, 1.0, 1.0, 1.0, 1.0, 1.0, 1.0, 1.0, 1.0, 1.0, 1.0, 1.0, 1.0, 1.0, 1.0, 1.0, 1.0, 1.0, 1.0, 1.0, 1.0], "Y"=[0.0375, 0.075, 0.11249999999999999, 0.15, 0.1875, 0.225, 0.26249999999999996, 0.3, 0.33749999999999997, 0.37499999999999994, 0.4125, 0.44999999999999996, 0.48749999999999993, 0.525, 0.5625, 0.6, 0.6375, 0.6749999999999999, 0.7124999999999999, 0.75, 0.7875, 0.825, 0.8624999999999999, 0.8999999999999999, 0.9374999999999999, 0.975, 1.0125, 1.05, 1.0875000000000001, 1.125, 1.1625, 1.2, 1.2375, 1.2750000000000001, 1.3125, 1.35, 1.3875, 1.425, 1.4625000000000001, 1.5, 1.5375, 1.575, 1.6125, 1.6500000000000001, 1.6875, 1.725, 1.7625, 1.8, 1.8375, 1.875, 1.9125, 1.95, 1.9875, 2.025, 2.0625, 2.1, 2.1375, 2.175, 2.2125, 2.25, 2.2875, 2.325, 2.3625, 2.4, 2.4375, 2.475, 2.5125, 2.55, 2.5875, 2.625, 2.6625, 2.7, 2.7375, 2.775, 2.8125, 2.85, 2.8875, 2.925, 2.9625, 3.0, 3.0375, 3.075, 3.1125, 3.15, 3.1875, 3.225, 3.2625, 3.3, 3.3375, 3.375, 3.4125, 3.45, 3.4875, 3.525, 3.5625, 3.6, 3.6374999999999997, 3.675, 3.7125, 3.75, 3.7875, 3.8249999999999997, 3.8625, 3.9, 3.9375, 3.975, 4.012499999999999, 4.05, 4.0874999999999995, 4.124999999999999, 4.1625, 4.199999999999999, 4.2375, 4.2749999999999995, 4.312499999999999, 4.35, 4.387499999999999, 4.425, 4.4624999999999995, 4.499999999999999, 4.5375, 4.574999999999999, 4.6125, 4.6499999999999995, 4.687499999999999, 4.725, 4.762499999999999, 4.8, 4.8374999999999995, 4.874999999999999, 4.9125, 4.949999999999999, 4.9875, 5.0249999999999995, 5.062499999999999, 5.1, 5.137499999999999, 5.175, 5.2124999999999995, 5.249999999999999, 5.2875, 5.324999999999999, 5.3625, 5.3999999999999995, 5.437499999999999, 5.475, 5.512499999999999, 5.55, 5.5874999999999995, 5.624999999999999, 5.6625, 5.699999999999999, 5.7375, 5.7749999999999995, 5.812499999999999, 5.85, 5.887499999999999, 5.925, 5.9624999999999995, 5.999999999999999, 6.0375, 6.074999999999999, 6.1125, 6.1499999999999995, 6.187499999999999, 6.225, 6.262499999999999, 6.3, 6.3374999999999995, 6.374999999999999, 6.4125, 6.449999999999999, 6.4875, 6.5249999999999995, 6.562499999999999, 6.6, 6.637499999999999, 6.675, 6.7124999999999995, 6.749999999999999, 6.7875, 6.824999999999999, 6.8625, 6.8999999999999995, 6.937499999999999, 6.975, 7.012499999999999, 7.05, 7.0874999999999995, 7.124999999999999, 7.1625, 7.199999999999999, 7.237499999999999, 7.2749999999999995, 7.312499999999999, 7.35, 7.387499999999999, 7.424999999999999, 7.4624999999999995, 7.499999999999999, 7.5375, 7.574999999999999, 7.612499999999999, 7.6499999999999995, 7.687499999999999, 7.725, 7.762499999999999, 7.799999999999999, 7.8374999999999995, 7.874999999999999, 7.9125, 7.949999999999999, 7.987499999999999, 8.025, 8.0625, 8.1, 8.1375, 8.174999999999999, 8.212499999999999, 8.25, 8.2875, 8.325, 8.362499999999999, 8.399999999999999, 8.4375, 8.475, 8.5125, 8.549999999999999, 8.587499999999999, 8.625, 8.6625, 8.7, 8.737499999999999, 8.774999999999999, 8.8125, 8.85, 8.8875, 8.924999999999999, 8.962499999999999, 9.0, 9.0375, 9.075, 9.112499999999999, 9.149999999999999, 9.1875, 9.225, 9.2625, 9.299999999999999, 9.337499999999999, 9.375, 9.4125, 9.45, 9.487499999999999, 9.524999999999999, 9.5625, 9.6, 9.6375, 9.674999999999999, 9.712499999999999, 9.75, 9.7875, 9.825, 9.862499999999999, 9.899999999999999, 9.9375, 9.975, 10.0125, 10.049999999999999, 10.087499999999999, 10.125, 10.1625, 10.2, 10.237499999999999, 10.274999999999999, 10.3125, 10.35, 10.3875, 10.424999999999999, 10.462499999999999, 10.5, 10.5375, 10.575, 10.612499999999999, 10.649999999999999, 10.6875, 10.725, 10.7625, 10.799999999999999, 10.837499999999999, 10.875, 10.9125, 10.95, 10.987499999999999, 11.024999999999999, 11.0625, 11.1, 11.1375, 11.174999999999999, 11.212499999999999, 11.25, 11.2875, 11.325, 11.362499999999999, 11.399999999999999, 11.4375, 11.475, 11.5125, 11.549999999999999, 11.587499999999999, 11.625, 11.6625, 11.7, 11.737499999999999, 11.774999999999999, 11.8125, 11.85, 11.8875, 11.924999999999999, 11.962499999999999, 12.0, 12.0375, 12.075, 12.112499999999999, 12.149999999999999, 12.1875, 12.225, 12.2625, 12.299999999999999, 12.337499999999999, 12.375, 12.4125, 12.45, 12.487499999999999, 12.524999999999999, 12.5625, 12.6, 12.6375, 12.674999999999999, 12.712499999999999, 12.75, 12.7875, 12.825, 12.862499999999999, 12.899999999999999, 12.9375, 12.975, 13.0125, 13.049999999999999, 13.087499999999999, 13.125, 13.1625, 13.2, 13.237499999999999, 13.274999999999999, 13.3125, 13.35, 13.3875, 13.424999999999999, 13.462499999999999, 13.5, 13.5375, 13.575, 13.612499999999999, 13.649999999999999, 13.6875, 13.725, 13.7625, 13.799999999999999, 13.837499999999999, 13.875, 13.9125, 13.95, 13.987499999999999, 14.024999999999999, 14.0625, 14.1, 14.1375, 14.174999999999999, 14.212499999999999, 14.25, 14.2875, 14.325, 14.362499999999999, 14.399999999999999, 14.437499999999998, 14.475, 14.5125, 14.549999999999999, 14.587499999999999, 14.624999999999998, 14.6625, 14.7, 14.737499999999999, 14.774999999999999, 14.812499999999998, 14.85, 14.8875, 14.924999999999999, 14.962499999999999, 14.999999999999998, 15.0375, 15.075, 15.112499999999999, 15.149999999999999, 15.187499999999998, 15.225, 15.2625, 15.299999999999999, 15.337499999999999, 15.374999999999998, 15.4125, 15.45, 15.487499999999999, 15.524999999999999, 15.562499999999998, 15.6, 15.6375, 15.674999999999999, 15.712499999999999, 15.749999999999998, 15.7875, 15.825, 15.862499999999999, 15.899999999999999, 15.937499999999998, 15.975, 16.0125, 16.05, 16.087500000000002, 16.125, 16.1625, 16.2, 16.2375, 16.275000000000002, 16.3125, 16.35, 16.3875, 16.425, 16.462500000000002, 16.5, 16.5375, 16.575, 16.6125, 16.650000000000002, 16.6875, 16.725, 16.7625, 16.8, 16.837500000000002, 16.875, 16.9125, 16.95, 16.9875, 17.025000000000002, 17.0625, 17.1, 17.1375, 17.175, 17.212500000000002, 17.25, 17.2875, 17.325, 17.3625, 17.400000000000002, 17.4375, 17.475, 17.5125, 17.55, 17.587500000000002, 17.625, 17.6625, 17.7, 17.7375, 17.775000000000002, 17.8125, 17.85, 17.8875, 17.925, 17.962500000000002, 18.0, 18.0375, 18.075, 18.1125, 18.150000000000002, 18.1875, 18.225, 18.2625, 18.3, 18.337500000000002, 18.375, 18.4125, 18.45, 18.4875, 18.525000000000002, 18.5625, 18.6, 18.6375, 18.675, 18.712500000000002, 18.75, 18.7875, 18.825, 18.8625, 18.900000000000002, 18.9375, 18.975, 19.0125, 19.05, 19.087500000000002, 19.125, 19.1625, 19.2, 19.2375, 19.275000000000002, 19.3125, 19.35, 19.3875, 19.425, 19.462500000000002, 19.5, 19.5375, 19.575, 19.6125, 19.650000000000002, 19.6875, 19.725, 19.7625, 19.8, 19.837500000000002, 19.875, 19.9125, 19.95, 19.9875, 20.025000000000002, 20.0625, 20.1, 20.1375, 20.175, 20.212500000000002, 20.25, 20.2875, 20.325, 20.3625, 20.400000000000002, 20.4375, 20.475, 20.5125, 20.55, 20.587500000000002, 20.625, 20.6625, 20.7, 20.7375, 20.775000000000002, 20.8125, 20.85, 20.8875, 20.925, 20.962500000000002, 21.0]}, ...(2 in all)]
  in  "dead time":dbl=3.7e-08
  out "CH1 RingBuffer long":dbl[][](array[numeric])
  out "CH1 RingBuffer short":dbl[][](array[numeric])
  in  "Weather":T3(tab)
  out "Temperature (C)":dbl(graph)=20.11660561660561
  out "Pressure (mb)":dbl(graph)=837.7335164835165
  out "Relative Humdity (%)":dbl(graph)=12.50152625152625
  out "Pulse Energy (Micro Joule)":T4(graph)={"Online Pulse Energy"=0.010624231428571426, "Pulse Energy Offline"=0.010612541428571428}
  out "?":cluster{"mean":dbl, "mean":dbl}(graph)={"mean"=0.0, "mean"=1404169.4084704237}
  out "Index":i32=111
  out "CH1 (WV off) smooth L":dbl[](array[numeric])
  out "CH1  Bin Readings":dbl[](array[numeric])
  out "CH1 (WV off) smooth S":dbl[](array[numeric])
  out "CH0 (WV on) smoothed":dbl[](array[numeric])
  out "CH 0 Bin Readings":dbl[](array[numeric])
  out "Range Corrected Altitude Array":dbl[](array[numeric])=[1406.25, 5625.0, 12656.25, 22500.0, 35156.25, 50625.0, 68906.25, 90000.0, 113906.25, 140625.0, 170156.25, 202500.0, 237656.25, 275625.0, 316406.25, 360000.0, 406406.25, 455625.0, 507656.25, 562500.0, 620156.25, 680625.0, 743906.25, 810000.0, 878906.25, 950625.0, 1025156.25, 1102500.0, 1182656.25, 1265625.0, 1351406.25, 1440000.0, 1531406.25, 1625625.0, 1722656.25, 1822500.0, 1925156.25, 2030625.0, 2138906.25, 2250000.0, 2363906.25, 2480625.0, 2600156.25, 2722500.0, 2847656.25, 2975625.0, 3106406.25, 3240000.0, 3376406.25, 3515625.0, 3657656.25, 3802500.0, 3950156.25, 4100625.0, 4253906.25, 4410000.0, 4568906.25, 4730625.0, 4895156.25, 5062500.0, 5232656.25, 5405625.0, 5581406.25, 5760000.0, 5941406.25, 6125625.0, 6312656.25, 6502500.0, 6695156.25, 6890625.0, 7088906.25, 7290000.0, 7493906.25, 7700625.0, 7910156.25, 8122500.0, 8337656.25, 8555625.0, 8776406.25, 9000000.0, 9226406.25, 9455625.0, 9687656.25, 9922500.0, 10160156.25, 10400625.0, 10643906.25, 10890000.0, 11138906.25, 11390625.0, 11645156.25, 11902500.0, 12162656.25, 12425625.0, 12691406.25, 12960000.0, 13231406.25, 13505625.0, 13782656.25, 14062500.0, 14345156.25, 14630625.0, 14918906.25, 15210000.0, 15503906.25, 15800625.0, 16100156.25, 16402500.0, 16707656.25, 17015625.0, 17326406.25, 17640000.0, 17956406.25, 18275625.0, 18597656.25, 18922500.0, 19250156.25, 19580625.0, 19913906.25, 20250000.0, 20588906.25, 20930625.0, 21275156.25, 21622500.0, 21972656.25, 22325625.0, 22681406.25, 23040000.0, 23401406.25, 23765625.0, 24132656.25, 24502500.0, 24875156.25, 25250625.0, 25628906.25, 26010000.0, 26393906.25, 26780625.0, 27170156.25, 27562500.0, 27957656.25, 28355625.0, 28756406.25, 29160000.0, 29566406.25, 29975625.0, 30387656.25, 30802500.0, 31220156.25, 31640625.0, 32063906.25, 32490000.0, 32918906.25, 33350625.0, 33785156.25, 34222500.0, 34662656.25, 35105625.0, 35551406.25, 36000000.0, 36451406.25, 36905625.0, 37362656.25, 37822500.0, 38285156.25, 38750625.0, 39218906.25, 39690000.0, 40163906.25, 40640625.0, 41120156.25, 41602500.0, 42087656.25, 42575625.0, 43066406.25, 43560000.0, 44056406.25, 44555625.0, 45057656.25, 45562500.0, 46070156.25, 46580625.0, 47093906.25, 47610000.0, 48128906.25, 48650625.0, 49175156.25, 49702500.0, 50232656.25, 50765625.0, 51301406.25, 51840000.0, 52381406.25, 52925625.0, 53472656.25, 54022500.0, 54575156.25, 55130625.0, 55688906.25, 56250000.0, 56813906.25, 57380625.0, 57950156.25, 58522500.0, 59097656.25, 59675625.0, 60256406.25, 60840000.0, 61426406.25, 62015625.0, 62607656.25, 63202500.0, 63800156.25, 64400625.0, 65003906.25, 65610000.0, 66218906.25, 66830625.0, 67445156.25, 68062500.0, 68682656.25, 69305625.0, 69931406.25, 70560000.0, 71191406.25, 71825625.0, 72462656.25, 73102500.0, 73745156.25, 74390625.0, 75038906.25, 75690000.0, 76343906.25, 77000625.0, 77660156.25, 78322500.0, 78987656.25, 79655625.0, 80326406.25, 81000000.0, 81676406.25, 82355625.0, 83037656.25, 83722500.0, 84410156.25, 85100625.0, 85793906.25, 86490000.0, 87188906.25, 87890625.0, 88595156.25, 89302500.0, 90012656.25, 90725625.0, 91441406.25, 92160000.0, 92881406.25, 93605625.0, 94332656.25, 95062500.0, 95795156.25, 96530625.0, 97268906.25, 98010000.0, 98753906.25, 99500625.0, 100250156.25, 101002500.0, 101757656.25, 102515625.0, 103276406.25, 104040000.0, 104806406.25, 105575625.0, 106347656.25, 107122500.0, 107900156.25, 108680625.0, 109463906.25, 110250000.0, 111038906.25, 111830625.0, 112625156.25, 113422500.0, 114222656.25, 115025625.0, 115831406.25, 116640000.0, 117451406.25, 118265625.0, 119082656.25, 119902500.0, 120725156.25, 121550625.0, 122378906.25, 123210000.0, 124043906.25, 124880625.0, 125720156.25, 126562500.0, 127407656.25, 128255625.0, 129106406.25, 129960000.0, 130816406.25, 131675625.0, 132537656.25, 133402500.0, 134270156.25, 135140625.0, 136013906.25, 136890000.0, 137768906.25, 138650625.0, 139535156.25, 140422500.0, 141312656.25, 142205625.0, 143101406.25, 144000000.0, 144901406.25, 145805625.0, 146712656.25, 147622500.0, 148535156.25, 149450625.0, 150368906.25, 151290000.0, 152213906.25, 153140625.0, 154070156.25, 155002500.0, 155937656.25, 156875625.0, 157816406.25, 158760000.0, 159706406.25, 160655625.0, 161607656.25, 162562500.0, 163520156.25, 164480625.0, 165443906.25, 166410000.0, 167378906.25, 168350625.0, 169325156.25, 170302500.0, 171282656.25, 172265625.0, 173251406.25, 174240000.0, 175231406.25, 176225625.0, 177222656.25, 178222500.0, 179225156.25, 180230625.0, 181238906.25, 182250000.0, 183263906.25, 184280625.0, 185300156.25, 186322500.0, 187347656.25, 188375625.0, 189406406.25, 190440000.0, 191476406.25, 192515625.0, 193557656.25, 194602500.0, 195650156.25, 196700625.0, 197753906.25, 198810000.0, 199868906.25, 200930625.0, 201995156.25, 203062500.0, 204132656.25, 205205625.0, 206281406.25, 207360000.0, 208441406.25, 209525625.0, 210612656.25, 211702500.0, 212795156.25, 213890625.0, 214988906.25, 216090000.0, 217193906.25, 218300625.0, 219410156.25, 220522500.0, 221637656.25, 222755625.0, 223876406.25, 225000000.0, 226126406.25, 227255625.0, 228387656.25, 229522500.0, 230660156.25, 231800625.0, 232943906.25, 234090000.0, 235238906.25, 236390625.0, 237545156.25, 238702500.0, 239862656.25, 241025625.0, 242191406.25, 243360000.0, 244531406.25, 245705625.0, 246882656.25, 248062500.0, 249245156.25, 250430625.0, 251618906.25, 252810000.0, 254003906.25, 255200625.0, 256400156.25, 257602500.0, 258807656.25, 260015625.0, 261226406.25, 262440000.0, 263656406.25, 264875625.0, 266097656.25, 267322500.0, 268550156.25, 269780625.0, 271013906.25, 272250000.0, 273488906.25, 274730625.0, 275975156.25, 277222500.0, 278472656.25, 279725625.0, 280981406.25, 282240000.0, 283501406.25, 284765625.0, 286032656.25, 287302500.0, 288575156.25, 289850625.0, 291128906.25, 292410000.0, 293693906.25, 294980625.0, 296270156.25, 297562500.0, 298857656.25, 300155625.0, 301456406.25, 302760000.0, 304066406.25, 305375625.0, 306687656.25, 308002500.0, 309320156.25, 310640625.0, 311963906.25, 313290000.0, 314618906.25, 315950625.0, 317285156.25, 318622500.0, 319962656.25, 321305625.0, 322651406.25, 324000000.0, 325351406.25, 326705625.0, 328062656.25, 329422500.0, 330785156.25, 332150625.0, 333518906.25, 334890000.0, 336263906.25, 337640625.0, 339020156.25, 340402500.0, 341787656.25, 343175625.0, 344566406.25, 345960000.0, 347356406.25, 348755625.0, 350157656.25, 351562500.0, 352970156.25, 354380625.0, 355793906.25, 357210000.0, 358628906.25, 360050625.0, 361475156.25, 362902500.0, 364332656.25, 365765625.0, 367201406.25, 368640000.0, 370081406.25, 371525625.0, 372972656.25, 374422500.0, 375875156.25, 377330625.0, 378788906.25, 380250000.0, 381713906.25, 383180625.0, 384650156.25, 386122500.0, 387597656.25, 389075625.0, 390556406.25, 392040000.0, 393526406.25, 395015625.0, 396507656.25, 398002500.0, 399500156.25, 401000625.0, 402503906.25, 404010000.0, 405518906.25, 407030625.0, 408545156.25, 410062500.0, 411582656.25, 413105625.0, 414631406.25, 416160000.0, 417691406.25, 419225625.0, 420762656.25, 422302500.0, 423845156.25, 425390625.0, 426938906.25, 428490000.0, 430043906.25, 431600625.0, 433160156.25, 434722500.0, 436287656.25, 437855625.0, 439426406.25, 441000000.0]
  out "Altitude Array (km)":dbl[](array[numeric])=[0.0375, 0.075, 0.11249999999999999, 0.15, 0.1875, 0.225, 0.26249999999999996, 0.3, 0.33749999999999997, 0.37499999999999994, 0.4125, 0.44999999999999996, 0.48749999999999993, 0.525, 0.5625, 0.6, 0.6375, 0.6749999999999999, 0.7124999999999999, 0.75, 0.7875, 0.825, 0.8624999999999999, 0.8999999999999999, 0.9374999999999999, 0.975, 1.0125, 1.05, 1.0875000000000001, 1.125, 1.1625, 1.2, 1.2375, 1.2750000000000001, 1.3125, 1.35, 1.3875, 1.425, 1.4625000000000001, 1.5, 1.5375, 1.575, 1.6125, 1.6500000000000001, 1.6875, 1.725, 1.7625, 1.8, 1.8375, 1.875, 1.9125, 1.95, 1.9875, 2.025, 2.0625, 2.1, 2.1375, 2.175, 2.2125, 2.25, 2.2875, 2.325, 2.3625, 2.4, 2.4375, 2.475, 2.5125, 2.55, 2.5875, 2.625, 2.6625, 2.7, 2.7375, 2.775, 2.8125, 2.85, 2.8875, 2.925, 2.9625, 3.0, 3.0375, 3.075, 3.1125, 3.15, 3.1875, 3.225, 3.2625, 3.3, 3.3375, 3.375, 3.4125, 3.45, 3.4875, 3.525, 3.5625, 3.6, 3.6374999999999997, 3.675, 3.7125, 3.75, 3.7875, 3.8249999999999997, 3.8625, 3.9, 3.9375, 3.975, 4.012499999999999, 4.05, 4.0874999999999995, 4.124999999999999, 4.1625, 4.199999999999999, 4.2375, 4.2749999999999995, 4.312499999999999, 4.35, 4.387499999999999, 4.425, 4.4624999999999995, 4.499999999999999, 4.5375, 4.574999999999999, 4.6125, 4.6499999999999995, 4.687499999999999, 4.725, 4.762499999999999, 4.8, 4.8374999999999995, 4.874999999999999, 4.9125, 4.949999999999999, 4.9875, 5.0249999999999995, 5.062499999999999, 5.1, 5.137499999999999, 5.175, 5.2124999999999995, 5.249999999999999, 5.2875, 5.324999999999999, 5.3625, 5.3999999999999995, 5.437499999999999, 5.475, 5.512499999999999, 5.55, 5.5874999999999995, 5.624999999999999, 5.6625, 5.699999999999999, 5.7375, 5.7749999999999995, 5.812499999999999, 5.85, 5.887499999999999, 5.925, 5.9624999999999995, 5.999999999999999, 6.0375, 6.074999999999999, 6.1125, 6.1499999999999995, 6.187499999999999, 6.225, 6.262499999999999, 6.3, 6.3374999999999995, 6.374999999999999, 6.4125, 6.449999999999999, 6.4875, 6.5249999999999995, 6.562499999999999, 6.6, 6.637499999999999, 6.675, 6.7124999999999995, 6.749999999999999, 6.7875, 6.824999999999999, 6.8625, 6.8999999999999995, 6.937499999999999, 6.975, 7.012499999999999, 7.05, 7.0874999999999995, 7.124999999999999, 7.1625, 7.199999999999999, 7.237499999999999, 7.2749999999999995, 7.312499999999999, 7.35, 7.387499999999999, 7.424999999999999, 7.4624999999999995, 7.499999999999999, 7.5375, 7.574999999999999, 7.612499999999999, 7.6499999999999995, 7.687499999999999, 7.725, 7.762499999999999, 7.799999999999999, 7.8374999999999995, 7.874999999999999, 7.9125, 7.949999999999999, 7.987499999999999, 8.025, 8.0625, 8.1, 8.1375, 8.174999999999999, 8.212499999999999, 8.25, 8.2875, 8.325, 8.362499999999999, 8.399999999999999, 8.4375, 8.475, 8.5125, 8.549999999999999, 8.587499999999999, 8.625, 8.6625, 8.7, 8.737499999999999, 8.774999999999999, 8.8125, 8.85, 8.8875, 8.924999999999999, 8.962499999999999, 9.0, 9.0375, 9.075, 9.112499999999999, 9.149999999999999, 9.1875, 9.225, 9.2625, 9.299999999999999, 9.337499999999999, 9.375, 9.4125, 9.45, 9.487499999999999, 9.524999999999999, 9.5625, 9.6, 9.6375, 9.674999999999999, 9.712499999999999, 9.75, 9.7875, 9.825, 9.862499999999999, 9.899999999999999, 9.9375, 9.975, 10.0125, 10.049999999999999, 10.087499999999999, 10.125, 10.1625, 10.2, 10.237499999999999, 10.274999999999999, 10.3125, 10.35, 10.3875, 10.424999999999999, 10.462499999999999, 10.5, 10.5375, 10.575, 10.612499999999999, 10.649999999999999, 10.6875, 10.725, 10.7625, 10.799999999999999, 10.837499999999999, 10.875, 10.9125, 10.95, 10.987499999999999, 11.024999999999999, 11.0625, 11.1, 11.1375, 11.174999999999999, 11.212499999999999, 11.25, 11.2875, 11.325, 11.362499999999999, 11.399999999999999, 11.4375, 11.475, 11.5125, 11.549999999999999, 11.587499999999999, 11.625, 11.6625, 11.7, 11.737499999999999, 11.774999999999999, 11.8125, 11.85, 11.8875, 11.924999999999999, 11.962499999999999, 12.0, 12.0375, 12.075, 12.112499999999999, 12.149999999999999, 12.1875, 12.225, 12.2625, 12.299999999999999, 12.337499999999999, 12.375, 12.4125, 12.45, 12.487499999999999, 12.524999999999999, 12.5625, 12.6, 12.6375, 12.674999999999999, 12.712499999999999, 12.75, 12.7875, 12.825, 12.862499999999999, 12.899999999999999, 12.9375, 12.975, 13.0125, 13.049999999999999, 13.087499999999999, 13.125, 13.1625, 13.2, 13.237499999999999, 13.274999999999999, 13.3125, 13.35, 13.3875, 13.424999999999999, 13.462499999999999, 13.5, 13.5375, 13.575, 13.612499999999999, 13.649999999999999, 13.6875, 13.725, 13.7625, 13.799999999999999, 13.837499999999999, 13.875, 13.9125, 13.95, 13.987499999999999, 14.024999999999999, 14.0625, 14.1, 14.1375, 14.174999999999999, 14.212499999999999, 14.25, 14.2875, 14.325, 14.362499999999999, 14.399999999999999, 14.437499999999998, 14.475, 14.5125, 14.549999999999999, 14.587499999999999, 14.624999999999998, 14.6625, 14.7, 14.737499999999999, 14.774999999999999, 14.812499999999998, 14.85, 14.8875, 14.924999999999999, 14.962499999999999, 14.999999999999998, 15.0375, 15.075, 15.112499999999999, 15.149999999999999, 15.187499999999998, 15.225, 15.2625, 15.299999999999999, 15.337499999999999, 15.374999999999998, 15.4125, 15.45, 15.487499999999999, 15.524999999999999, 15.562499999999998, 15.6, 15.6375, 15.674999999999999, 15.712499999999999, 15.749999999999998, 15.7875, 15.825, 15.862499999999999, 15.899999999999999, 15.937499999999998, 15.975, 16.0125, 16.05, 16.087500000000002, 16.125, 16.1625, 16.2, 16.2375, 16.275000000000002, 16.3125, 16.35, 16.3875, 16.425, 16.462500000000002, 16.5, 16.5375, 16.575, 16.6125, 16.650000000000002, 16.6875, 16.725, 16.7625, 16.8, 16.837500000000002, 16.875, 16.9125, 16.95, 16.9875, 17.025000000000002, 17.0625, 17.1, 17.1375, 17.175, 17.212500000000002, 17.25, 17.2875, 17.325, 17.3625, 17.400000000000002, 17.4375, 17.475, 17.5125, 17.55, 17.587500000000002, 17.625, 17.6625, 17.7, 17.7375, 17.775000000000002, 17.8125, 17.85, 17.8875, 17.925, 17.962500000000002, 18.0, 18.0375, 18.075, 18.1125, 18.150000000000002, 18.1875, 18.225, 18.2625, 18.3, 18.337500000000002, 18.375, 18.4125, 18.45, 18.4875, 18.525000000000002, 18.5625, 18.6, 18.6375, 18.675, 18.712500000000002, 18.75, 18.7875, 18.825, 18.8625, 18.900000000000002, 18.9375, 18.975, 19.0125, 19.05, 19.087500000000002, 19.125, 19.1625, 19.2, 19.2375, 19.275000000000002, 19.3125, 19.35, 19.3875, 19.425, 19.462500000000002, 19.5, 19.5375, 19.575, 19.6125, 19.650000000000002, 19.6875, 19.725, 19.7625, 19.8, 19.837500000000002, 19.875, 19.9125, 19.95, 19.9875, 20.025000000000002, 20.0625, 20.1, 20.1375, 20.175, 20.212500000000002, 20.25, 20.2875, 20.325, 20.3625, 20.400000000000002, 20.4375, 20.475, 20.5125, 20.55, 20.587500000000002, 20.625, 20.6625, 20.7, 20.7375, 20.775000000000002, 20.8125, 20.85, 20.8875, 20.925, 20.962500000000002, 21.0]
  out "Offline Pulse Energy":dbl=0.010639517142857142
  out "Online Pulse Energy":dbl=0.010624231428571426
  in  "Instrument Control":T5(tab)=enum."Wavemeter"
  in  "Device In":refnum<visa-resource-name>="Pro8000"
  in  "Settings":T6={"Module"=enum."WV Online TEC", "WV Online TEC"=14.177149999999989, "WV Online LD"=0.16, "WV Offline TEC"=29.53825, "WV Offline LD"=0.16, "WV Etalon TEC"=30.0, "HSRL Etalon TEC"=18.9999638, "HSRL TEC"=14.172, "HSRL LD"=0.16} {"HSRL LD" min=0.0 max=0.18 step=0.001 format="%.3p"; "HSRL TEC" min=14.0 max=28.0 step=0.1 format="%.3g"; "WV Offline LD" min=0.0 max=0.18 step=0.001 format="%.3p"; "WV Online LD" min=0.0 max=0.18 step=0.001 format="%.3p"; "HSRL Etalon TEC" format="%.2g"; "WV Etalon TEC" format="%.2g"; "WV Offline TEC" min=16.0 max=30.0 step=0.1 format="%.3g"; "WV Online TEC" min=14.0 max=28.0 step=0.1 format="%.3g"}
  out "Readings":T7={"Pro8000"=TRUE, "WV OnLine TEC"=14.1784306, "WV Online TEC"=TRUE, "WV Online LD"=0.160609379, "WV Online LD"=TRUE, "WV Offline TEC"=23.4319096, "WV Offline TEC"=FALSE, "WV Offline LD"=0.00020117189, "WV Offline LD"=FALSE, "WV EtalonTEC"=30.0249977, "WV Etalon TEC"=TRUE, "HSRL Etalon TEC"=9.51464272, "HSRL Etalon TEC"=FALSE, "HSRL TEC"=-12.375, "HSRL TEC "=FALSE, "HSRL LD"=0.0, "HSRL LD"=FALSE} {"HSRL LD" format="%.3p"; "HSRL TEC" format="%.3g"; "WV Offline LD" format="%.3p"; "WV Online LD" format="%.3p"; "HSRL Etalon TEC" format="%.3g"; "WV EtalonTEC" format="%.3g"; "WV Offline TEC" format="%.3g"; "WV OnLine TEC" format="%.3g"}
  in  "Pulse B Polarity":enum32{"Low", "High"}(ring)=enum."High"
  in  "Pulse A Delay(ns)":u32=1040 min=80 max=327600
  in  "Pulse B Delay(ns)":u32=170000 min=80 max=327600 step=1
  in  "Accumulation Delay(ns)":u32=10 min=10 max=1270 step=1
  in  "Sync Pulse Polarity":enum32{"Low", "High"}(ring)=enum."High"
  in  "Pulse A Polarity":enum32{"Low", "High"}(ring)=enum."High"
  in  "Number of Bins":u32=560 min=2 max=4095 step=1
  in  "Number of Accumulates":u32=14285 min=1 max=32767 step=1
  in  "Time Resolution Per Bin(ns)":u32=250 min=5 max=1063 step=1
  out "AMCS_Profile":i32=137
  in  "WV Online Set (nm)":dbl=780.24612 format="%.5f"
  out "WV Online Read (nm)":dbl=780.2461193940377 format="%.5f"
  out "WV Offline Read (nm)":dbl=780.2461227054038 format="%.5f"
  in  "WV Offline Set (nm)":dbl=780.24612 format="%#.5f"
  in  "Bristol In":i32=5
  out "Bristol Out":i32
  out "WL_Difference":dbl=-6.059623274268233e-07 format="%#_3e"
  out "WL Difference off":dbl=2.7054037445850554e-06 format="%#_3e"
  out "Wavelength Lock Online":bool=TRUE
  out "Wavelength Lock Offline":bool=TRUE
  in  "calculate absorption cross sections":bool
  in  "Online_Tol":dbl=5e-05 format="%#_15g"
  in  "Cancel online":bool
  in  "Offline_Tol":dbl=0.001 format="%#_15g"
  in  "Cancel Offline":bool
  in  "y":dbl=0.00025 format="%#_6p"
  in  "Smoothing Range":dbl=150.0
  in  "Total DIAL Integration Time (Minutes)":i32=3
  in  "Data Reads (number of loops)":i32=1
  in  "Total Aerosol Integration Time (Minutes)":dbl=0.5
  in  "Scalar Wait Time":u32
  out "Smoothed Bins":dbl=4.0
  in  "NewportIn":string
  in  "logging":bool
  out "Newport Device Key":string="1918-R 15120"
  in  "SampleSize":i32=2
  out "NewportRef":refnum<k24>
  in  "Switch Comm Port":refnum<visa-resource-name>="COM3"
  out "FF_On_Ref":refnum<file>
  out "FF_On_Ptr":i64=502608 format="%.2p"
  out "FF_Off_Ref":refnum<file>
  out "FF_Off_Ptr":i64=502608 format="%.2p"
  out "NF_On_Ref":refnum<file>
  out "NF_On_Ptr":i64=502608 format="%.2p"
  out "NF_Off_Ref":refnum<file>
  out "NF_Off_Ptr":i64=502608 format="%.2p"
  out "DataOpen":bool=TRUE
  out "File Path_Far Field (out)":string="C:\\Users\\H2ODial\\Desktop\\SharedTeleWVData\\170309FF\\21"
  out "File Path_Near Field (out)":string="C:\\Users\\H2ODial\\Desktop\\SharedTeleWVData\\170309NF\\21"
  in  "Data File DIR (in)":string="C:\\Users\\H2ODial\\Desktop\\SharedTeleWVData\\"
  out "TRHP":T8={"Temp C"=20.11660561660561, "RelH %"=12.50152625152625, "Press hPa"=837.7335164835165, "AbH g/m^3"=2.1062271062271063}
  in  "WS visa":refnum<visa-resource-name>="LuftWS"
  in  "WS_On/Off":bool=TRUE
  in  "bins":u32=560 min=2 max=4095 step=1
  out "y offset":u32=10
  in  "ns scale":u32=250
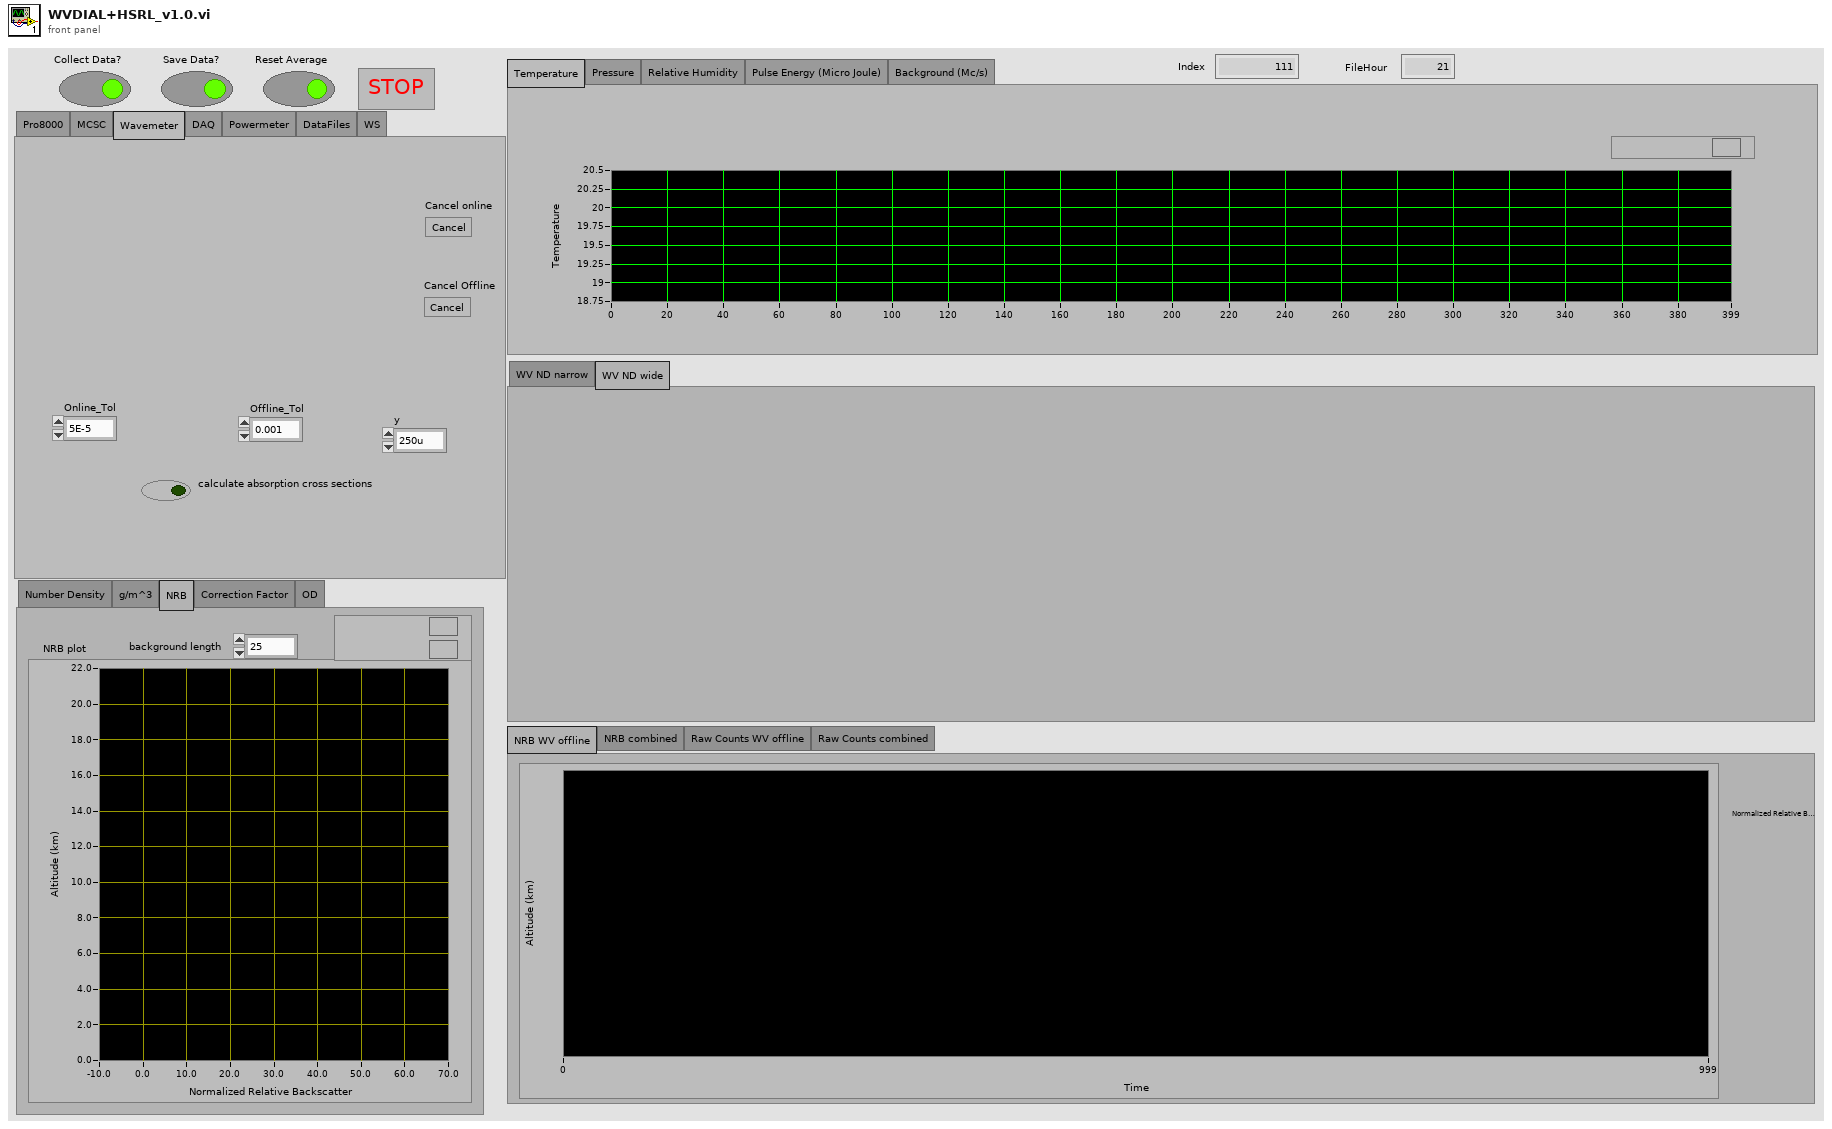
[diagram p1: front panel]
types:
  T1 = enum32{"NRB WV offline", "NRB combined", "Raw Counts WV offline", "Raw Counts combined"}
  T2 = enum32{"Number Density", "g/m^3", "NRB", "Correction Factor", "OD"}
  T3 = enum32{"Temperature", "Pressure", "Relative Humidity", "Pulse Energy (Micro Joule)", "Background (Mc/s)"}
  T4 = cluster{"Online Pulse Energy":dbl, "Pulse Energy Offline":dbl}
  T5 = enum32{"Pro8000", "MCSC", "Wavemeter", "DAQ", "Powermeter", "DataFiles", "WS"}
  T6 = cluster{"Module":enum16{"WV Online TEC", "WV Online LD", "WV Offline TEC", "WV Offline LD", "WV Etalon TEC", "HSRL Etalon TEC", "HSRL TEC", "HSRL LD"}, "WV Online TEC":dbl, "WV Online LD":dbl, "WV Offline TEC":dbl, "WV Offline LD":dbl, "WV Etalon TEC":dbl, "HSRL Etalon TEC":dbl, "HSRL TEC":dbl, "HSRL LD":dbl}
  T7 = cluster{"Pro8000":bool, "WV OnLine TEC":dbl, "WV Online TEC":bool, "WV Online LD":dbl, "WV Online LD":bool, "WV Offline TEC":dbl, "WV Offline TEC":bool, "WV Offline LD":dbl, "WV Offline LD":bool, "WV EtalonTEC":dbl, "WV Etalon TEC":bool, "HSRL Etalon TEC":dbl, "HSRL Etalon TEC":bool, "HSRL TEC":dbl, "HSRL TEC ":bool, "HSRL LD":dbl, "HSRL LD":bool}
  T8 = cluster{"Temp C":dbl, "RelH %":dbl, "Press hPa":dbl, "AbH g/m^3":dbl}
  T9 = enum16{"Open_TL", "Close_TL", "Verify_ID", "TEC_Sensor", "SET", "READ", "ON", "OFF", "Set_Limits", "Read_Limits", "Enable_Status", "Read_Status"}
  T10 = enum16{"Initialize ILX", "Set ON T", "Set Off T", "Set ON I", "Set Off I", "Set On Lim", "Set Off Lim", "Read ILX", "TEC ON/OFF", "LASER ON/OFF", "Status?", "ILX OFF"}
  T11 = enum16{"open", "replace", "create", "open or create", "replace or create", "replace or create with confirmation"}
  T12 = enum16{"WV Online TEC", "WV Online LD", "WV Offline TEC", "WV Offline LD", "WV Etalon TEC", "HSRL Etalon TEC", "HSRL TEC", "HSRL LD"}
  T13 = cluster{"Temp":dbl, "RelH":dbl, "Press":dbl, "AbH":dbl}
  T14 = typedef "LVDateTimeRec.ctl" = cluster{"fractional second":dbl, "second":i32, "minute":i32, "hour":i32, "day of month":i32, "month":i32, "year":i32, "day of week":i32, "day of year":i32, "DST":i32}
  T15 = cluster{"Online Pulse Energy":dbl, "Offline Pulse Energy":dbl}
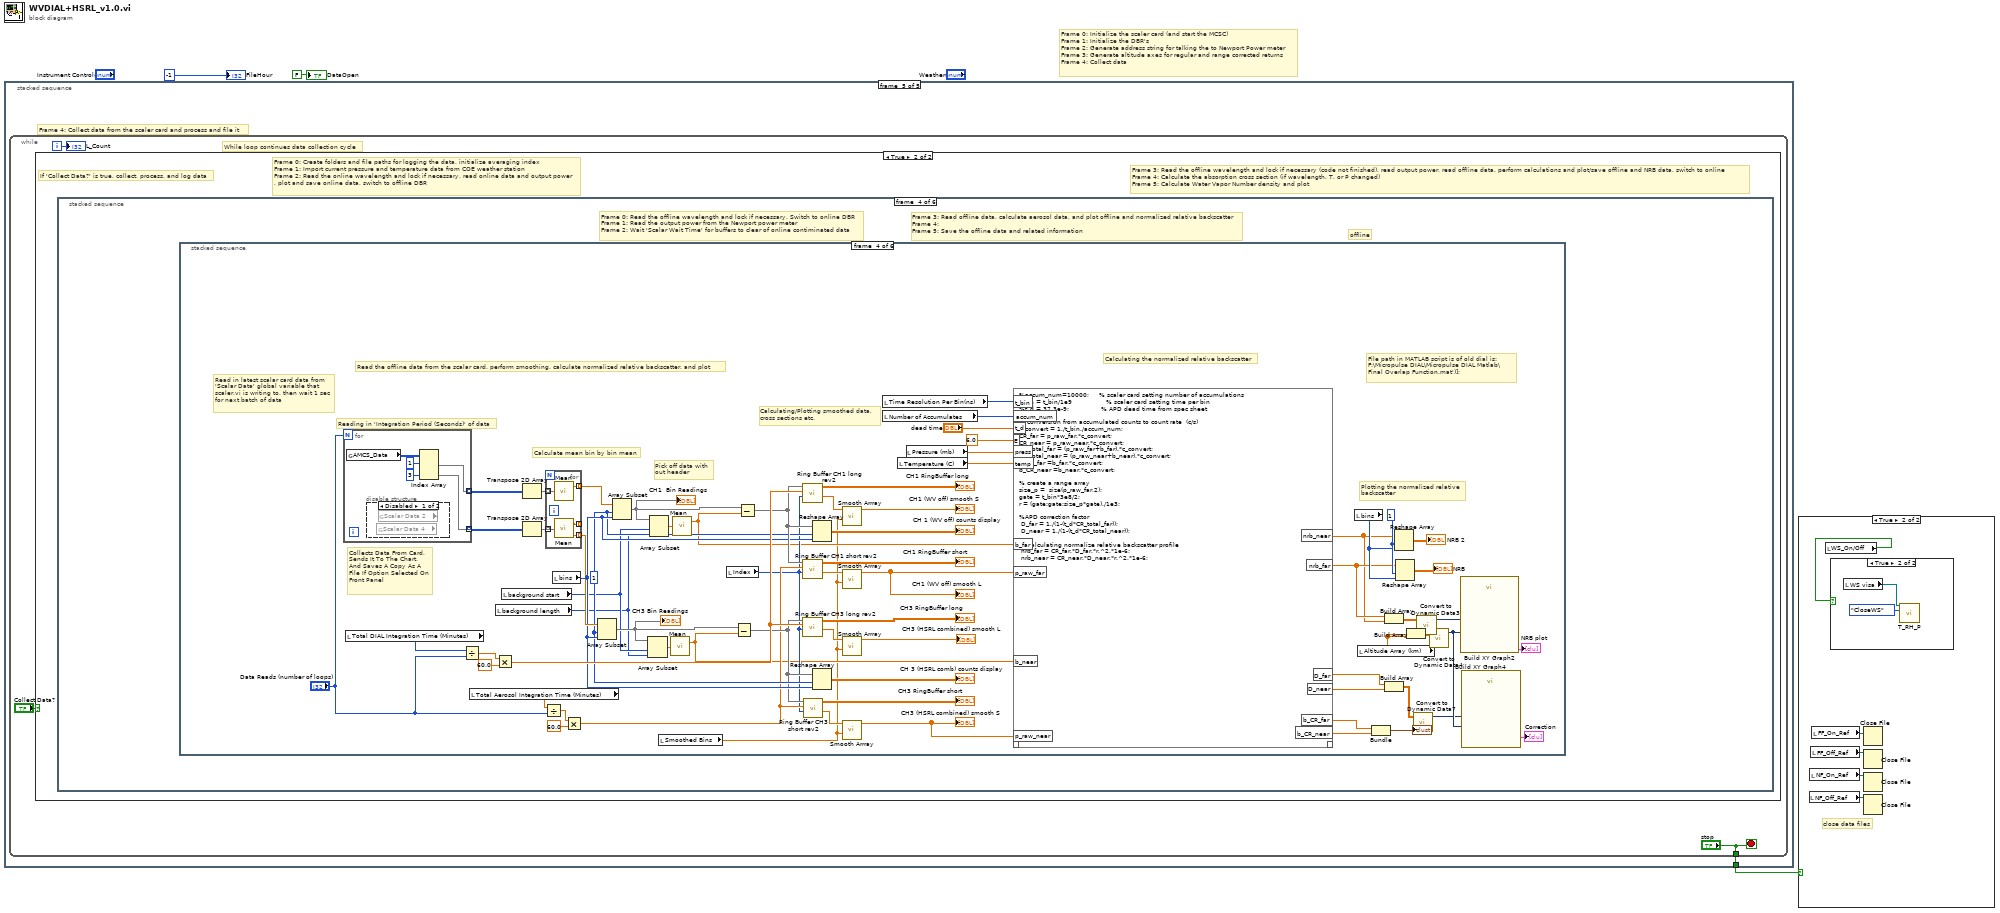
[diagram p0: block diagram]
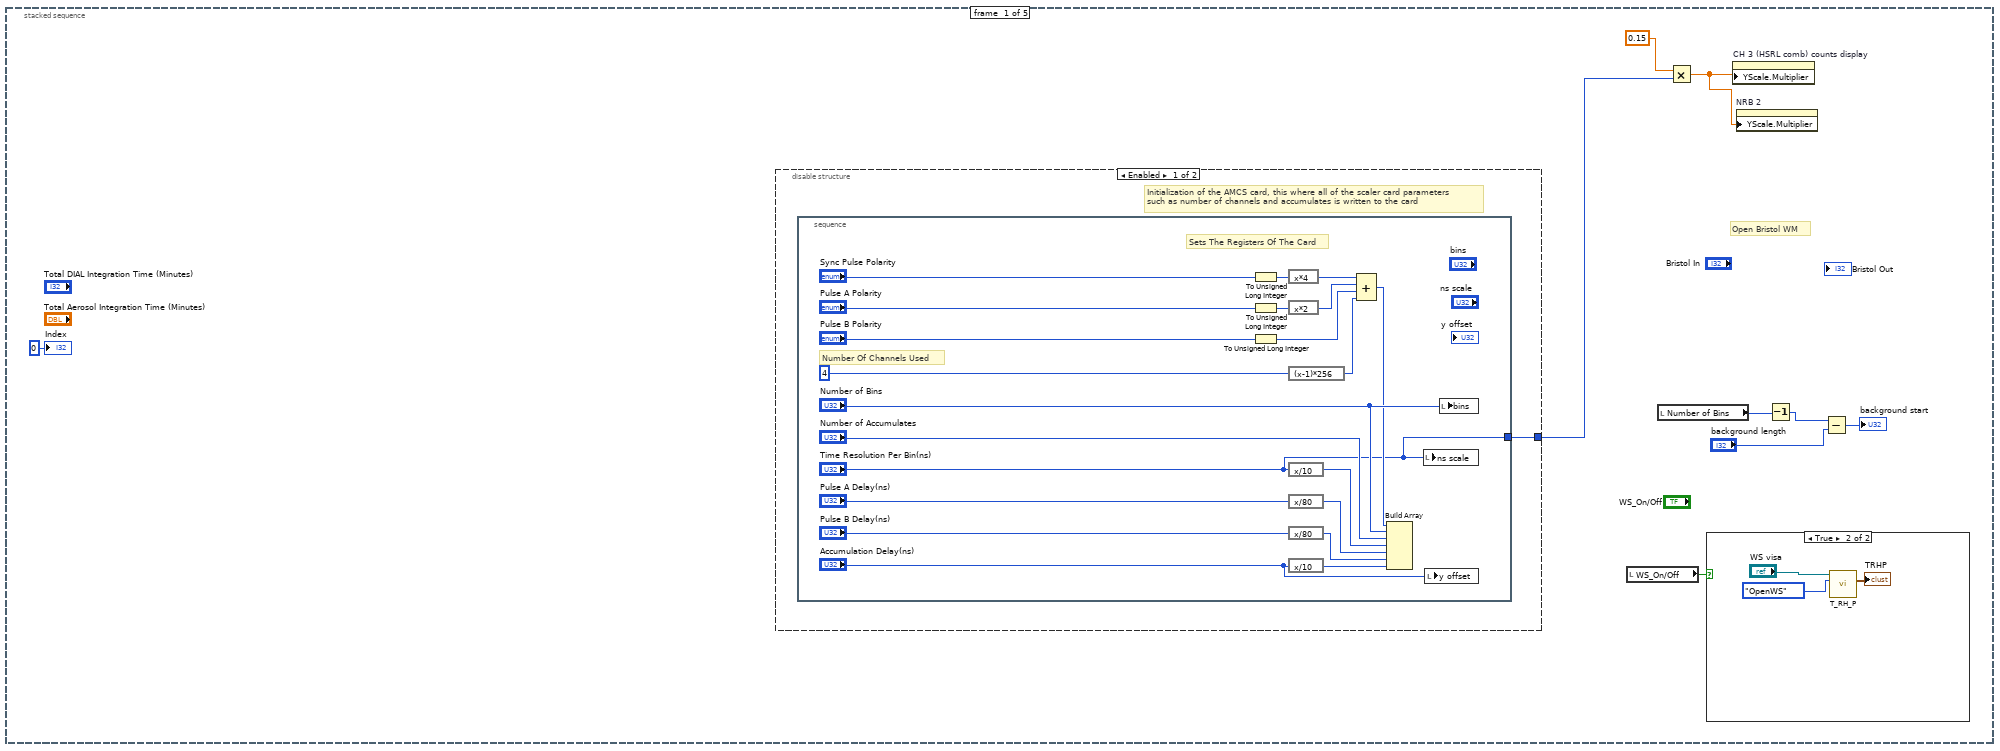
[diagram p4: hidden frame]
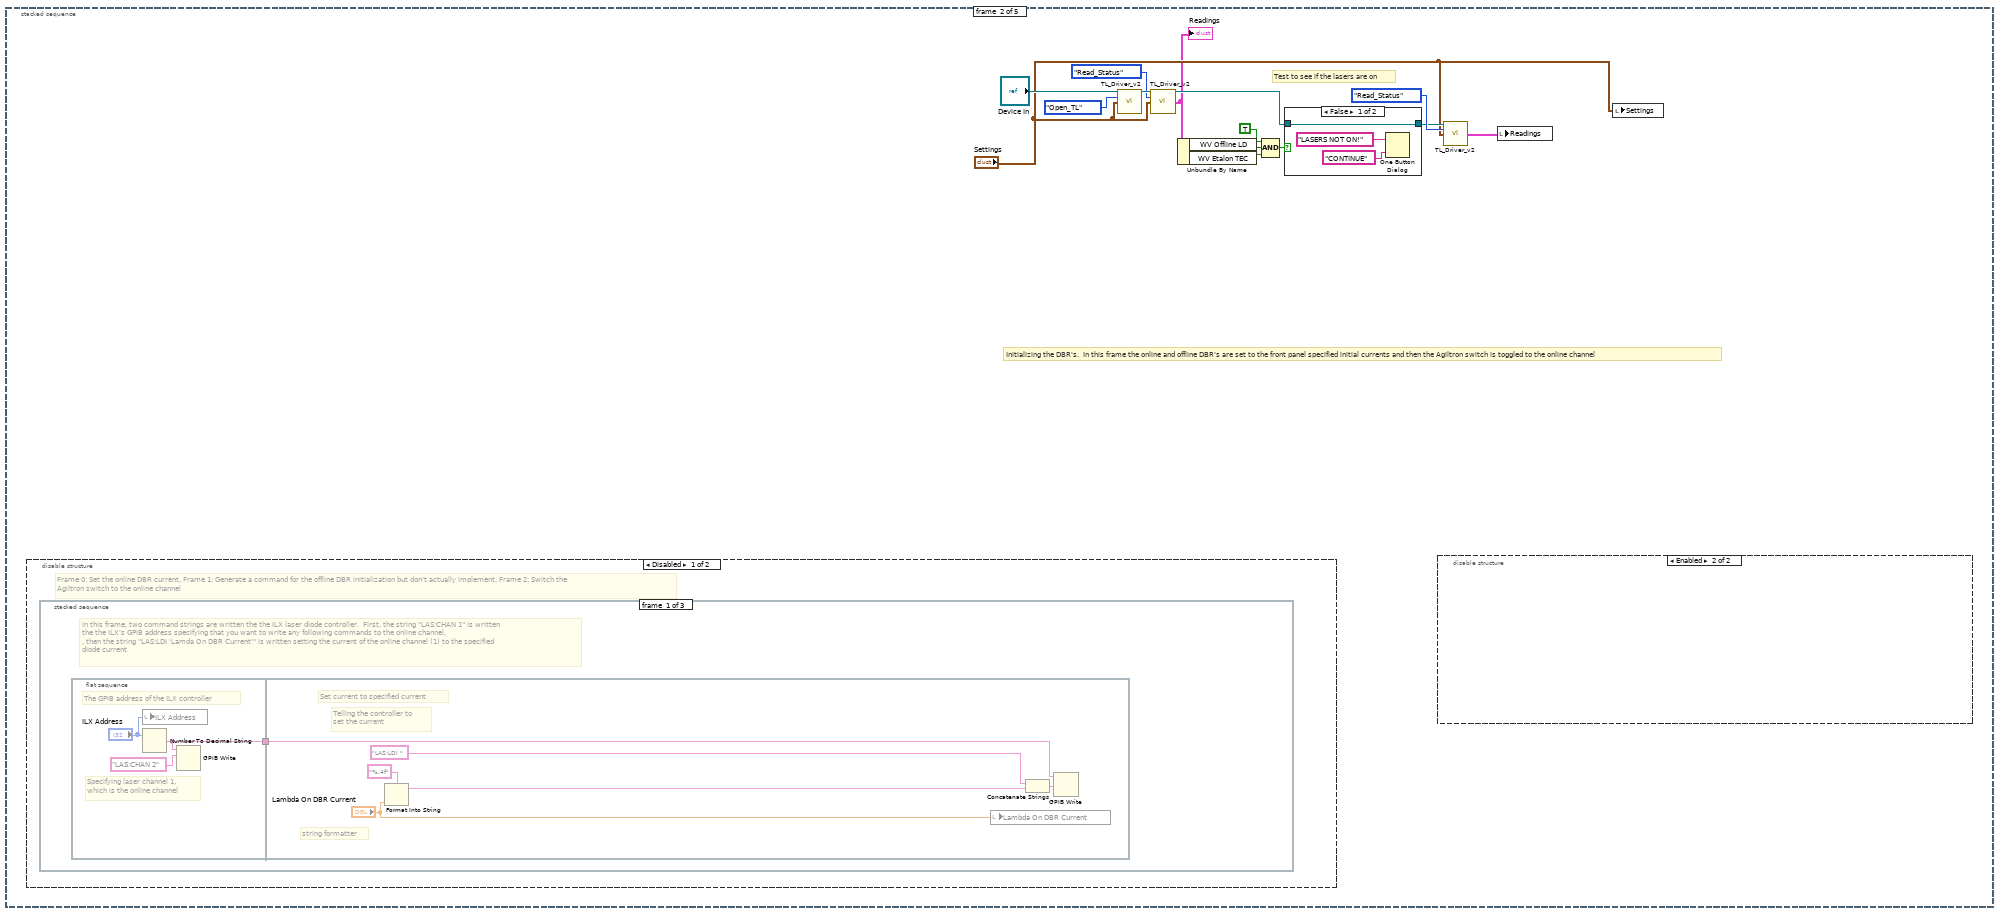
[diagram p7: hidden frame]
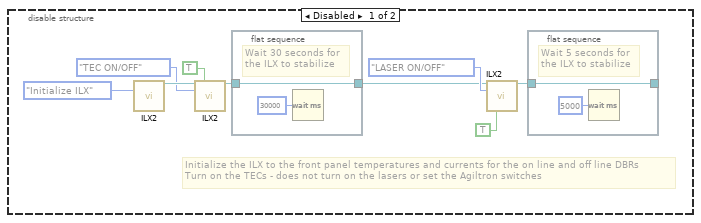
[diagram p9: hidden frame]
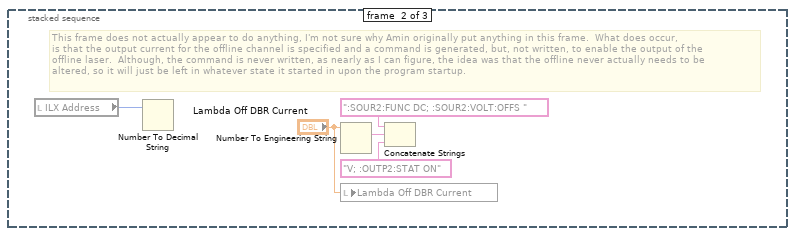
[diagram p10: hidden frame]
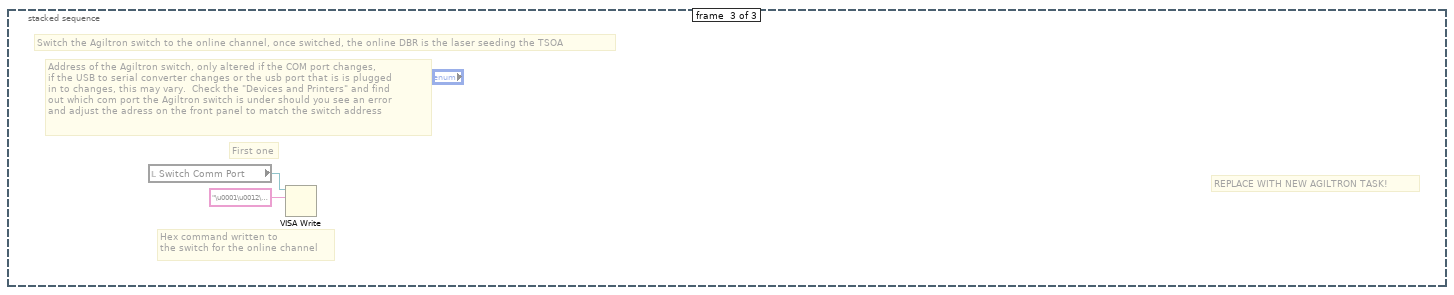
[diagram p11: hidden frame]
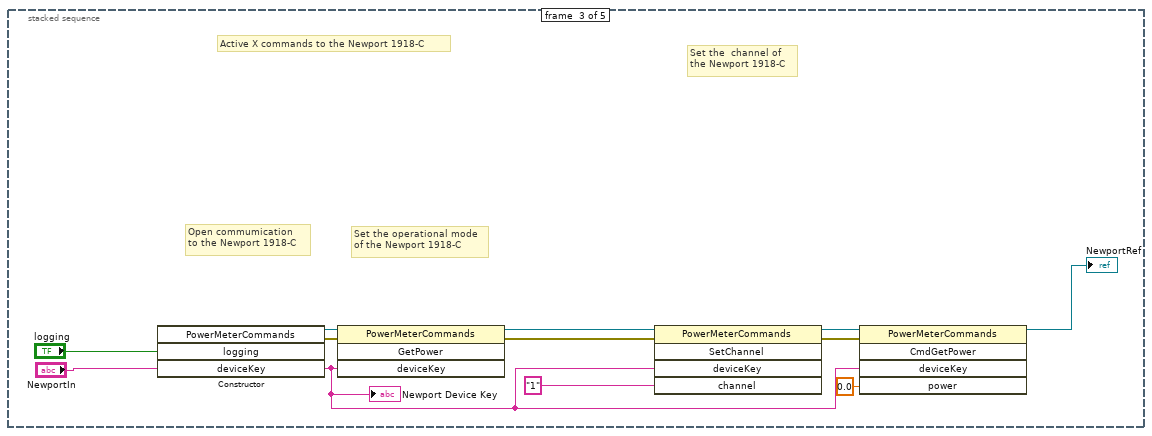
[diagram p13: hidden frame]
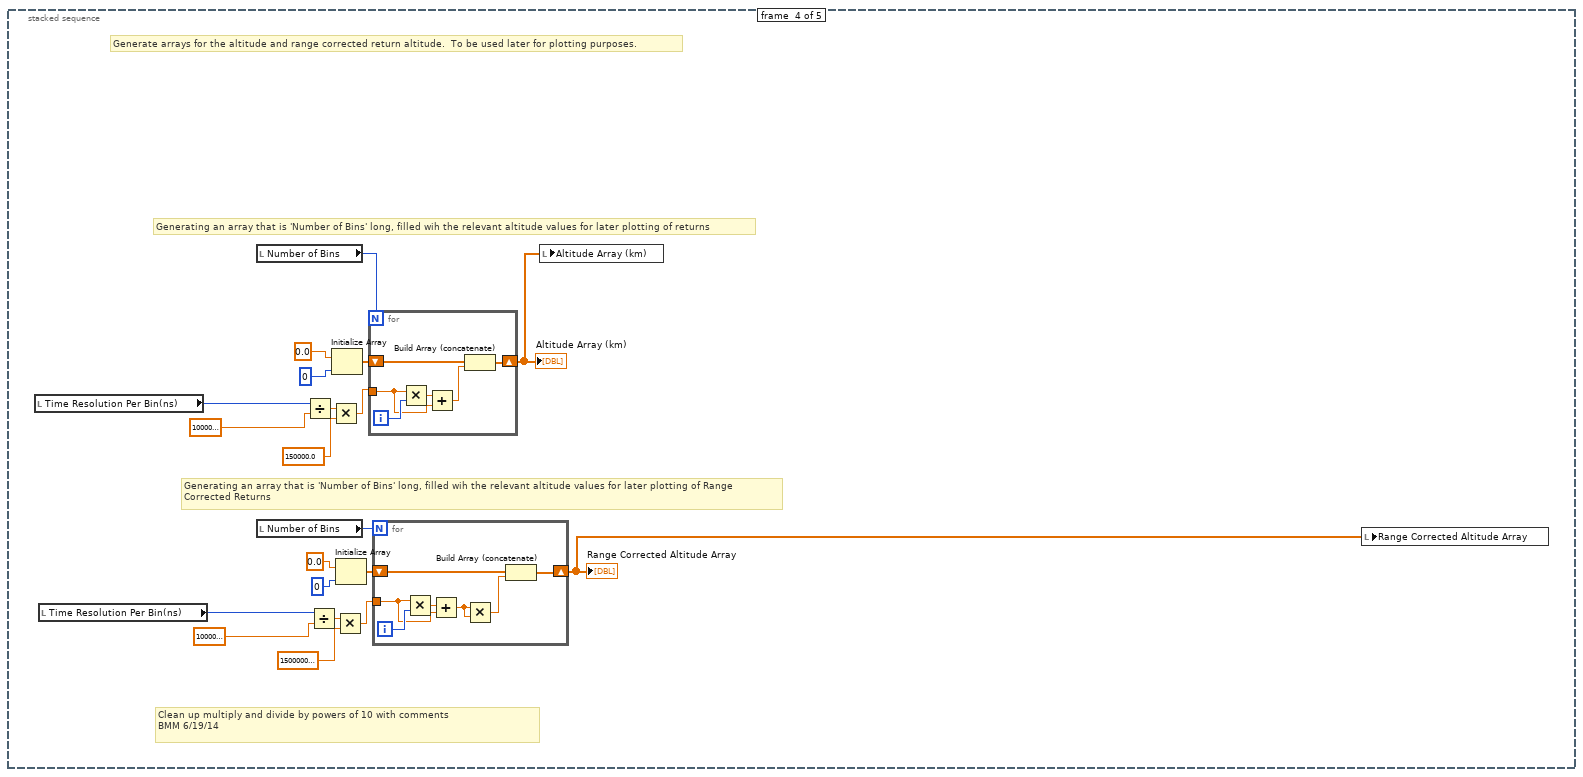
[diagram p14: hidden frame]
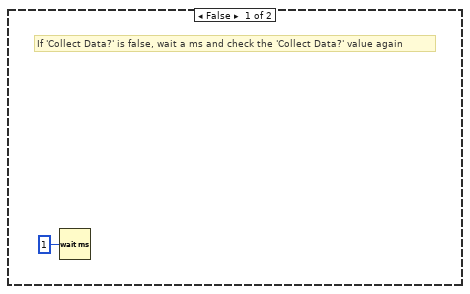
[diagram p15: hidden frame]
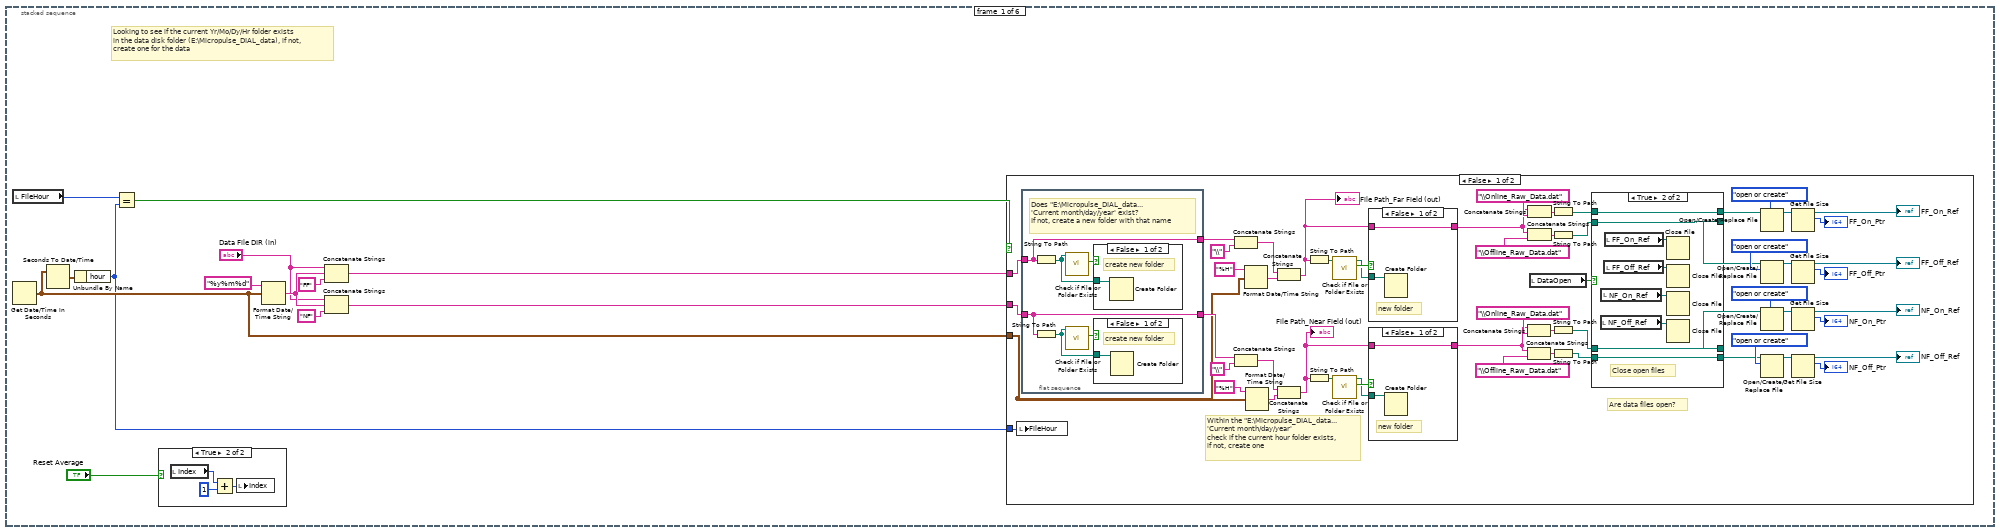
[diagram p16: hidden frame]
diagram:
  # "Frame 0: Initialize the scaler card (and start the MCSC)\nFrame 1: Initialize the DBR's\nFrame 2: Generate address string for talking the to Newport Power meter\nFrame 3: Generate altitude axes for regular and range corrected returns\nFrame 4: Collect data"
  n1 = stacked-sequence {
    tunnel: [_ _ _ _ w131] -> w3
    frame #0 {
      # "Open Bristol WM"
      n2 = disable-structure shown="Enabled" {
        disable-tunnel: [w16 _] -> w5
        frame Enabled {
          # "Initialization of the AMCS card, this where all of the scaler card parameters\nsuch as number of channels and accumulates is written to the card"
          n3 = stacked-sequence {
            tunnel: ["Time Resolution Per Bin(ns)"] -> w16
            frame #0 {
              # "Sets The Registers Of The Card"
              # "Number Of Channels Used"
              n4 = To Unsigned Long Integer(number="Sync Pulse Polarity") -> (unsigned 32bit integer=w18:u32)
              n5 = To Unsigned Long Integer(number="Pulse A Polarity") -> (unsigned 32bit integer=w22:u32)
              n6 = To Unsigned Long Integer(number="Pulse B Polarity") -> (unsigned 32bit integer=w20:u32)
              n7 = expression code="x*4"(w18) -> (w27:u32)
              n8 = expression code="x*2"(w22) -> (w26:u32)
              n9 = expression code="(x-1)*256"(u32 4 ("Number of Channels Used")) -> (w25:u32)
              n10 = expression code="x/10"("Time Resolution Per Bin(ns)") -> (w28:u32)
              n11 = expression code="x/80"("Pulse A Delay(ns)") -> (w35:u32)
              n12 = expression code="x/80"("Pulse B Delay(ns)") -> (w37:u32)
              n13 = expression code="x/10"("Accumulation Delay(ns)") -> (w36:u32)
              n14 = Compound Arithmetic op=ADD(w27, w26, w20, w25) -> (w24:u32)
              n15 = Build Array(w24, "Number of Bins", "Number of Accumulates", w28, w35, w37, w36) -> ()  [unwired: 1 out]
              n16 = local write "ns scale"("Time Resolution Per Bin(ns)") -> ()
              n17 = local write "y offset"("Accumulation Delay(ns)") -> ()
              n18 = local write "bins"("Number of Bins") -> ()
            }
          }
        }
        frame Disabled {
        }
      }
      n19 = local read "WS_On/Off"() -> (w7:bool)
      n20 = local read "Number of Bins"() -> (w11:u32)
      n21 = Multiply(x=0.15, y=w5) -> (x*y=w4:dbl)
      n22 = case shown="True" w7 {
        frame False {
        }
        frame True {
          n23 = call "T_RH_P.vi"("VISA in"="WS visa", "WS_Commands"=enum16{"OpenWS", "ReadTRHP", "CloseWS"}."OpenWS") -> ("TRHP"=→"TRHP":T13)  [unwired: 11 in, 2 out]
        }
      }
      n24 = property on="CH 3 (HSRL comb) counts display" class="IntChart (strict)"("YScale.Multiplier"=w4) -> ()  [unwired: 2 in, 2 out]
      n25 = property on="NRB 2" class="IntChart (strict)"("YScale.Multiplier"=w4) -> ()  [unwired: 2 in, 2 out]
      n26 = Decrement(x=w11) -> (x-1=w10:u32)
      n27 = Subtract(x=w10, y="background length") -> (x-y=→"background start":u32)
      "Index" <- 0 ("Index")
    }
    frame #1 {
      # "Test to see if the lasers are on"
      # "Initializing the DBR's.  In this frame the online and offline DBR's are set to the front panel specified initial currents and then the Agiltron switch is toggled to the online channel"
      n28 = disable-structure shown="Disabled" {
        frame Disabled {
          # "Frame 0: Set the online DBR current, Frame 1: Generate a command for the offline DBR initialization but don't actually implement, Frame 2: Switch the \nAgiltron switch to the online channel"
          n29 = stacked-sequence {
            frame #0 {
              # "In this frame, two command strings are written the the ILX laser diode controller.  First, the string \"LAS:CHAN 1\" is written\nthe the ILX's GPIB address specifying that you want to write any following commands to the online channel,\n, then the string \"LAS:LDI 'Lamda On DBR Current'\" is written setting the current of the online channel (1) to the specified \ndiode current"
              n30 = flat-sequence {
                tunnel: [w71] -> w69
                tunnel: w69 -> [w73]
                frame #0 {
                  # "The GPIB address of the ILX controller"
                  # "Specifying laser channel 1,\nwhich is the online channel"
                  n31 = local write "ILX Address"("ILX Address") -> ()
                  n32 = Number To Decimal String(number="ILX Address") -> (decimal integer string=w71:string)  [unwired: 1 in]
                  n33 = GPIB Write(0:w71, 1:"LAS:CHAN 2") -> ()  [unwired: 3 in, 2 out]
                }
                frame #1 {
                  # "Telling the controller to\nset the current"
                  # "string formatter"
                  # "Set current to specified current"
                  n34 = Format Into String(format string="%.4f" ("Format String"), "Lambda On DBR Current") -> (resulting string=w76:string)  [unwired: 2 in, 1 out]
                  n35 = local write "Lambda On DBR Current"("Lambda On DBR Current") -> ()
                  n36 = Concatenate Strings("LAS:LDI ", w76) -> (w77:string)
                  n37 = GPIB Write(0:w73, 1:w77) -> ()  [unwired: 3 in, 2 out]
                }
              }
            }
            frame #1 {
              # "This frame does not actually appear to do anything, I'm not sure why Amin originally put anything in this frame.  What does occur, \nis that the output current for the offline channel is specified and a command is generated, but, not written, to enable the output of the\noffline laser.  Although, the command is never written, as nearly as I can figure, the idea was that the offline never actually needs to be \naltered, so it will just be left in whatever state it started in upon the program startup."
              n38 = local read "ILX Address"() -> (w79:i32)
              n39 = Number To Decimal String(number=w79) -> ()  [unwired: 1 in, 1 out]
              n40 = Number To Engineering String(4:"Lambda Off DBR Current") -> (0:w83:string)  [unwired: 3 in]
              n41 = local write "Lambda Off DBR Current"("Lambda Off DBR Current") -> ()
              n42 = Concatenate Strings(":SOUR2:FUNC DC; :SOUR2:VOLT:OFFS ", w83, "V; :OUTP2:STAT ON") -> ()  [unwired: 1 out]
            }
            frame #2 {
              # "REPLACE WITH NEW AGILTRON TASK!"
              # "First one"
              # "Address of the Agiltron switch, only altered if the COM port changes,\nif the USB to serial converter changes or the usb port that is is plugged\nin to changes, this may vary.  Check the \"Devices and Printers\" and find \nout which com port the Agiltron switch is under should you see an error \nand adjust the adress on the front panel to match the switch address"
              # "Hex command written to \nthe switch for the online channel"
              # "Switch the Agiltron switch to the online channel, once switched, the online DBR is the laser seeding the TSOA"
              n43 = local read "Switch Comm Port"() -> (w84:refnum<visa-resource-name>)
              n44 = VISA Write(VISA resource name=w84, write buffer="\u0001\u0012\u0000\u0002") -> ()  [unwired: 1 in, 3 out]
            }
          }
        }
        frame Enabled {
        }
      }
      n45 = call "TL_Driver_v2.vi"("Device In"="Device In", "Commands"=T9."Open_TL", "Settings"="Settings") -> ("Device Out"=w49:refnum<visa-resource-name>)  [unwired: 9 in, 3 out]
      n46 = call "TL_Driver_v2.vi"("Device In"=w49, "Commands"=T9."Read_Status", "Settings"="Settings") -> ("Device Out"=w47:refnum<visa-resource-name>, "Readings"=w38:T7)  [unwired: 9 in, 2 out]
      "Readings" <- w38
      n47 = Unbundle By Name(w38) -> ("WV Offline LD"=w42:bool, "WV Etalon TEC"=w43:bool)
      n48 = Compound Arithmetic op=AND(TRUE, w42, w43) -> (w41:bool)
      n49 = case shown="False" w41 {
        tunnel: w47 -> [w52 w55]
        tunnel: [w52 w55] -> w45
        frame False {
          n50 = One Button Dialog(message="LASERS NOT ON!", button name ("OK")="CONTINUE") -> ()  [unwired: 1 out]
        }
        frame True {
        }
      }
      n51 = disable-structure shown="Enabled" {
        frame Disabled {
          # "Initialize the ILX to the front panel temperatures and currents for the on line and off line DBRs\nTurn on the TECs - does not turn on the lasers or set the Agiltron switches"
          n52 = call "ILX2.vi"("ILX Command"=T10."Initialize ILX") -> ("Device Out"=w63:refnum<visa-resource-name>)  [unwired: 10 in, 4 out]
          n53 = call "ILX2.vi"("Device In"=w63, "TEC Control"=TRUE, "ILX Command"=T10."TEC ON/OFF") -> ("Device Out"=w60:refnum<visa-resource-name>)  [unwired: 8 in, 4 out]
          n54 = flat-sequence {
            tunnel: w60 -> [w67]
            tunnel: [w67] -> w57
            frame #0 {
              # "Wait 30 seconds for\nthe ILX to stabilize"
              n55 = Wait (ms)(milliseconds to wait=u32 30000) -> ()  [unwired: 1 out]
            }
          }
          n56 = call "ILX2.vi"("Device In"=w57, "ILX Command"=T10."LASER ON/OFF", "Laser Control"=TRUE ("TEC Control")) -> ("Device Out"=w56:refnum<visa-resource-name>)  [unwired: 8 in, 4 out]
          n57 = flat-sequence {
            tunnel: w56 -> [w65]
            tunnel: [w65] -> _
            frame #0 {
              # "Wait 5 seconds for\nthe ILX to stabilize"
              n58 = Wait (ms)(milliseconds to wait=u32 5000) -> ()  [unwired: 1 out]
            }
          }
        }
        frame Enabled {
        }
      }
      n59 = call "TL_Driver_v2.vi"("Device In"=w45, "Commands"=T9."Read_Status", "Settings"="Settings") -> ("Readings"=w40:T7)  [unwired: 9 in, 3 out]
      n60 = local write "Readings"(w40) -> ()
      n61 = local write "Settings"("Settings") -> ()
    }
    frame #2 {
      # "Active X commands to the Newport 1918-C"
      # "Set the  channel of\nthe Newport 1918-C"
      # "Set the operational mode\nof the Newport 1918-C"
      # "Open commumication\nto the Newport 1918-C"
      n62 = constructor class="PowerMeterCommands"("logging"="logging", "deviceKey"="NewportIn") -> (reference out=w97:refnum<k24>, error out=w94:errorcluster, "deviceKey"=w89:string)  [unwired: 3 in, 2 out]
      "Newport Device Key" <- w89
      n63 = invoke class="PowerMeterCommands" method="GetPower"(reference=w97, error in=w94, "deviceKey"=w89) -> (reference out=w96:refnum<k24>, error out=w93:errorcluster)  [unwired: 1 in, 2 out]
      n64 = invoke class="PowerMeterCommands" method="SetChannel"(reference=w96, error in=w93, "deviceKey"=w89, "channel"="1") -> (reference out=w90:refnum<k24>, error out=w92:errorcluster)  [unwired: 1 in, 3 out]
      n65 = invoke class="PowerMeterCommands" method="CmdGetPower"(reference=w90, error in=w92, "deviceKey"=w89, "power"=sgl 0.0) -> (reference out=→"NewportRef":refnum<k24>)  [unwired: 1 in, 4 out]
    }
    frame #3 {
      # "Clean up multiply and divide by powers of 10 with comments\nBMM 6/19/14"
      # "Generating an array that is 'Number of Bins' long, filled wih the relevant altitude values for later plotting of Range \nCorrected Returns"
      # "Generating an array that is 'Number of Bins' long, filled wih the relevant altitude values for later plotting of returns"
      # "Generate arrays for the altitude and range corrected return altitude.  To be used later for plotting purposes."
      n66 = local read "Time Resolution Per Bin(ns)"() -> (w110:u32)
      n67 = local read "Time Resolution Per Bin(ns)"() -> (w100:u32)
      n68 = local read "Number of Bins"() -> (w113:u32)
      n69 = local read "Number of Bins"() -> (w103:u32)
      n70 = Divide(x=w110, y=1000000000.0) -> (x/y=w108:dbl)
      n71 = Divide(x=w100, y=1000000000.0) -> (x/y=w98:dbl)
      n72 = Multiply(x=w108, y=150000.0) -> (x*y=w111:dbl)
      n73 = Initialize Array(0.0, 0) -> (w116:dbl[])
      n74 = Multiply(x=w98, y=150000000.0) -> (x*y=w101:dbl)
      n75 = Initialize Array(0.0, 0) -> (w106:dbl[])
      n76 = for {
        N: w113 -> [_]
        shift-right: [w129] -> w114
        shift-left: w116 -> [w130]
        tunnel: w111 -> [w126]
        i -> [w128]
        n77 = Multiply(x=w126, y=w128) -> (x*y=w127:dbl)
        n78 = Add(x=w127, y=w126) -> (x+y=w125:dbl)
        n79 = Build Array (concatenate)(w130, w125) -> (w129:dbl[])
      }
      "Altitude Array (km)" <- w114
      n80 = for {
        N: w103 -> [_]
        shift-right: [w123] -> w104
        shift-left: w106 -> [w124]
        tunnel: w101 -> [w119]
        i -> [w122]
        n81 = Multiply(x=w119, y=w122) -> (x*y=w120:dbl)
        n82 = Add(x=w120, y=w119) -> (x+y=w118:dbl)
        n83 = Multiply(x=w118, y=w118) -> (x*y=w121:dbl)
        n84 = Build Array (concatenate)(w124, w121) -> (w123:dbl[])
      }
      "Range Corrected Altitude Array" <- w104
      n85 = local write "Altitude Array (km)"(w114) -> ()
      n86 = local write "Range Corrected Altitude Array"(w104) -> ()
    }
    frame #4 {
      # "Frame 4: Collect data from the scaler card and process and file it"
      n87 = while {
        tunnel: ["stop"] -> w131
        i -> [w132]
        stop <- "stop" stop-if-true
        # "While loop continues data collection cycle"
        n88 = case shown="True" "Collect Data?" {
          frame False {
            # "If 'Collect Data?' is false, wait a ms and check the 'Collect Data?' value again"
            n89 = Wait (ms)(milliseconds to wait=u32 1) -> ()  [unwired: 1 out]
          }
          frame True {
            # "Frame 3: Read the offline wavelength and lock if necessary (code not finished), read output power, read offline data, perform calculations and plot/save offline and NRB data, switch to online\nFrame 4: Calculate the absorption cross section (if wavelength, T, or P changed)\nFrame 5: Calculate Water Vapor Number density and plot"
            # "Frame 0: Create folders and file paths for logging the data, initialize averaging index\nFrame 1: Import current pressure and temperature data from COE weather station\nFrame 2: Read the online wavelength and lock if necessary, read online data and output power\n, plot and save online data, switch to offline DBR"
            # "If 'Collect Data?' is true, collect, process, and log data"
            n90 = stacked-sequence {
              frame #0 {
                # "Looking to see if the current Yr/Mo/Dy/Hr folder exists\nin the data disk folder (E:\\Micropulse_DIAL_data), if not,\ncreate one for the data"
                n91 = local read "FileHour"() -> (w145:i32)
                n92 = Get Date/Time In Seconds() -> (seconds since 1Jan1904=w137:timestamp)
                n93 = Seconds To Date/Time(time stamp (now)=w137) -> (date time rec=w147:T14)  [unwired: 1 in]
                n94 = Unbundle By Name(w147) -> ("hour"=w136:i32)
                n95 = Equal?(x=w145, y=w136) -> (x = y?=w146:bool)
                n96 = case shown="True" "Reset Average" {
                  frame False {
                    n97 = local write "Index"(0 ("Index")) -> ()
                  }
                  frame True {
                    n98 = local read "Index"() -> (w235:i32)
                    n99 = Add(x=w235, y=1) -> (x+y=w234:i32)
                    n100 = local write "Index"(w234) -> ()
                  }
                }
                n101 = Format Date/Time String(time format string (%c)="%y%m%d", seconds (now)=w137) -> (date/time string=w141:string)  [unwired: 1 in]
                n102 = Concatenate Strings("Data File DIR (in)", w141, "FF" ("string")) -> (w143:string)
                n103 = Concatenate Strings("Data File DIR (in)", w141, "NF" ("string")) -> (w138:string)
                n104 = case shown="False" w146 {
                  tunnel: w143 -> [w205 _]
                  tunnel: w138 -> [w204 _]
                  tunnel: w137 -> [w191 _]
                  tunnel: w136 -> [w167 _]
                  frame False {
                    # "Are data files open?"
                    # "Within the \"E:\\Micropulse_DIAL_data...\n'Current month/day/year' \ncheck if the current hour folder exists,\nif not, create one"
                    n105 = local write "FileHour"(w167) -> ()
                    n106 = flat-sequence {
                      tunnel: [w225] -> w192
                      tunnel: w205 -> [w224]
                      tunnel: w204 -> [w225]
                      tunnel: [w224] -> w193
                      frame #0 {
                        # "Does \"E:\\Micropulse_DIAL_data...\n'Current month/day/year' exist?\nIf not, create a new folder with that name"
                        n107 = String To Path(string=w224) -> (path=w229:path)
                        n108 = String To Path(string=w225) -> (path=w227:path)
                        n109 = call <vilib>:"Check if File or Folder Exists.vi"("path"=w229) -> ("file or folder exists?"=w228:bool)  [unwired: 8 in, 2 out]
                        n110 = call <vilib>:"Check if File or Folder Exists.vi"("path"=w227) -> ("file or folder exists?"=w226:bool)  [unwired: 8 in, 2 out]
                        n111 = case shown="False" w228 {
                          tunnel: w229 -> [w231 _]
                          frame False {
                            # "create new folder"
                            n112 = Create Folder(path (use dialog)=w231) -> ()  [unwired: 2 in, 3 out]
                          }
                          frame True {
                            # "Folder exists\ndo nothing"
                          }
                        }
                        n113 = case shown="False" w226 {
                          tunnel: w227 -> [w230 _]
                          frame False {
                            # "create new folder"
                            n114 = Create Folder(path (use dialog)=w230) -> ()  [unwired: 2 in, 3 out]
                          }
                          frame True {
                            # "Folder exists\ndo nothing"
                          }
                        }
                      }
                    }
                    n115 = Concatenate Strings(w193, "\\" ("string")) -> (w200:string)
                    n116 = Concatenate Strings(w192, "\\" ("string")) -> (w195:string)
                    n117 = Format Date/Time String(time format string (%c)="%H", seconds (now)=w191) -> (date/time string=w203:string)  [unwired: 1 in]
                    n118 = Format Date/Time String(time format string (%c)="%H", seconds (now)=w191) -> (date/time string=w198:string)  [unwired: 1 in]
                    n119 = Concatenate Strings(w200, w203) -> (w163:string)
                    "File Path_Far Field (out)" <- w163
                    n120 = Concatenate Strings(w195, w198) -> (w164:string)
                    "File Path_Near Field (out)" <- w164
                    n121 = String To Path(string=w163) -> (path=w201:path)
                    n122 = String To Path(string=w164) -> (path=w196:path)
                    n123 = call <vilib>:"Check if File or Folder Exists.vi"("path"=w201) -> ("file or folder exists?"=w190:bool, "dup path"=w188:path)  [unwired: 8 in, 1 out]
                    n124 = call <vilib>:"Check if File or Folder Exists.vi"("path"=w196) -> ("file or folder exists?"=w189:bool, "dup path"=w187:path)  [unwired: 8 in, 1 out]
                    n125 = case shown="False" w190 {
                      tunnel: w188 -> [w222 _]
                      tunnel: w163 -> [w221 w223]
                      tunnel: [w221 w223] -> w161
                      frame False {
                        # "new folder"
                        n126 = Create Folder(path (use dialog)=w222) -> ()  [unwired: 2 in, 3 out]
                      }
                      frame True {
                        # "Folder exists\ndo nothing"
                      }
                    }
                    n127 = case shown="False" w189 {
                      tunnel: w187 -> [w219 _]
                      tunnel: w164 -> [w218 w220]
                      tunnel: [w218 w220] -> w162
                      frame False {
                        # "new folder"
                        n128 = Create Folder(path (use dialog)=w219) -> ()  [unwired: 2 in, 3 out]
                      }
                      frame True {
                        # "Folder exists\ndo nothing"
                      }
                    }
                    n129 = Concatenate Strings(w162, "\\Online_Raw_Data.dat" ("string")) -> (w181:string)
                    n130 = Concatenate Strings(w162, "\\Offline_Raw_Data.dat" ("string")) -> (w180:string)
                    n131 = Concatenate Strings(w161, "\\Online_Raw_Data.dat" ("string")) -> (w186:string)
                    n132 = Concatenate Strings(w161, "\\Offline_Raw_Data.dat" ("string")) -> (w185:string)
                    n133 = local read "DataOpen"() -> (w178:bool)
                    n134 = String To Path(string=w186) -> (path=w177:path)
                    n135 = String To Path(string=w185) -> (path=w176:path)
                    n136 = String To Path(string=w181) -> (path=w175:path)
                    n137 = String To Path(string=w180) -> (path=w174:path)
                    n138 = case shown="True" w178 {
                      tunnel: w177 -> [w209 w213]
                      tunnel: [w209 w213] -> w171
                      tunnel: w176 -> [w208 w212]
                      tunnel: [w208 w212] -> w170
                      tunnel: w175 -> [w207 w211]
                      tunnel: [w207 w211] -> w169
                      tunnel: [w206 w210] -> w168
                      tunnel: w174 -> [w206 w210]
                      frame False {
                        # "No files open\ndo nothing"
                      }
                      frame True {
                        # "Close open files"
                        n139 = local read "NF_Off_Ref"() -> (w215:refnum<file>)
                        n140 = local read "NF_On_Ref"() -> (w214:refnum<file>)
                        n141 = local read "FF_Off_Ref"() -> (w217:refnum<file>)
                        n142 = local read "FF_On_Ref"() -> (w216:refnum<file>)
                        n143 = Close File(refnum=w216) -> ()  [unwired: 1 in, 2 out]
                        n144 = Close File(refnum=w217) -> ()  [unwired: 1 in, 2 out]
                        n145 = Close File(refnum=w214) -> ()  [unwired: 1 in, 2 out]
                        n146 = Close File(refnum=w215) -> ()  [unwired: 1 in, 2 out]
                      }
                    }
                    n147 = Open/Create/Replace File(file path (use dialog)=w171, operation (0:open)=T11."open or create") -> (refnum out=w157:refnum<file>)  [unwired: 4 in, 2 out]
                    n148 = Open/Create/Replace File(file path (use dialog)=w170, operation (0:open)=T11."open or create") -> (refnum out=w158:refnum<file>)  [unwired: 4 in, 2 out]
                    n149 = Open/Create/Replace File(file path (use dialog)=w169, operation (0:open)=T11."open or create") -> (refnum out=w159:refnum<file>)  [unwired: 4 in, 2 out]
                    n150 = Open/Create/Replace File(file path (use dialog)=w168, operation (0:open)=T11."open or create") -> (refnum out=w160:refnum<file>)  [unwired: 4 in, 2 out]
                    n151 = Get File Size(file=w157) -> (refnum out=→"FF_On_Ref":refnum<file>, size (in bytes)=→"FF_On_Ptr":i64)  [unwired: 1 in, 1 out]
                    n152 = Get File Size(file=w158) -> (refnum out=→"FF_Off_Ref":refnum<file>, size (in bytes)=→"FF_Off_Ptr":i64)  [unwired: 1 in, 1 out]
                    n153 = Get File Size(file=w159) -> (refnum out=→"NF_On_Ref":refnum<file>, size (in bytes)=→"NF_On_Ptr":i64)  [unwired: 1 in, 1 out]
                    n154 = Get File Size(file=w160) -> (refnum out=→"NF_Off_Ref":refnum<file>, size (in bytes)=→"NF_Off_Ptr":i64)  [unwired: 1 in, 1 out]
                  }
                  frame True {
                    # "Don't need to do anything!"
                  }
                }
              }
              frame #1 {
                # "Writing and plotting retrieved\nweather parameters"
                # "Matlab script goes online and retrieves most recent press, temp, and relative humidity data \nfrom the weather station on the roof of Cobleigh"
                # "Importing the current weather conditions from the COE weather station"
                n155 = disable-structure shown="Disabled" {
                  frame Disabled {
                    n156 = script code="%try\n%s=urlread('http://www.coe.montana.edu/ee/weather/mostCurrentCSV.php');\n%amin=textscan(s,'%s %s %s %s %s %s %s %s %s %s %s %s %s');\n%data=amin{1}{2};\n%[test remain]=strtok(data,',');\n%remain=str2num(remain);\n%press=remain(3)./1000;\n%temp=remain(5);\n%RH=remain(7);\n%catch\npress=.850;\ntemp=20;\nRH=40;\n%end"() -> ()  [unwired: 1 in, 4 out]
                  }
                  frame Enabled {
                  }
                }
                n157 = local read "WS_On/Off"() -> (w236:bool)
                n158 = case shown="True" w236 {
                  frame False {
                  }
                  frame True {
                    n159 = local read "WS visa"() -> (w241:refnum<visa-resource-name>)
                    n160 = call "T_RH_P.vi"("VISA in"=w241, "WS_Commands"=enum16{"OpenWS", "ReadTRHP", "CloseWS"}."ReadTRHP") -> ("TRHP"=w237:T13)  [unwired: 11 in, 2 out]
                    n161 = local write "TRHP"(w237) -> ()
                    n162 = Unbundle By Name(w237) -> ("Temp"=→"Temperature (C)":dbl, "RelH"=→"Relative Humdity (%)":dbl, "Press"=→"Pressure (mb)":dbl)
                  }
                }
              }
              frame #2 {
                # "Frame 3: Read, process, and plot online data\nFrame 4:\nFrame 5: Write the data to the folders from Frame 0 of outter sequence"
                # "Frame 0: Read the online wavelength and adjust to locking tolerance if out of range, Switch to offline DBR\nFrame 1: Read the output power from the Newport meter, calculate and plot the output pulse energy\nFrame 2: Wait 'Scalar Wait Time' for buffer to clear other wavelength data"
                # "Online"
                n163 = stacked-sequence {
                  frame #0 {
                    # "Read the online wavelength and continue adjusting the online DBR if outside the wavelength tolerance\nuntil it is within tolerance"
                    n164 = while {
                      i -> [w246]
                      stop <- w243 stop-if-true
                      # "Frame 2: Decrement DBR current if above tolerance\nFrame 3: Increment DBR current if below tolerance"
                      # "Frame 0: Read the current wavelength from the wavemeter\nFrame 1: Calculate the difference between desired and actual wavelength"
                      # "Continue reading and adjusting online DBR current until within locking tolerance"
                      n165 = stacked-sequence {
                        tunnel: w246 -> [w248 _ _ _ _]
                        tunnel: [_ _ w262 _ _] -> w244
                        frame #0 {
                          n166 = Equal To 0?(x=w248) -> (x = 0?=w247:bool)
                          n167 = case shown="True" w247 {
                            frame False {
                            }
                            frame True {
                              # "Set the TSOA switch to\namplify the ABSORBING\nwavelength"
                              n168 = Build Array(FALSE ("Boolean")) -> (w249:bool[])
                              n169 = call-poly <vilib>:"DAQmx Write.vi"("task/channels in"=refnum<k21> "BristolWM", "data"=w249) -> ()  [unwired: 11 in, 3 out]
                            }
                          }
                        }
                        frame #1 {
                          # "Reading the wavelength from the wavemeter"
                          n170 = flat-sequence {
                            tunnel: [w254] -> w253
                            tunnel: w253 -> [w257]
                            tunnel: [w256] -> w252
                            tunnel: w252 -> [w260]
                            frame #0 {
                              n171 = local read "Bristol In"() -> (w255:i32)
                              n172 = dll-call lib="C:/Users/H2ODial/Desktop/Shared Telescope WV DIAL Code/bristol/CLDevIface.dll" fn="CLOpenUSBSerialDevice"("commPort"=w255) -> ("return type"=w254:i32)  [unwired: 4 in, 2 out]
                            }
                            frame #1 {
                              n173 = dll-call lib="C:/Users/H2ODial/Desktop/Shared Telescope WV DIAL Code/bristol/CLDevIface.dll" fn="CLGetLambdaReading"("devHandle"=w257) -> ("return type"=→"WV Online Read (nm)":dbl, "devHandle"=w256:i32)  [unwired: 3 in, 2 out]
                            }
                            frame #2 {
                              n174 = dll-call lib="C:/Users/H2ODial/Desktop/Shared Telescope WV DIAL Code/bristol/CLDevIface.dll" fn="CLCloseDevice"("commPort"=w260) -> ("return type"=w259:i32)  [unwired: 4 in, 2 out]
                              n175 = local write "Bristol Out"(w259) -> ()
                            }
                          }
                        }
                        frame #2 {
                          # "If WL difference is within tolerance, stop looping, and illuminate 'Wavelength Lock Online' indicator"
                          # "Calculating the difference between the actual and desired online wavelength"
                          n176 = local read "WV Online Read (nm)"() -> (w261:dbl)
                          n177 = local read "Online_Tol"() -> (w267:dbl)
                          n178 = Multiply(x=-1.0, y=w267) -> (x*y=w268:dbl)
                          n179 = Subtract(x=w261, y="WV Online Set (nm)") -> (x-y=w263:dbl)
                          "WL_Difference" <- w263
                          n180 = Greater?(x=w263, y=w268) -> (0:w264:bool)
                          n181 = Less?(x=w263, y=w267) -> (x < y?=w265:bool)
                          n182 = And(x=w264, y=w265) -> (x .and. y?=w262:bool)
                          "Wavelength Lock Online" <- w262
                        }
                        frame #3 {
                          # "If the wavelength difference is greater that 0.0002 nm, decrement the \nDBR current by 0.01 mA"
                          n183 = local read "WL_Difference"() -> (w272:dbl)
                          n184 = Greater Or Equal?(x=w272, y="Online_Tol") -> (x >= y?=w271:bool)
                          n185 = case shown="True" w271 {
                            frame False {
                              # "Wavelength difference is not greater than 0.0002 nm, do nothing"
                            }
                            frame True {
                              # "Generating a command string\nto decrement the current"
                              # "WL difference is greater than 0.0002 nm,\ndecrement the DBR current by 0.01 mA"
                              n186 = local read "Settings"() -> (w279:T6)
                              n187 = local read "y"() -> (w274:dbl)
                              n188 = Unbundle By Name(w279) -> ("WV Online TEC"=w278:dbl)
                              n189 = local read "Device In"() -> (w275:refnum<visa-resource-name>)
                              n190 = Subtract(x=w278, y=w274) -> (x-y=w277:dbl)
                              n191 = Bundle By Name(cluster=w279, "WV Online TEC"=w277, "Module"=T12."WV Online TEC") -> (w281:T6)
                              n192 = call "TL_Driver_v2.vi"("Device In"=w275, "Commands"=T9."SET", "Settings"=w281) -> ("Readings"=w280:T7)  [unwired: 9 in, 3 out]
                              n193 = local write "Settings"(w281) -> ()
                              n194 = local write "Readings"(w280) -> ()
                            }
                          }
                        }
                        frame #4 {
                          # "If WL difference is < 0.0002 nm, increment the DBR current"
                          n195 = local read "Online_Tol"() -> (w283:dbl)
                          n196 = local read "WL_Difference"() -> (w286:dbl)
                          n197 = Multiply(x=-1.0, y=w283) -> (x*y=w282:dbl)
                          n198 = Less Or Equal?(x=w286, y=w282) -> (x <= y?=w285:bool)
                          n199 = case shown="True" w285 {
                            frame False {
                              # "WL difference is no <= to -0.0002 nm, do nothing"
                            }
                            frame True {
                              # "WL difference is < -0.0002,\nincrement the DBR current by 0.01 mA"
                              # "Generating a command string\nto decrement the current"
                              n200 = local read "Settings"() -> (w295:T6)
                              n201 = Unbundle By Name(w295) -> ("WV Online TEC"=w292:dbl)
                              n202 = local read "y"() -> (w288:dbl)
                              n203 = local read "Device In"() -> (w289:refnum<visa-resource-name>)
                              n204 = Add(x=w292, y=w288) -> (x+y=w291:dbl)
                              n205 = Bundle By Name(cluster=w295, "WV Online TEC"=w291, "Module"=T12."WV Online TEC") -> (w294:T6)
                              n206 = call "TL_Driver_v2.vi"("Device In"=w289, "Commands"=T9."SET", "Settings"=w294) -> ("Readings"=w293:T7)  [unwired: 9 in, 3 out]
                              n207 = local write "Settings"(w294) -> ()
                              n208 = local write "Readings"(w293) -> ()
                            }
                          }
                        }
                      }
                      n209 = Or(x=w244, y="Cancel online") -> (x .or. y?=w243:bool)
                    }
                  }
                  frame #1 {
                    # "Converting to pulse energy, assumes 5 percent pickoff"
                    # "Reading the Newport Power meter"
                    # "Reading the output power of the laser transmitter from the Newport power meter, once read, convert to corresponding pulse energy and plot"
                    n210 = local read "Newport Device Key"() -> (w300:string)
                    n211 = local read "NewportRef"() -> (w296:refnum<k24>)
                    n212 = disable-structure shown="Disabled" {
                      frame Disabled {
                        # "Plotting the online and offling pulse energies"
                        n213 = local read "Online Pulse Energy"() -> (w311:dbl)
                        n214 = local read "Offline Pulse Energy"() -> (w310:dbl)
                        n215 = Bundle("Online Pulse Energy"=w311, "Offline Pulse Energy"=w310) -> (→"Pulse Energy (Micro Joule)":T15)  [unwired: 1 in]
                      }
                      frame Enabled {
                      }
                    }
                    n216 = Number To Decimal String(number="SampleSize") -> (decimal integer string=w298:string)  [unwired: 1 in]
                    n217 = invoke class="PowerMeterCommands" method="PerformDAQ"(reference=w296, "deviceKey"=w300, "interval"="1", "sampleSize"=w298) -> ("PerformDAQ"=w301:dbl[])  [unwired: 2 in, 5 out]
                    n218 = call-poly <vilib>:"Mean.vi"("X"=w301) -> ("mean"=w299:dbl)  [unwired: 1 out]
                    n219 = Multiply(x=w299, y=1000.0) -> (x*y=w307:dbl)
                    n220 = Divide(x=w307, y=0.05) -> (x/y=w305:dbl)
                    n221 = Divide(x=w305, y=7.0) -> (x/y=→"Online Pulse Energy":dbl)
                  }
                  frame #2 {
                    # "Wait 'Scalar Wait Time' for the next available batch of scalar card data"
                    n222 = local read "AMCS_Profile"() -> (w312:i32)
                    n223 = disable-structure shown="Disabled" {
                      frame Disabled {
                        # "Waiting 'Scalar Wait Time'"
                        n224 = Wait (ms)(milliseconds to wait="Scalar Wait Time") -> ()  [unwired: 1 out]
                      }
                      frame Enabled {
                      }
                    }
                    n225 = while {
                      tunnel: [w319] -> w313
                      tunnel: [w315] -> _
                      tunnel: w312 -> [w315]
                      stop <- w317 stop-if-true
                      n226 = global read "AMCS_Data.vi" "AMCS_Profile"() -> (w319:i32)
                      n227 = Wait (ms)(milliseconds to wait=u32 10) -> ()  [unwired: 1 out]
                      n228 = Equal?(x=w319, y=w315) -> (x = y?=w318:bool)
                      n229 = case shown="False" w318 {
                        tunnel: [TRUE FALSE] -> w317
                        frame False {
                        }
                        frame True {
                        }
                      }
                    }
                    "AMCS_Profile" <- w313
                  }
                  frame #3 {
                    # "convert time per range bin to meters\nand calculate smoothed bins using\nsmoothing range"
                    # "Plotting online cross section and smoothed online data"
                    # "Calculate the bin by bin mean of the data"
                    # "Collect 'Integration Period (Seconds)' number\nof scalar data"
                    # "Reading, processing, and plotting the online data"
                    n230 = local read "Data Reads (number of loops)"() -> (w347:i32)
                    n231 = for {
                      N: w347 -> [_]
                      tunnel: [w368] -> w359 mode=indexing
                      tunnel: [w367] -> w322 mode=indexing
                      # "Scalar Data is retrieved from Global \nVariable that scaler.vi is writing to,"
                      n232 = global read "AMCS_Data.vi" "AMCS_Data"() -> (w371:u16[][])
                      n233 = disable-structure shown="Disabled" {
                        frame Disabled {
                          n234 = global read "Scalar_Data_3.vi" "Scalar Data 3"() -> ()  [unwired: 1 out]
                          n235 = global read "Scalar_Data.vi" "Scalar Data"() -> ()  [unwired: 1 out]
                        }
                        frame Enabled {
                        }
                      }
                      n236 = Index Array(array=w371, index (row) #1=0 ("index (row)"), index (row) #2=2 ("index (row)")) -> (element #1=w368:u16[], element #2=w367:u16[])  [unwired: 2 in]
                    }
                    n237 = Transpose 2D Array(2D array=w359) -> (transposed array=w363:u16[][])
                    n238 = Transpose 2D Array(2D array=w322) -> (transposed array=w345:u16[][])
                    n239 = for {
                      tunnel: w363 -> [w373] mode=indexing
                      tunnel: [w372] -> w364 mode=indexing
                      n240 = call-poly <vilib>:"Mean.vi"("X"=w373) -> ("mean"=w372:dbl)  [unwired: 1 out]
                    }
                    n241 = for {
                      tunnel: w345 -> [w366] mode=indexing
                      tunnel: [w365] -> w346 mode=indexing
                      n242 = call-poly <vilib>:"Mean.vi"("X"=w366) -> ("mean"=w365:dbl)  [unwired: 1 out]
                    }
                    n243 = local read "bins"() -> (w339:u32)
                    n244 = Array Subset(array=w364, index=1 ("dimension size"), length=w339) -> (w351:dbl[])
                    n245 = Array Subset(array=w346, index=1 ("dimension size"), length=w339) -> (w343:dbl[])
                    n246 = local read "background length"() -> (w329:i32)
                    n247 = local read "background start"() -> (w330:u32)
                    n248 = Array Size(array=w351) -> (size(s)=w348:i32)
                    n249 = Array Size(array=w343) -> (size(s)=w340:i32)
                    n250 = Initialize Array(1.0 ("element"), w348) -> (w350:dbl[])
                    n251 = Initialize Array(1.0 ("element"), w340) -> (w342:dbl[])
                    n252 = Multiply(x=w351, y=w350) -> (x*y=w352:dbl[])
                    "CH 0 Bin Readings" <- w352
                    n253 = Multiply(x=w343, y=w342) -> (x*y=w333:dbl[])
                    "CH 2 Bin Readings" <- w333
                    n254 = local read "Total DIAL Integration Time (Minutes)"() -> (w355:i32)
                    n255 = local read "Time Resolution Per Bin(ns)"() -> (w325:u32)
                    n256 = Array Subset(array=w352, index=w330, length=w329) -> (w361:dbl[])
                    n257 = Array Subset(array=w333, index=w330, length=w329) -> (w335:dbl[])
                    n258 = call-poly <vilib>:"Mean.vi"("X"=w361) -> ("mean"=w360:dbl)  [unwired: 1 out]
                    n259 = call-poly <vilib>:"Mean.vi"("X"=w335) -> ("mean"=w336:dbl)  [unwired: 1 out]
                    n260 = Divide(x=w355, y=w347) -> (x/y=w353:dbl)
                    n261 = local read "Index"() -> (w334:i32)
                    n262 = Subtract(x=w352, y=w360) -> (x-y=w357:dbl[])
                    n263 = Subtract(x=w333, y=w336) -> (x-y=w337:dbl[])
                    n264 = To Double Precision Float(number=w325) -> (double precision float=w326:dbl)
                    n265 = Multiply(x=w353, y=60.0) -> (x*y=w331:dbl)
                    n266 = Multiply(x=w326, y=0.15) -> (x*y=w328:dbl)
                    n267 = call "Ring Buffer CH2 rev2.vi"("Index"=w334, "Profiles to Average"=w331, "Input Array"=w337) -> ("AvgArray"=w338:dbl[])  [unwired: 7 in, 1 out]
                    n268 = call "Ring Buffer CH0 rev2.vi"("Index"=w334, "Profiles to Average"=w331, "Input Array"=w357) -> ("AvgArray"=w356:dbl[])  [unwired: 7 in, 1 out]
                    n269 = Divide(x="Smoothing Range", y=w328) -> (x/y=w323:dbl)
                    "Smoothed Bins" <- w323
                    n270 = call "Smooth Arrray.vi"("smooth size"=w323, "Raw Array"=w356) -> ("Smoothed Array"=→"CH0 (WV on) smoothed":dbl[])  [unwired: 9 in]
                    n271 = call "Smooth Arrray.vi"("smooth size"=w323, "Raw Array"=w338) -> ("Smoothed Array"=→"CH2 (molecular) smoothed":dbl[])  [unwired: 9 in]
                    n272 = disable-structure shown="Disabled" {
                      frame Disabled {
                        n273 = script code="format long;\ncounts=sum(Online);\nif counts >=0.5e6\ntime=time;\nelse\ntime=time\nend"() -> ()  [unwired: 3 in, 2 out]
                      }
                      frame Enabled {
                      }
                    }
                  }
                  frame #4 {
                    # "Toggling the Agiltron switch to the offline DBR seed laser"
                    n274 = disable-structure shown="Disabled" {
                      frame Disabled {
                        n275 = flat-sequence {
                          frame #0 {
                            # "Second one"
                            # "Command the switch to switch to position 2\ncorresponding to the offline DBR"
                            # "Hex string command \ncorrespond to offline"
                            n276 = VISA Write(VISA resource name="Switch Comm Port", write buffer="\u0001\u0012\u0000\u0001") -> ()  [unwired: 1 in, 3 out]
                          }
                        }
                      }
                      frame Enabled {
                      }
                    }
                  }
                  frame #5 {
                    # "Save the recently collected online data if 'Save Data?' is true"
                    n277 = case shown="True" "Save Data?" {
                      frame False {
                        # "'Save Data?' is false, do nothing"
                      }
                      frame True {
                        # "'Save Data?' is true, save onfline data to the Data Disk"
                        # "Write only one copy of data at this time"
                        # "Retrieve Julian Date"
                        n278 = local read "Time Resolution Per Bin(ns)"() -> (w383:u32)
                        n279 = local read "Number of Accumulates"() -> (w381:u32)
                        n280 = local read "Number of Bins"() -> (w382:u32)
                        n281 = local read "WV Online Read (nm)"() -> (w377:dbl)
                        n282 = local read "Lambda On DBR Current"() -> (w405:dbl)
                        n283 = local read "CH 2 Bin Readings"() -> (w403:dbl[])
                        n284 = local read "Online Pulse Energy"() -> (w404:dbl)
                        n285 = local read "CH 0 Bin Readings"() -> (w407:dbl[])
                        n286 = To Double Precision Float(number=w383) -> (double precision float=w378:dbl)
                        n287 = To Double Precision Float(number=w382) -> (double precision float=w379:dbl)
                        n288 = To Double Precision Float(number=w381) -> (double precision float=w380:dbl)
                        n289 = call "Julian_Date_2.vi"() -> ("Julian Date"=w406:dbl)  [unwired: 11 in]
                        n290 = Build Array (concatenate)(w406, w377, w405, w404, w378, w379, w380, w407) -> (w398:dbl[])
                        n291 = Build Array (concatenate)(w406, w377, w405, w404, w378, w379, w380, w403) -> (w388:dbl[])
                        n292 = local write "DataOpen"(TRUE ("DataOpen")) -> ()
                        n293 = local read "NF_On_Ref"() -> (w386:refnum<file>)
                        n294 = local read "FF_On_Ref"() -> (w402:refnum<file>)
                        n295 = local read "NF_On_Ptr"() -> (w387:i64)
                        n296 = local read "FF_On_Ptr"() -> (w401:i64)
                        n297 = Set File Position(offset (in bytes) (0)=w401, refnum=w402) -> (refnum out=w399:refnum<file>, error out=w396:errorcluster)  [unwired: 2 in]
                        n298 = Set File Position(offset (in bytes) (0)=w387, refnum=w386) -> (refnum out=w392:refnum<file>, error out=w390:errorcluster)  [unwired: 2 in]
                        n299 = Write to Binary File(file (use dialog)=w392, data=w388, error in=w390, 5:FALSE ("prepend array or string size? (T)")) -> (refnum out=w391:refnum<file>, error out=w389:errorcluster)  [unwired: 2 in, 1 out]
                        n300 = Write to Binary File(file (use dialog)=w399, data=w398, error in=w396, 5:FALSE ("prepend array or string size? (T)")) -> (refnum out=w397:refnum<file>, error out=w395:errorcluster)  [unwired: 2 in, 1 out]
                        n301 = Get File Position(4:w389, 7:w391) -> (2:w385:i64)  [unwired: 2 out]
                        n302 = Get File Position(4:w395, 7:w397) -> (2:w394:i64)  [unwired: 2 out]
                        n303 = local write "NF_On_Ptr"(w385) -> ()
                        n304 = local write "FF_On_Ptr"(w394) -> ()
                      }
                    }
                  }
                }
              }
              frame #3 {
                # "Frame 3: Read offline data, calculate aerosol data, and plot offline and normalized relative backscatter\nFrame 4:\nFrame 5: Save the offline data and related information"
                # "Frame 0: Read the offline wavelength and lock if necessary, Switch to online DBR\nFrame 1: Read the output power from the Newport power meter\nFrame 2: Wait 'Scalar Wait Time' for buffers to clear of online contiminated data"
                # "offline"
                n305 = stacked-sequence {
                  frame #0 {
                    # "Every 60 data collection cycles, read the offline DBR wavelength, and if outside of wavelength tolerance, adjust DBR current until within tolerance"
                    n306 = local read "L_Count"() -> (w409:i32)
                    n307 = Quotient & Remainder(x=w409, y=60.0) -> (x-y*floor(x/y)=w410:dbl)  [unwired: 1 out]
                    n308 = Equal To 0?(x=w410) -> (x = 0?=w408:bool)
                    n309 = case shown="True" w408 {
                      frame False {
                      }
                      frame True {
                        n310 = while {
                          i -> [w415]
                          stop <- w413 stop-if-true
                          # "If WL difference is within tolerance, stop looping, and illuminate 'Wavelength Lock Offline' indicator"
                          # "Frame 2: Decrement DBR current if above tolerance\nFrame 3: Increment DBR current if below tolerance"
                          # "Frame 0: Read the current wavelength from the wavemeter\nFrame 1: Calculate the difference between desired and actual wavelength"
                          # "Continue reading and adjusting offline DBR current until within locking tolerance"
                          n311 = stacked-sequence {
                            tunnel: w415 -> [w417 _ _ _ _]
                            tunnel: [_ _ w431 _ _] -> w412
                            frame #0 {
                              n312 = Equal To 0?(x=w417) -> (x = 0?=w416:bool)
                              n313 = case shown="True" w416 {
                                frame False {
                                }
                                frame True {
                                # "Set the TSOA switch to\namplify the non ABSORBING\nwavelength"
                                n314 = Build Array(TRUE ("Boolean")) -> (w419:bool[])
                                n315 = call-poly <vilib>:"DAQmx Write.vi"("task/channels in"=refnum<k21> "BristolWM", "data"=w419) -> ()  [unwired: 11 in, 3 out]
                                n316 = Wait (ms)(milliseconds to wait=u32 3200) -> ()  [unwired: 1 out]
                                }
                              }
                            }
                            frame #1 {
                              # "Reading the wavelength from the wavemeter"
                              n317 = flat-sequence {
                                tunnel: [w424] -> w423
                                tunnel: w423 -> [w427]
                                tunnel: [w426] -> w422
                                tunnel: w422 -> [w430]
                                frame #0 {
                                n318 = local read "Bristol In"() -> (w425:i32)
                                n319 = dll-call lib="C:/Users/H2ODial/Desktop/Shared Telescope WV DIAL Code/bristol/CLDevIface.dll" fn="CLOpenUSBSerialDevice"("commPort"=w425) -> ("return type"=w424:i32)  [unwired: 4 in, 2 out]
                                }
                                frame #1 {
                                n320 = dll-call lib="C:/Users/H2ODial/Desktop/Shared Telescope WV DIAL Code/bristol/CLDevIface.dll" fn="CLGetLambdaReading"("devHandle"=w427) -> ("return type"=→"WV Offline Read (nm)":dbl, "devHandle"=w426:i32)  [unwired: 3 in, 2 out]
                                }
                                frame #2 {
                                n321 = dll-call lib="C:/Users/H2ODial/Desktop/Shared Telescope WV DIAL Code/bristol/CLDevIface.dll" fn="CLCloseDevice"("commPort"=w430) -> ("return type"=w429:i32)  [unwired: 4 in, 2 out]
                                n322 = local write "Bristol Out"(w429) -> ()
                                }
                              }
                            }
                            frame #2 {
                              # "Calculating the difference between the actual and desired online wavelength"
                              n323 = local read "Offline_Tol"() -> (w433:dbl)
                              n324 = local read "WV Offline Read (nm)"() -> (w439:dbl)
                              n325 = Multiply(x=-1.0, y=w433) -> (x*y=w432:dbl)
                              n326 = Subtract(x=w439, y="WV Offline Set (nm)") -> (x-y=w435:dbl)
                              "WL Difference off" <- w435
                              n327 = Greater?(x=w435, y=w432) -> (0:w436:bool)
                              n328 = Less?(x=w435, y=w433) -> (x < y?=w437:bool)
                              n329 = And(x=w436, y=w437) -> (x .and. y?=w431:bool)
                              "Wavelength Lock Offline" <- w431
                              n330 = case shown="True" w431 {
                                frame False {
                                }
                                frame True {
                                # "Set the TSOA switch to\namplify the ABSORBING\nwavelength"
                                n331 = Build Array(FALSE ("Boolean")) -> (w441:bool[])
                                n332 = call-poly <vilib>:"DAQmx Write.vi"("task/channels in"=refnum<k21> "BristolWM", "data"=w441) -> ()  [unwired: 11 in, 3 out]
                                n333 = Wait (ms)(milliseconds to wait=u32 3200) -> ()  [unwired: 1 out]
                                }
                              }
                            }
                            frame #3 {
                              # "If the wavelength difference is greater that 0.0002 nm, decrement the \nDBR current by 0.01 mA"
                              n334 = local read "WL Difference off"() -> (w446:dbl)
                              n335 = Greater Or Equal?(x=w446, y="Offline_Tol") -> (x >= y?=w445:bool)
                              n336 = case shown="True" w445 {
                                frame False {
                                # "Wavelength difference is not greater than 0.0002 nm, do nothing"
                                }
                                frame True {
                                # "Generating a command string\nto decrement the current"
                                n337 = local read "Settings"() -> (w453:T6)
                                n338 = Unbundle By Name(w453) -> ("WV Offline TEC"=w451:dbl)
                                n339 = Subtract(x=w451, y="y") -> (x-y=w450:dbl)
                                n340 = local read "Device In"() -> (w448:refnum<visa-resource-name>)
                                n341 = Bundle By Name(cluster=w453, "WV Offline TEC"=w450, "Module"=T12."WV Offline TEC") -> (w454:T6)
                                n342 = call "TL_Driver_v2.vi"("Device In"=w448, "Commands"=T9."SET", "Settings"=w454) -> ("Readings"=w455:T7)  [unwired: 9 in, 3 out]
                                n343 = local write "Settings"(w454) -> ()
                                n344 = local write "Readings"(w455) -> ()
                                }
                              }
                            }
                            frame #4 {
                              # "If WL difference is < 0.0002 nm, increment the DBR current"
                              n345 = local read "WL Difference off"() -> (w458:dbl)
                              n346 = Less Or Equal?(x=w458, y=-0.0001) -> (x <= y?=w456:bool)
                              n347 = case shown="True" w456 {
                                frame False {
                                # "WL difference is no <= to -0.0002 nm, do nothing"
                                }
                                frame True {
                                # "Generating a command string\nto decrement the current"
                                # "WL difference is less than 0.0002 nm,\nincrement the DBR current by 0.01 mA"
                                n348 = local read "Settings"() -> (w466:T6)
                                n349 = Unbundle By Name(w466) -> ("WV Offline TEC"=w464:dbl)
                                n350 = local read "y"() -> (w460:dbl)
                                n351 = Add(x=w464, y=w460) -> (x+y=w463:dbl)
                                n352 = local read "Device In"() -> (w461:refnum<visa-resource-name>)
                                n353 = Bundle By Name(cluster=w466, "WV Offline TEC"=w463, "Module"=T12."WV Offline TEC") -> (w467:T6)
                                n354 = call "TL_Driver_v2.vi"("Device In"=w461, "Commands"=T9."SET", "Settings"=w467) -> ("Readings"=w465:T7)  [unwired: 9 in, 3 out]
                                n355 = local write "Settings"(w467) -> ()
                                n356 = local write "Readings"(w465) -> ()
                                }
                              }
                            }
                          }
                          n357 = Or(x=w412, y="Cancel Offline") -> (x .or. y?=w413:bool)
                        }
                      }
                    }
                  }
                  frame #1 {
                    # "Reading the power meter"
                    # "Updating the pulse energy plot"
                    # "Converting to pulse energy"
                    # "Reading the offline output power, converting to pulse energy,  and updating the Pulse energy plot"
                    n358 = local read "SampleSize"() -> (w470:i32)
                    n359 = local read "Newport Device Key"() -> (w471:string)
                    n360 = local read "Online Pulse Energy"() -> (w477:dbl)
                    n361 = local read "Offline Pulse Energy"() -> (w476:dbl)
                    n362 = local read "NewportRef"() -> (w468:refnum<k24>)
                    n363 = Number To Decimal String(number=w470) -> (decimal integer string=w472:string)  [unwired: 1 in]
                    n364 = invoke class="PowerMeterCommands" method="PerformDAQ"(reference=w468, "deviceKey"=w471, "interval"="1", "sampleSize"=w472) -> ("PerformDAQ"=w473:dbl[])  [unwired: 2 in, 5 out]
                    n365 = Bundle("Online Pulse Energy"=w477, "Offline Pulse Energy"=w476) -> (w475:T15)  [unwired: 1 in]
                    n366 = local write "Pulse Energy (Micro Joule)"(w475) -> ()
                    n367 = call-poly <vilib>:"Mean.vi"("X"=w473) -> ("mean"=w469:dbl)  [unwired: 1 out]
                    n368 = Multiply(x=w469, y=1000.0) -> (x*y=w482:dbl)
                    n369 = Divide(x=w482, y=0.05) -> (x/y=w480:dbl)
                    n370 = Divide(x=w480, y=7.0) -> (x/y=→"Offline Pulse Energy":dbl)
                  }
                  frame #2 {
                    # "Added in the ability to interactively control the ThorLab  setting (just etalon temp for now)"
                    # "Wait 'Scalar Wait Time' for buffers to clear of online contiminated offline data"
                    n371 = disable-structure shown="Disabled" {
                      frame Disabled {
                        # "Wait 'Scalar Wait Time'"
                        n372 = local read "Scalar Wait Time"() -> (w492:u32)
                        n373 = Wait (ms)(milliseconds to wait=w492) -> ()  [unwired: 1 out]
                      }
                      frame Enabled {
                      }
                    }
                    n374 = event shown="[1] \"Settings.WV Etalon TEC\": Value Change" {
                      selector: _ -> [_ _]
                      dyn-events: _ -> [_ _]
                      timeout: 1 -> [_ _]
                      event Timeout {
                        n375 = event-data() -> ()  [unwired: 1 in, 2 out]
                      }
                      event "Settings.WV Etalon TEC": Value Change {
                        # "Generating a command string\nto update the etalon"
                        n376 = event-data() -> ()  [unwired: 1 in, 5 out]
                        n377 = local read "Settings"() -> (w489:T6)
                        n378 = Unbundle By Name(w489) -> ("WV Etalon TEC"=w491:dbl)
                        n379 = Bundle By Name(cluster=w489, "WV Etalon TEC"=w491, "Module"=T12."WV Etalon TEC") -> (w487:T6)
                        n380 = call "TL_Driver_v2.vi"("Device In"=refnum<visa-resource-name> "Pro8000", "Commands"=T9."SET", "Settings"=w487) -> ("Readings"=w488:T7)  [unwired: 9 in, 3 out]
                        n381 = local write "Readings"(w488) -> ()
                        n382 = local write "Settings"(w487) -> ()
                      }
                    }
                  }
                  frame #3 {
                    w527 = 1 ("dimension size")
                    w531 = 1
                    # "Read in latest scalar card data from \n'Scalar Data' global variable that \nscaler.vi is writing to, then wait 1 sec\nfor next batch of data"
                    # "Plotting the normalized relative \nbackscatter"
                    # "Calculating the normalized relative backscatter"
                    # "Calculating/Plotting smoothed data,\ncross sections etc."
                    # "Pick off data with\nout header"
                    # "Calculate mean bin by bin mean"
                    # "Reading in 'Integration Period (Seconds)' of data"
                    # "Read the offline data from the scalar card, perform smoothing, calculate normalized relative backscatter, and plot"
                    # "File path in MATLAB script is of old dial is:\nF:\\Micropulse DIAL\\Micropulse DIAL Matlab\\\nFinal Overlap Function.mat')];"
                    # "Collects Data From Card,\nSends It To The Chart,\nAnd Saves A Copy As A\nFile If Option Selected On\nFront Panel"
                    n383 = for {
                      N: "Data Reads (number of loops)" -> [_]
                      tunnel: [w563] -> w495 mode=indexing
                      tunnel: [w562] -> w494 mode=indexing
                      n384 = global read "AMCS_Data.vi" "AMCS_Data"() -> (w564:u16[][])
                      n385 = disable-structure shown="Disabled" {
                        frame Disabled {
                          n386 = global read "Scalar_Data_4.vi" "Scalar Data 4"() -> ()  [unwired: 1 out]
                          n387 = global read "Scalar_Data_2.vi" "Scalar Data 2"() -> ()  [unwired: 1 out]
                        }
                        frame Enabled {
                        }
                      }
                      n388 = Index Array(array=w564, index (row) #1=1 ("index (row)"), index (row) #2=3 ("index (row)")) -> (element #1=w563:u16[], element #2=w562:u16[])  [unwired: 2 in]
                    }
                    n389 = local read "Total DIAL Integration Time (Minutes)"() -> (w552:i32)
                    n390 = Divide(x=w552, y="Data Reads (number of loops)") -> (x/y=w550:dbl)
                    n391 = local read "Total Aerosol Integration Time (Minutes)"() -> (w554:dbl)
                    n392 = local read "background length"() -> (w499:i32)
                    n393 = Multiply(x=w550, y=60.0) -> (x*y=w537:dbl)
                    n394 = local read "background start"() -> (w500:u32)
                    n395 = Transpose 2D Array(2D array=w495) -> (transposed array=w560:u16[][])
                    n396 = Transpose 2D Array(2D array=w494) -> (transposed array=w543:u16[][])
                    n397 = Divide(x=w554, y="Data Reads (number of loops)") -> (x/y=w555:dbl)
                    n398 = for {
                      tunnel: w560 -> [w570] mode=indexing
                      tunnel: [w569] -> w561 mode=indexing
                      tunnel: w543 -> [w568] mode=indexing
                      tunnel: [w567] -> _ mode=indexing
                      tunnel: [w567] -> w540 mode=indexing
                      n399 = call-poly <vilib>:"Mean.vi"("X"=w570) -> ("mean"=w569:dbl)  [unwired: 1 out]
                      n400 = call-poly <vilib>:"Mean.vi"("X"=w568) -> ("mean"=w567:dbl)  [unwired: 1 out]
                    }
                    n401 = local read "bins"() -> (w528:u32)
                    n402 = Multiply(x=w555, y=60.0) -> (x*y=w518:dbl)
                    n403 = Array Subset(array=w540, index=w527, length=w528) -> (w541:dbl[])
                    "CH3 Bin Readings" <- w541
                    n404 = Array Subset(array=w561, index=w527, length=w528) -> (w539:dbl[])
                    "CH1  Bin Readings" <- w539
                    n405 = Array Subset(array=w541, index=w500, length=w499) -> (w542:dbl[])
                    n406 = Array Subset(array=w539, index=w500, length=w499) -> (w559:dbl[])
                    n407 = local read "Smoothed Bins"() -> (w496:dbl)
                    n408 = call-poly <vilib>:"Mean.vi"("X"=w542) -> ("mean"=w506:dbl)  [unwired: 1 out]
                    n409 = call-poly <vilib>:"Mean.vi"("X"=w559) -> ("mean"=w507:dbl)  [unwired: 1 out]
                    n410 = local read "Index"() -> (w517:i32)
                    n411 = Subtract(x=w541, y=w506) -> (x-y=w519:dbl[])
                    n412 = Subtract(x=w539, y=w507) -> (x-y=w535:dbl[])
                    n413 = call "Ring Buffer CH1 long rev2.vi"("Index"=w517, "Profiles to Average"=w537, "Input Array"=w535) -> ("AvgArray"=w557:dbl[], "RingBufferOut"=→"CH1 RingBuffer long":dbl[][])  [unwired: 7 in]
                    n414 = call "Ring Buffer CH1 short rev2.vi"("Index"=w517, "Profiles to Average"=w518, "Input Array"=w535) -> ("AvgArray"=w553:dbl[], "RingBufferOut"=→"CH1 RingBuffer short":dbl[][])  [unwired: 7 in]
                    n415 = call "Ring Buffer CH3 long rev2.vi"("Index"=w517, "Profiles to Average"=w537, "Input Array"=w519) -> ("AvgArray"=w538:dbl[], "RingBufferOut"=→"CH3 RingBuffer long":dbl[][])  [unwired: 7 in]
                    n416 = call "Ring Buffer CH3 short rev2.vi"("Index"=w517, "Profiles to Average"=w518, "Input Array"=w519) -> ("AvgArray"=w515:dbl[], "RingBufferOut"=→"CH3 RingBuffer short":dbl[][])  [unwired: 7 in]
                    n417 = Reshape Array(w535, w527, w528) -> (→"CH 1 (WV off) counts display":dbl[][])
                    n418 = Reshape Array(w519, w527, w528) -> (→"CH 3 (HSRL comb) counts display":dbl[][])
                    n419 = call "Smooth Arrray.vi"("smooth size"=w496, "Raw Array"=w557) -> ("Smoothed Array"=→"CH1 (WV off) smooth S":dbl[])  [unwired: 9 in]
                    n420 = call "Smooth Arrray.vi"("smooth size"=w496, "Raw Array"=w553) -> ("Smoothed Array"=w526:dbl[])  [unwired: 9 in]
                    "CH1 (WV off) smooth L" <- w526
                    n421 = call "Smooth Arrray.vi"("smooth size"=w496, "Raw Array"=w538) -> ("Smoothed Array"=→"CH3 (HSRL combined) smooth L":dbl[])  [unwired: 9 in]
                    n422 = call "Smooth Arrray.vi"("smooth size"=w496, "Raw Array"=w515) -> ("Smoothed Array"=w498:dbl[])  [unwired: 9 in]
                    "CH3 (HSRL combined) smooth S" <- w498
                    n423 = local read "Time Resolution Per Bin(ns)"() -> (w493:u32)
                    n424 = local read "Number of Accumulates"() -> (w502:u32)
                    n425 = local read "Temperature (C)"() -> (w549:dbl)
                    n426 = local read "Pressure (mb)"() -> (w548:dbl)
                    n427 = script code="%accum_num=10000;     % scaler card setting number of accumulations\nt_bin = t_bin/1e9                 % scaler card setting time per bin\n%t_d = 37.3e-9;                % APD dead time from spec sheet\n\n% conversion from accumulated counts to count rate  (c/s)\nc_convert = 1./t_bin./accum_num;\nCR_far = p_raw_far.*c_convert;\nCR_near = p_raw_near.*c_convert;\nCR_total_far = (p_raw_far+b_far).*c_convert;\nCR_total_near = (p_raw_near+b_near).*c_convert;\nb_CR_far =b_far.*c_convert;\nb_CR_near =b_near.*c_convert;\n \n% create a range array\nsize_p =  size(p_raw_far,2);\ngate = t_bin*3e8/2;\nr = (gate:gate:size_p*gate)./1e3; \n   \n%APD correction factor\n D_far = 1./(1-(t_d*CR_total_far));\n D_near = 1./(1-(t_d*CR_total_near));\n\n %Calculating normalize relative backscatter profile\n nrb_far = CR_far.*D_far.*r.^2.*1e-6;\n nrb_near = CR_near.*D_near.*r.^2.*1e-6;"("E"=6.0 ("Real"), "temp"=w549, "press"=w548, "p_raw_far"=w526, "b_far"=w507, "b_near"=w506, "p_raw_near"=w498, "accum_num"=w502, "t_d"="dead time", "t_bin"=w493) -> ("nrb_far"=w521:cdb[], "D_far"=w512:dbl[], "nrb_near"=w520:cdb[], "D_near"=w511:dbl[], "b_CR_far"=w504:dbl, "b_CR_near"=w503:dbl)  [unwired: 1 in, 1 out]
                    n428 = local read "bins"() -> (w530:u32)
                    n429 = local read "Altitude Array (km)"() -> (w523:dbl[])
                    n430 = Bundle(w504, w503) -> (→"?":cluster{dbl, dbl})  [unwired: 1 in]
                    n431 = Build Array(w521, w520) -> (w525:cdb[][])
                    n432 = Build Array(w512, w511) -> (w510:dbl[][])
                    n433 = Reshape Array(w520, w531, w530) -> (→"NRB 2":cdb[][])
                    n434 = Reshape Array(w521, w531, w530) -> (→"NRB":cdb[][])
                    n435 = Build Array(w523, w523) -> (w522:dbl[][])
                    n436 = call "Convert to Dynamic Data7"("2D Array"=w510) -> ("Dynamic Data Type"=w509:dynamicdata)  [unwired: 3 in]
                    n437 = call "Convert to Dynamic Data3"("2D Array"=w525) -> ("Dynamic Data Type"=w524:dynamicdata)  [unwired: 3 in]
                    n438 = call "Convert to Dynamic Data4"("2D Array"=w522) -> ("Dynamic Data Type"=w513:dynamicdata)  [unwired: 3 in]
                    n439 = call "Build XY Graph2"("Y Input"=w513, "X Input"=w524) -> ("XY Graph"=→"NRB plot":cluster{"Y":dbl[], "Y":dbl[]}[])  [unwired: 3 in, 6 out]
                    n440 = call "Build XY Graph4"("Y Input"=w513, "X Input"=w509) -> ("XY Graph"=→"Correction":cluster{"Y":dbl[], "Y":dbl[]}[])  [unwired: 3 in, 6 out]
                  }
                  frame #4 {
                    # "REPLACE WITH NEW AGILTRON TASK!"
                    # "Toggle Agiltron switch to online DBR"
                    n441 = disable-structure shown="Disabled" {
                      frame Disabled {
                        # "ABSORBING"
                        n442 = flat-sequence {
                          frame #0 {
                            # "Third one"
                            # "Command the switch to switch to position 1\ncorresponding to the online DBR"
                            # "Hex string command \ncorrespond to online"
                            n443 = local read "Switch Comm Port"() -> (w574:refnum<visa-resource-name>)
                            n444 = VISA Write(VISA resource name=w574, write buffer="\u0001\u0012\u0000\u0002") -> ()  [unwired: 1 in, 3 out]
                          }
                        }
                        n445 = Build Array(FALSE ("Boolean")) -> (w573:bool[])
                        n446 = call-poly <vilib>:"DAQmx Write.vi"("task/channels in"=refnum<k21> "AgiltronSwitch", "data"=w573) -> ()  [unwired: 11 in, 3 out]
                      }
                      frame Enabled {
                      }
                    }
                  }
                  frame #5 {
                    # "If 'Save Data?' is true, save all relavant offline info"
                    n447 = local read "Save Data?"() -> (w576:bool)
                    n448 = case shown="True" w576 {
                      frame False {
                        # "'Save Data?' is false, do nothing"
                      }
                      frame True {
                        # "Write only one data file at this time"
                        # "Retrive Julian Date"
                        # "'Save Data?' is true, save offline data to the Data Disk"
                        n449 = local read "Lambda Off DBR Current"() -> (w598:dbl)
                        n450 = local read "WV Offline Read (nm)"() -> (w597:dbl)
                        n451 = local read "Relative Humdity (%)"() -> (w602:dbl)
                        n452 = local read "CH3 Bin Readings"() -> (w595:dbl[])
                        n453 = local read "CH1  Bin Readings"() -> (w603:dbl[])
                        n454 = local read "Offline Pulse Energy"() -> (w599:dbl)
                        n455 = local read "Temperature (C)"() -> (w600:dbl)
                        n456 = local read "Pressure (mb)"() -> (w601:dbl)
                        n457 = call "Julian_Date_2.vi"() -> ("Julian Date"=w596:dbl)  [unwired: 11 in]
                        n458 = Build Array (concatenate)(w596, w597, w598, w599, w600, w601, w602, w603) -> (w581:dbl[])
                        n459 = Build Array (concatenate)(w596, w597, w598, w599, w600, w601, w602, w595) -> (w578:dbl[])
                        n460 = local read "FF_Off_Ref"() -> (w583:refnum<file>)
                        n461 = local read "NF_Off_Ref"() -> (w580:refnum<file>)
                        n462 = local read "FF_Off_Ptr"() -> (w582:i64)
                        n463 = local read "NF_Off_Ptr"() -> (w579:i64)
                        n464 = Set File Position(offset (in bytes) (0)=w582, refnum=w583) -> (refnum out=w594:refnum<file>, error out=w592:errorcluster)  [unwired: 2 in]
                        n465 = Set File Position(offset (in bytes) (0)=w579, refnum=w580) -> (refnum out=w590:refnum<file>, error out=w588:errorcluster)  [unwired: 2 in]
                        n466 = Write to Binary File(file (use dialog)=w594, data=w581, error in=w592, 5:FALSE ("prepend array or string size? (T)")) -> (refnum out=w593:refnum<file>, error out=w591:errorcluster)  [unwired: 2 in, 1 out]
                        n467 = Write to Binary File(file (use dialog)=w590, data=w578, error in=w588, 5:FALSE ("prepend array or string size? (T)")) -> (refnum out=w589:refnum<file>, error out=w587:errorcluster)  [unwired: 2 in, 1 out]
                        n468 = Get File Position(4:w591, 7:w593) -> (2:w584:i64)  [unwired: 2 out]
                        n469 = Get File Position(4:w587, 7:w589) -> (2:w577:i64)  [unwired: 2 out]
                        n470 = local write "FF_Off_Ptr"(w584) -> ()
                        n471 = local write "NF_Off_Ptr"(w577) -> ()
                      }
                    }
                  }
                }
              }
              frame #4 {
                n472 = First Call?() -> (First Call?: T/F=w606:bool)
                n473 = Or(x="calculate absorption cross sections", y=w606) -> (x .or. y?=w604:bool)
                n474 = case shown="True" w604 {
                  frame False {
                  }
                  frame True {
                    # "calculate absorption cross sections from HITRAN data base"
                  }
                }
              }
              frame #5 {
                # "Data Processing Far Channel"
                # "Calculating the range resolved water vapor number density and plotting"
              }
            }
          }
        }
        "L_Count" <- w132
      }
    }
  }
  n475 = case shown="True" w3 {
    frame False {
    }
    frame True {
      # "close data files"
      n476 = local read "NF_Off_Ref"() -> (w608:refnum<file>)
      n477 = local read "NF_On_Ref"() -> (w609:refnum<file>)
      n478 = local read "FF_Off_Ref"() -> (w610:refnum<file>)
      n479 = local read "FF_On_Ref"() -> (w611:refnum<file>)
      n480 = local read "WS_On/Off"() -> (w607:bool)
      n481 = case shown="True" w607 {
        frame False {
        }
        frame True {
          n482 = local read "WS visa"() -> (w612:refnum<visa-resource-name>)
          n483 = call "T_RH_P.vi"("VISA in"=w612, "WS_Commands"=enum16{"OpenWS", "ReadTRHP", "CloseWS"}."CloseWS") -> ()  [unwired: 11 in, 3 out]
        }
      }
      n484 = Close File(refnum=w611) -> ()  [unwired: 1 in, 2 out]
      n485 = Close File(refnum=w610) -> ()  [unwired: 1 in, 2 out]
      n486 = Close File(refnum=w609) -> ()  [unwired: 1 in, 2 out]
      n487 = Close File(refnum=w608) -> ()  [unwired: 1 in, 2 out]
    }
  }
  "FileHour" <- -1 ("FileHour")
  "DataOpen" <- FALSE
